vi "TestBoxStart.vi"() -> ()   [LabVIEW 2019]
uses:
  QCtests/general_VIs/globals/QC_MeasurementSetup.vi
  InstrControl/InstrumentSetup.vi
  <instrlib>/ke7002/KE7002.LLB/Keith 7002 Open/Close Chan.vi
  <instrlib>/Agilent 34401/Public/Data/Read (Single Point).vi
  <vilib>/regexp/Match Regular Expression.xnode
  InstrControl/SupplyControl/SupplyControl.lvclass
  InstrControl/LCRControl/LCRControl.lvclass
  InstrControl/InstrControl.lvclass
  InstrControl/ArduinoControl/ArduinoControl.lvclass
  <instrlib>/Agilent 34401/Agilent 34401.lvlib
panel:
  out "Data Path":path
  out "Monitor Start \nTime":dbl=10.0 format="%<%I:%M:%S %p>T"
  out "LCS Data":cluster{dbl[], dbl[], dbl[], dbl[], dbl[]}[](array[cluster])
  out "CV Test CH":i32
  out "CV Data":cluster{dbl[], dbl[], dbl[], dbl[], dbl[]}[](array[cluster])
  out "Time":u32[](array[numeric])
  out "Temperature Array":dbl[](array[numeric])
  out "Humidity Array":dbl[](array[numeric])
  out "IV Data":cluster{dbl[], dbl[], dbl[], dbl[], dbl[]}[](array[cluster])
  out "IV Test CH":i32
  out "Run time":u32 format="%<%H:%M:%S>t"
  out "RH [%]":dbl=10.0
  out "Temp. [°C]":dbl=10.0
  in  "Abort Test":bool
  out "TGraph":cluster{u32[], dbl[]}[](graph)
  in  "Test Control":T1(tab)
  in  "SID 7":string
  in  "LCS Test":bool
  in  "CV Test":bool
  in  "IV Test":bool
  out "T/RH":enum16{"Read Arduino"}(ring)
  in  "Institute:":string(combo)="TRIUMF"
  out "Volt:":string="Aglient 34401A"
  out "LCR:":string="WayneKerr 6440B"
  in  "Quit":bool
  in  "Continue":bool
  in  "Mesurement Control":enum32{"IV Setup", "CV Setup", "LCS Setup"}(tab)
  in  "Cofigure IV Test":bool
  in  "IV Breakdown Limit [V]":dbl=-500.0 caption="Breakdown Limit [V]"
  in  "Step Interval [s] IN":i32=10 caption="step interval [s]"
  in  "Step [V] IN":dbl=10.0 caption="step [V]" format="%.1f"
  in  "IV_Final Volts [V] IN":dbl=-700.0 caption="Final volts [V]"
  in  "IV_Initial Volts [V] IN":dbl caption="Initial volts [V]"
  in  "hold steps IN":i32=6 caption="hold steps"
  in  "IV Current Limit [µA]":dbl=1000.0 caption="Current Limit [µA]" min=0.0001 format="%.3f"
  in  "CV Current Limit [µA]":dbl=15.0 caption="Current Limit [µA]" min=0.0001 format="%.3f"
  in  "CV_depletion limit [V] IN":dbl=-300.0 caption="Depletion Limit [V]"
  in  "CV Frequency [Hz] IN":i32=5000 caption="Frequency [Hz]" format="%#.3p"
  in  "CV_step interval [s] IN":i32=16 caption="Step Interval [s]"
  in  "CV step [V] IN":dbl=10.0 caption="Step [V]" format="%.1f"
  in  "CV_Final volts [V] IN":dbl=-500.0 caption="Final Voltage [V]"
  in  "CV Initial volts [V] IN":dbl caption="Initial Voltage [V]"
  in  "Configure CV Test":bool
  in  "LCS Norm. to Temp. [°C]":dbl=22.0 caption="Norm. to Temp. [°C]"
  in  "LCS Step Interval [s] IN":i32 caption="Step Interval [s]"
  in  "Configure LCS Test":bool
  in  "LCS Current Limit [µA]":dbl=1000.0 caption="Current Limit [µA]" min=0.0001 format="%.3f"
  in  "LCS Step Size [V] IN":dbl caption="Step Size [V]"
  in  "LCS Test Volts [V] IN":dbl=-700.0 caption="Test Voltage [V]"
  in  "LCS Test Duration IN":i32=10 caption="Test Length [HH:MM:SS]" format="%<%H:%M:%S>t"
  in  "LCS Measurement Interval [s] IN":i32=10 caption="Measurement Interval [s]"
  out "SMU:":string="Keithley 2410"
  in  "User:":string(combo)="Graham"
  in  "SID 24":string
  in  "SID 23":string
  in  "SID 22":string
  in  "SID 21":string
  in  "SID 20":string
  in  "SID 19":string
  in  "SID 18":string
  in  "SID 17":string
  in  "SID 16":string
  in  "SID 15":string
  in  "SID 14":string
  in  "SID 13":string
  in  "SID 12":string
  in  "SID 11":string
  in  "SID 10":string
  in  "SID 9":string
  in  "SID 8":string
  in  "SID 6":string
  in  "SID 5":string
  in  "SID 4":string
  in  "SID 3":string
  in  "SID 2":string
  in  "SID 1":string
  in  "IV Scales":T2(ring) caption="Plot Scale"
  out "IV Volts":dbl[](array[numeric]) caption="Volts [V]"
  out "IV Current":dbl[](array[numeric]) caption="Current [nA]"
  in  "IV Iscale":enum16{"nanoAmps", "microAmps", "milliAmps"}(ring) caption="Y Axis Scale"
  out "IV Test Channel:":string caption="Test Channel:"
  out "IV step interval [s]":i32=10 caption="step interval [s]"
  out "IV step [V]":dbl=10.0 caption="Step Size [V]" format="%.1f"
  out "IV Final volts [V]":dbl=-700.0 caption="Final Voltage [V]" format="%.1f"
  out "IV Initial volts [V]":dbl caption="Initial Voltage [V]" format="%.1f"
  out "IV hold steps":i32 caption="Hold Steps"
  out "IV STATUS":string
  out "IV Last reading at:":string caption="Last reading at:"
  out "IV Current reading No.":u32
  out "No of steps":u32
  out "IV Bias On/Off:":bool caption="Bias On/Off:"
  out "IV Current Volts:":dbl caption="Current Volts:" format="%.2f"
  out "IV Time Initiated:":string caption="Time Initiated:"
  out "IV Sensor No.:":string caption="Sensor No.:"
  out "IV Graph":cluster{dbl[], dbl[]}[](graph)
  out "CV Graph":cluster{dbl[], dbl[]}[](graph)
  in  "Cscale":enum16{"1/C^2 [1/nF^2]", "nF", "pF"}(ring) caption="Y Axis Scale"
  out "CV Sensor No.:":string caption="Sensor No.:"
  out "CV Time Initiated:":string caption="Time Initiated:"
  out "CV Current Volts:":dbl caption="Current Volts:" format="%.2f"
  out "CV Bias On/Off:":bool caption="Bias On/Off:"
  out "CV No of steps":u32
  out "CV Current reading No.":u32
  out "CV Last reading at:":string caption="Last reading at:"
  out "CV STATUS":string
  out "CV Test Channel:":string caption="Test Channel:"
  in  "CV Scales":T2(ring) caption="Plot Scale"
  out "CV Capacitance":dbl[](array[numeric]) caption="C [pF]"
  out "CV Resistance":dbl[](array[numeric]) caption="R [kOhm]"
  out "CV Volts":dbl[](array[numeric]) caption="V [V]"
  out "Frequency [Hz]":i32=1000 format="%#.3p"
  out "CV step interval [s]":u32=5 caption="Step Interval [s]"
  out "CV step [V]":dbl=10.0 caption="Step Size [V]" format="%.1f"
  out "CV Final volts [V]":dbl=-700.0 caption="Final Voltage [V]" format="%.1f"
  out "CV Initial volts [V]":dbl caption="Initial Voltage [V]" format="%.1f"
  out "Norm. to Temp. [°C]":dbl=20.0
  out "Number of Sensors":i32=10 caption="No. of Sensors"
  out "LCS Measurement Interval":i32=10 caption="Interval [s["
  out "LCS Test Duration":i32=10 caption="Test Length" format="%<%H:%M:%S>t"
  out "LCS Test Volts [V]":dbl=-700.0 caption="Test Voltage [V]"
  out "Time Remaining":u32 format="%<%H:%M:%S>t"
  out "Time Elapsed":u32 format="%<%H:%M:%S>t"
  out "LCS No of steps":u32
  out "LCS Time Initiated:":string caption="Time Initiated:"
  out "LCS Test Channel:":string caption="Test Channel:"
  out "LCS Sensor No.:":string caption="Sensor No.:"
  out "LCS Current reading No.":u32
  out "LCS Last reading at:":string caption="Last reading at:"
  out "LCS Bias On/Off:":bool caption="Bias On/Off:"
  out "LCS Current Volts:":dbl caption="Current Volts:" format="%.2f"
  in  "LCS Scales":T2(ring) caption="Plot Scale"
  in  "LCS Iscale":enum16{"nanoAmps", "microAmps", "milliAmps"}(ring) caption="Y Axis Scale"
  out "LCS Graph":cluster{dbl[], dbl[]}[](graph)
  out "LCS STATUS":string
  in  "Write Comments":bool
  out "Current Text":string
  in  "End Program":bool
  in  "Comment Box":string
  out "Stability":bool[](array[boolean])
  out "CV":bool[](array[boolean])
  out "IV":bool[](array[boolean])
  in  "Channel":u16(ring)=24 items=["CH 1", "CH 2", "CH 3", "CH 4", "CH 5", "CH 6", "CH 7", "CH 8", "CH 9", "CH 10", "CH 11", "CH 12", "CH 13", "CH 14", "CH 15", "CH 16", "CH 17", "CH 18", "CH 19", "CH 20", "CH 21", "CH 22", "CH 23", "CH 24", "none"]
  in  "Test Type":u16(ring)=3 items=["IV", "CV", "Stability", "none"]
  in  "Review Iscale":u16(ring) caption="Y Axis Scale" items=["nanoAmps", "microAmps", "milliAmps"]
  in  "Review Scales":u16(ring) caption="Plot Scale" items=["Lin - Lin", "Log - Lin", "Lin - Log", "Log - log"]
  out "Review Graph":cluster{dbl[], dbl[]}(graph)
  # "Temperature and Humidity Monitor"
  # "TRIUMF Dark Box Tests"
  # "Base Settings"
  # "Channel 1"
  # "Channel 9"
  # "Channel 17"
  # "Serial Number:"
  # "Serial Number:"
  # "Serial Number:"
  # "Channel 2"
  # "Channel 10"
  # "Channel 18"
  # "Serial Number:"
  # "Serial Number:"
  # "Serial Number:"
  # "Channel 3"
  # "Channel 11"
  # "Channel 19"
  # "Serial Number:"
  # "Serial Number:"
  # "Serial Number:"
  # "Channel 4"
  # "Channel 12"
  # "Channel 20"
  # "Serial Number:"
  # "Serial Number:"
  # "Serial Number:"
  # "Channel 5"
  # "Channel 13"
  # "Channel 21"
  # "Hardware Settings"
  # "Serial Number:"
  # "Serial Number:"
  # "Serial Number:"
  # "Channel 6"
  # "Channel 14"
  # "Channel 22"
  # "Serial Number:"
  # "Serial Number:"
  # "Serial Number:"
  # "Channel 7"
  # "Channel 15"
  # "Channel 23"
  # "Serial Number:"
  # "Serial Number:"
  # "Serial Number:"
  # "Channel 8"
  # "Channel 16"
  # "Channel 24"
  # "Serial Number:"
  # "Serial Number:"
  # "Serial Number:"
  # "IV Mesurement\nParameters"
  # "CV Mesurement\nParameters"
  # "LCS Mesurement\nParameters"
  # "IV Test"
  # "DUT Parameters"
  # "IV Test Parameters"
  # "Plot Settings"
  # "Plot Settings"
  # "Current Status"
  # "Last 5 readings:"
  # "n-4"
  # "n-3"
  # "n-2"
  # "n-1"
  # "Rdg No:"
  # "out of"
  # "n"
  # "CV Test"
  # "DUT Parameters"
  # "CV Test Parameters"
  # "Plot Settings"
  # "Plot Settings"
  # "Current Status"
  # "Last 5 Readings:"
  # "n-4"
  # "n-3"
  # "n-2"
  # "n-1"
  # "Rdg No:"
  # "out of"
  # "n"
  # "Leakage Current Stability Test"
  # "DUT Parameters"
  # "LCS Test Parameters"
  # "Plot Settings"
  # "Plot Settings"
  # "Current Status"
  # "Time"
  # "Rdg No:"
  # "out of"
  # "Test Results"
  # "Plot Selection"
  # "CH 1"
  # "CH 2"
  # "CH 3"
  # "CH 4"
  # "CH 5"
  # "CH 6"
  # "CH 7"
  # "CH 8"
  # "Plot Settings"
  # "CH 9"
  # "CH 10"
  # "Plot Settings"
  # "CH 11"
  # "CH 12"
  # "CH 13"
  # "CH 14"
  # "CH 15"
  # "CH 16"
  # "CH 17"
  # "CH 18"
  # "CH 19"
  # "CH 20"
  # "CH 21"
  # "CH 22"
  # "CH 23"
  # "CH 24"
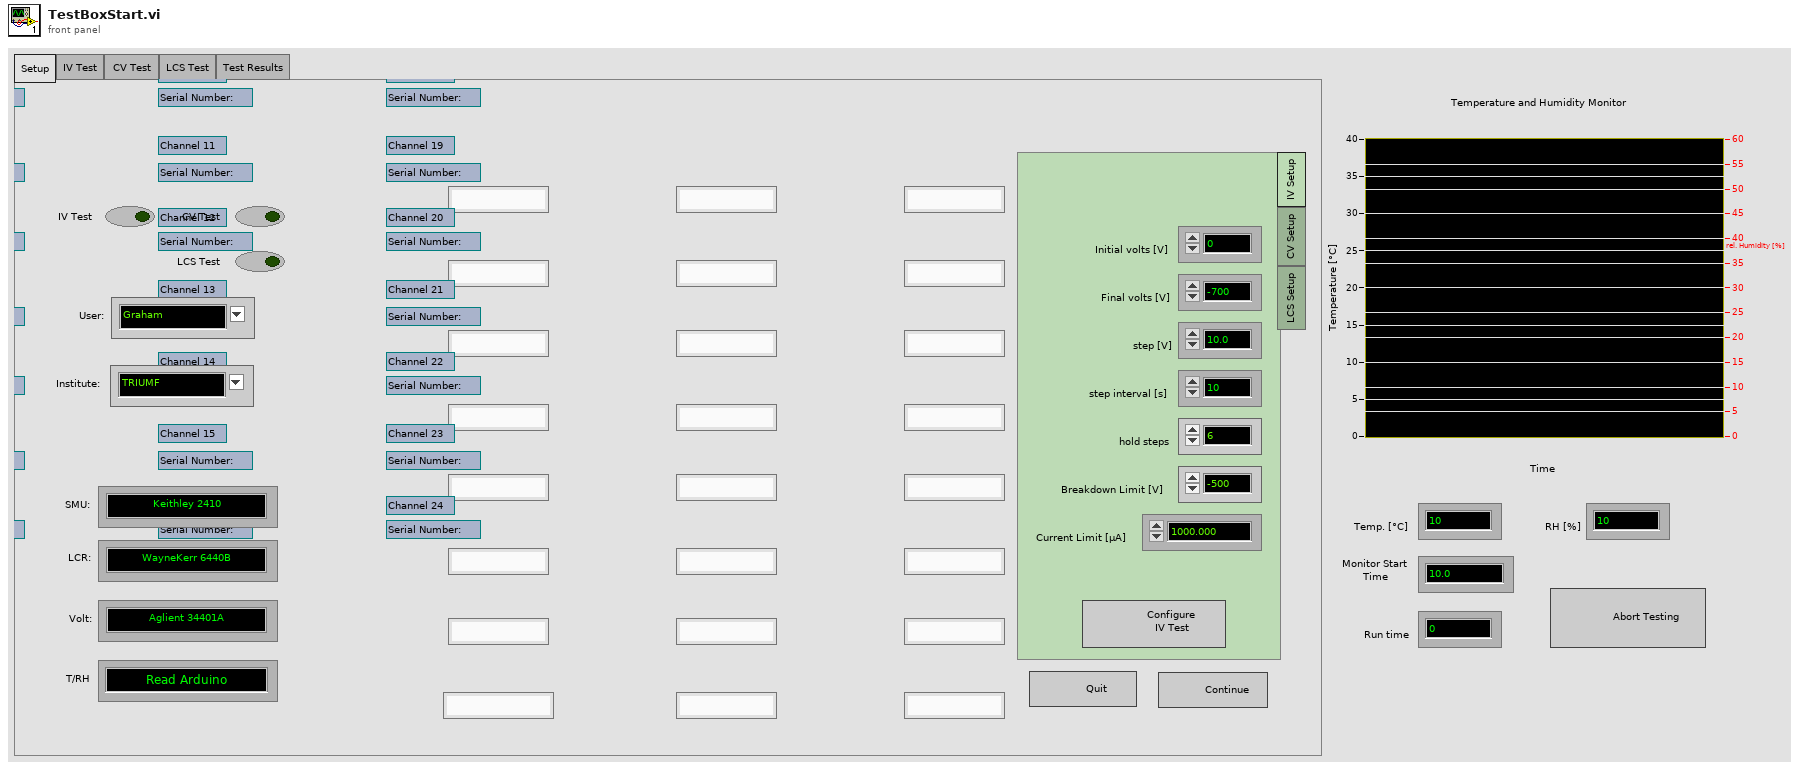
[diagram p1: front panel]
types:
  T1 = enum32{"Setup", "IV Test", "CV Test ", "LCS Test", "Test Results"}
  T2 = enum16{"Lin - Lin", "Log - Lin", "Lin - Log", "Log - log"}
  T3 = enum8{"Enabled", "Disabled", "Disabled and Grayed Out"}
  T4 = enum32{"Setup", "IV Test", "CV Test ", "LCS Test"}
  T5 = enum16{"Supply", "LCR", "Multimeter", "Switching"}
  T6 = enum16{"T/RH", "Interlock", "Edgesense", "Open Switch", "Close Switch", "Reset Switches"}
  T7 = enum32{"IV", "CV", "Stability", "Striptest", "Cis", "Ris", "PTP"}
  T8 = cluster{"Supply":refnum<class "SupplyControl.lvclass">, "Voltage [V]":dbl, "Measurement Interval [s]":i32, "Test Duration":u32, "Ramp up steps [V]":dbl, "Ramp up Interval [s]":u32, "Ramp down steps [V]":dbl, "Ramp down Interval [s]":i32, "Set Current Limit?":bool, "Current Limit [µA]":dbl, "Temperature Readout":enum16{"Read Arduino", "Enter manually"}, "Arduino":refnum<class "ArduinoControl.lvclass">, "Supply Name":string, "Maximum current fluctuation [%]":dbl, "Switching.lvclass":refnum<class "Switching.lvclass">, "Matrix used?":bool, "Matrix X Channels":cluster{"Bias Supply / SMU LO":i32, "Bias Supply / SMU HI":i32, "CV Box LO":i32, "CV Box HI":i32, "CV Box LO IN":i32, "CV Box HI IN":i32, "Volt meter LO":i32, "Volt meter HI":i32, "Mux1 C1":i32, "Mux1 C2":i32, "Mux2 C1":i32, "Mux2 C2":i32}, "LCS Test?":bool, "Number of Steps":i32, "Norm. to Temp.":dbl}
  T9 = cluster{"Supply":refnum<class "SupplyControl.lvclass">, "LCR":refnum<class "LCRControl.lvclass">, "Initial Voltage [V]":dbl, "Final Voltage [V]":dbl, "Step Size [V]":dbl, "Step Interval [s]":i32, "Number Of Steps":u32, "AC frequency [Hz]":i32, "RC Configuration":u16, "AC amplitude [V]":dbl, "Ramp down steps [V]":dbl, "Ramp down Interval [s]":i32, "Set Current Limit?":bool, "Current Limit [µA]":dbl, "Temperature Readout":enum16{"Read Arduino", "Enter manually"}, "Arduino":refnum<class "ArduinoControl.lvclass">, "Supply Name":string, "LCR Name":string, "V_depletion Limit [V]":dbl, "Switching":refnum<class "Switching.lvclass">, "Matrix used?":bool, "Matrix X Channels":cluster{"Bias Supply / SMU LO":i32, "Bias Supply / SMU HI":i32, "CV Box LO":i32, "CV Box HI":i32, "CV Box LO IN":i32, "CV Box HI IN":i32, "Volt meter LO":i32, "Volt meter HI":i32, "Mux1 C1":i32, "Mux1 C2":i32, "Mux2 C1":i32, "Mux2 C2":i32}, "CV Test?":bool}
  T10 = cluster{"Supply":refnum<class "SupplyControl.lvclass">, "Initial Voltage [V]":dbl, "Final Voltage [V]":dbl, "Step Size [V]":dbl, "Step Interval [s]":i32, "Number Of Steps":u32, "Ramp down steps [V]":dbl, "Ramp down Interval [s]":i32, "hold steps":i32, "Set Current Limit?":bool, "Current Limit [µA]":dbl, "Temperature Readout":enum16{"Read Arduino", "Enter manually"}, "Arduino":refnum<class "ArduinoControl.lvclass">, "Supply Name":string, "V_breakdown Limit [V]":dbl, "Switching":refnum<class "Switching.lvclass">, "Matrix used?":bool, "Matrix X Channels":cluster{"Bias Supply / SMU LO":i32, "Bias Supply / SMU HI":i32, "CV Box LO":i32, "CV Box HI":i32, "CV Box LO IN":i32, "CV Box HI IN":i32, "Volt meter LO":i32, "Volt meter HI":i32, "Mux1 C1":i32, "Mux1 C2":i32, "Mux2 C1":i32, "Mux2 C2":i32}, "IV Test?":bool}
  T11 = cluster{"Supply":refnum<class "SupplyControl.lvclass">, "LCR":refnum<class "LCRControl.lvclass">, "Arduino":refnum<class "ArduinoControl.lvclass">, "Switching":refnum<class "Switching.lvclass">, "SMU Name":string, " LCR Name":string, " Volt Name ":string, " Switching GPIB Address ":string, "Temperature Readout":enum16{"Read Arduino", "Enter manually"}, "Voltmeter Visa":refnum<visa-resource-name>}
  T12 = cluster{"User":string, " Institute":string, " Test Time":string, " Test Date":string, "Instruments":string, "Sensor Serials":string[], "IV Test?":bool, "CV Test? ":bool, "LCS Test? ":bool, "No. of Ch.":u16, " Current Sensor":string, " Current Test":string, "Arduino DP Map":string[], "Sensor DB IDs":string[], "Sensor Types":string[], "Data directory":string, "7036 Channel Map":string[], "7054 1 Map":string[], "7054 2 Map ":string[], "7054 3 Map ":string[], "Data Paths":string[][], "IV":bool[], "CV":bool[], "Stability":bool[], "No. of Sensors":i32}
  T13 = cluster{"error":bool, "code":i32, "source":string}
  T14 = cluster{"VISA address":refnum<visa-resource-name>, "T sensor":enum16{"SHT", "DS"}, "Arduino":refnum<class "ArduinoControl.lvclass">}
  T15 = cluster{"slot/memory":i16, "channel/row":i16, "column":i16, bool, bool}[]
  T16 = cluster{"Current Limit":sgl, "KE2410":refnum<class "KE2410.lvclass">}
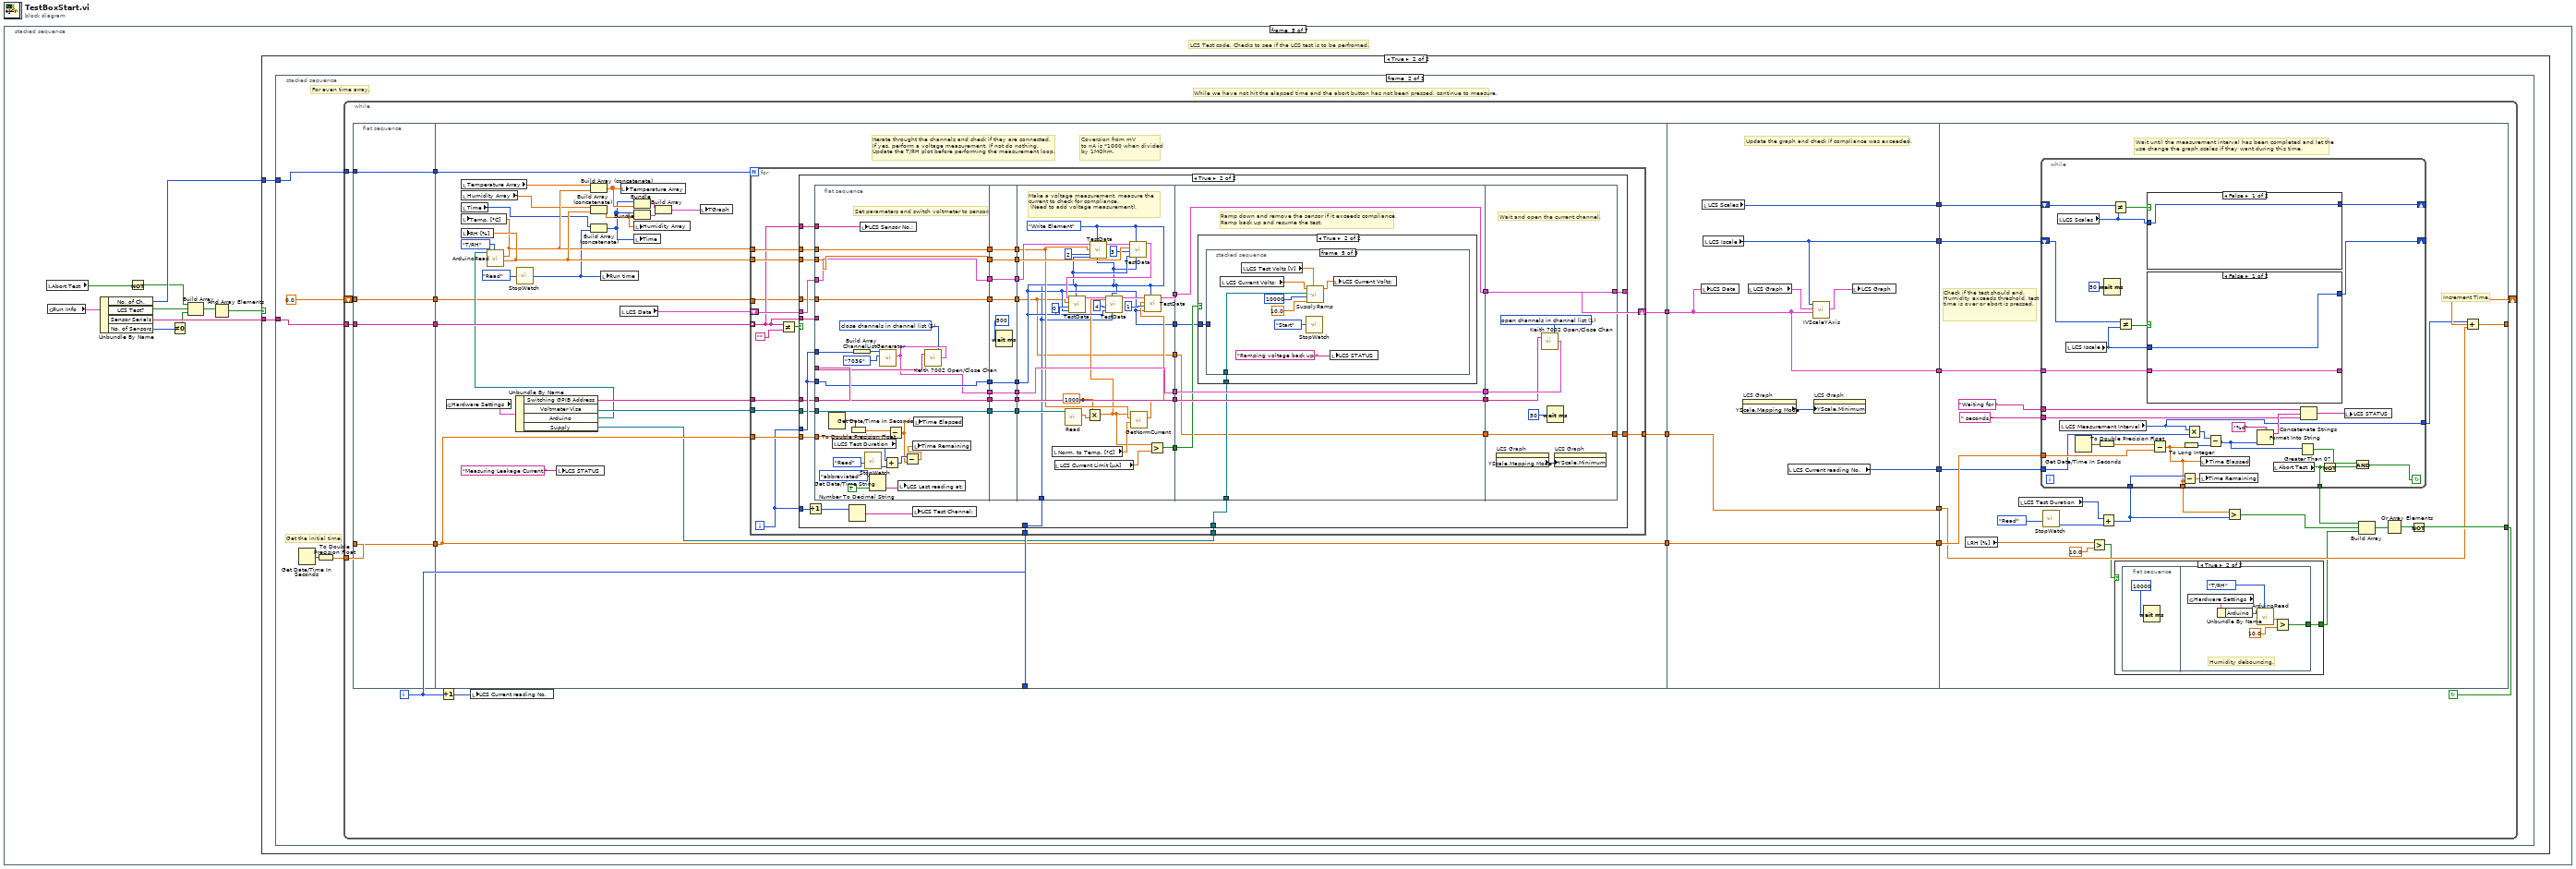
[diagram p0: block diagram]
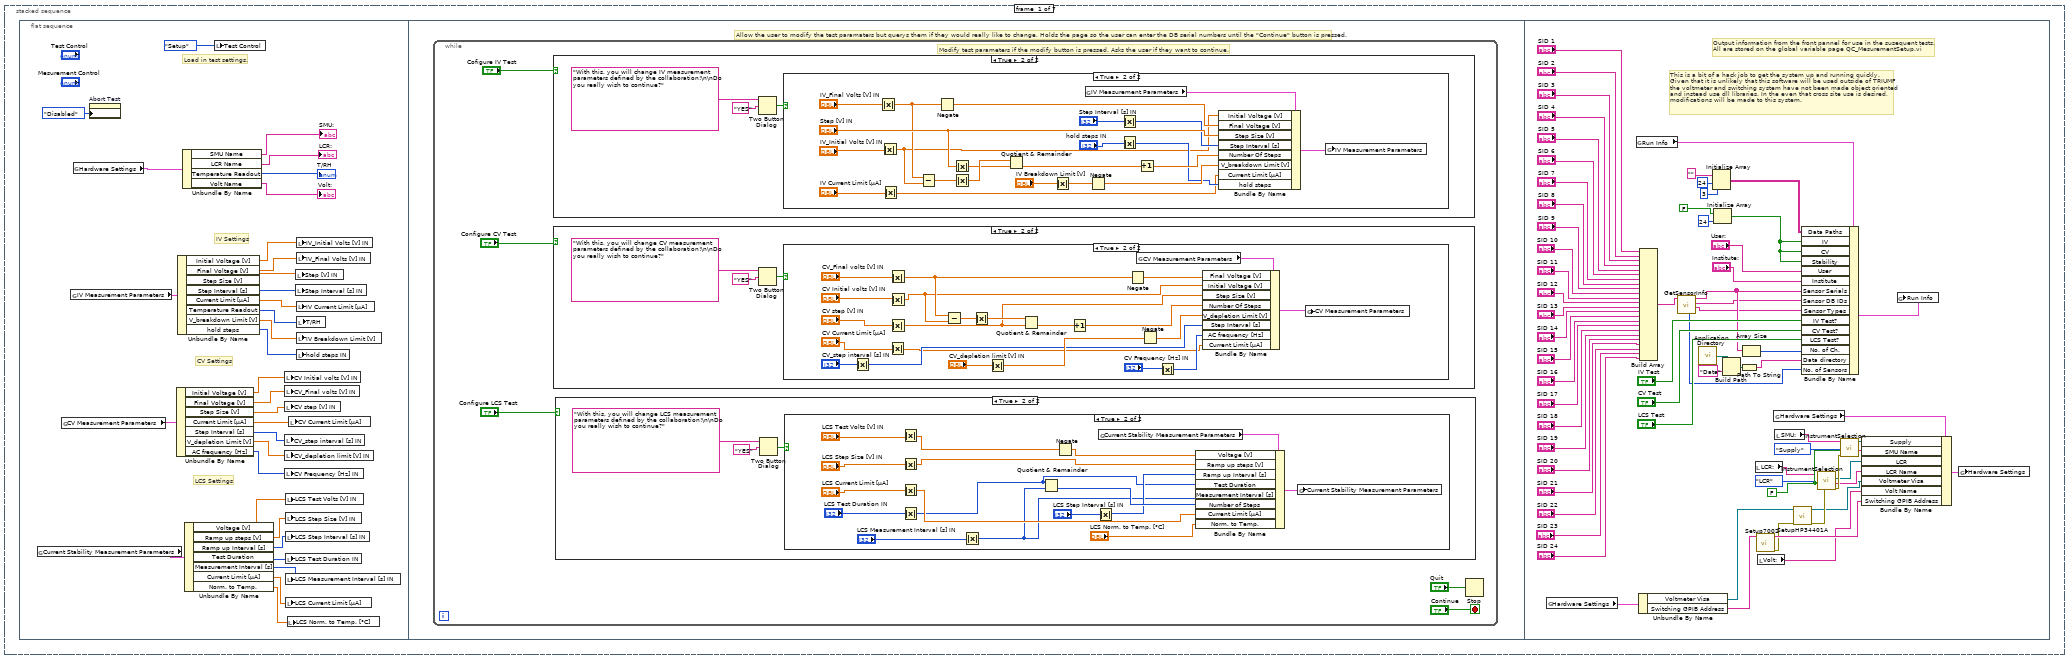
[diagram p2: hidden frame]
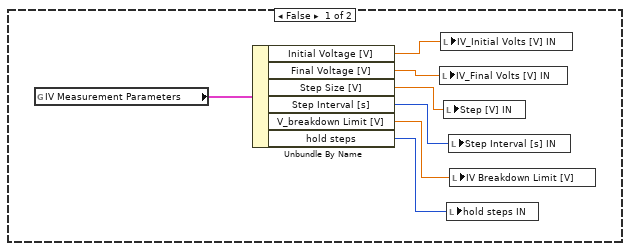
[diagram p8: hidden frame]
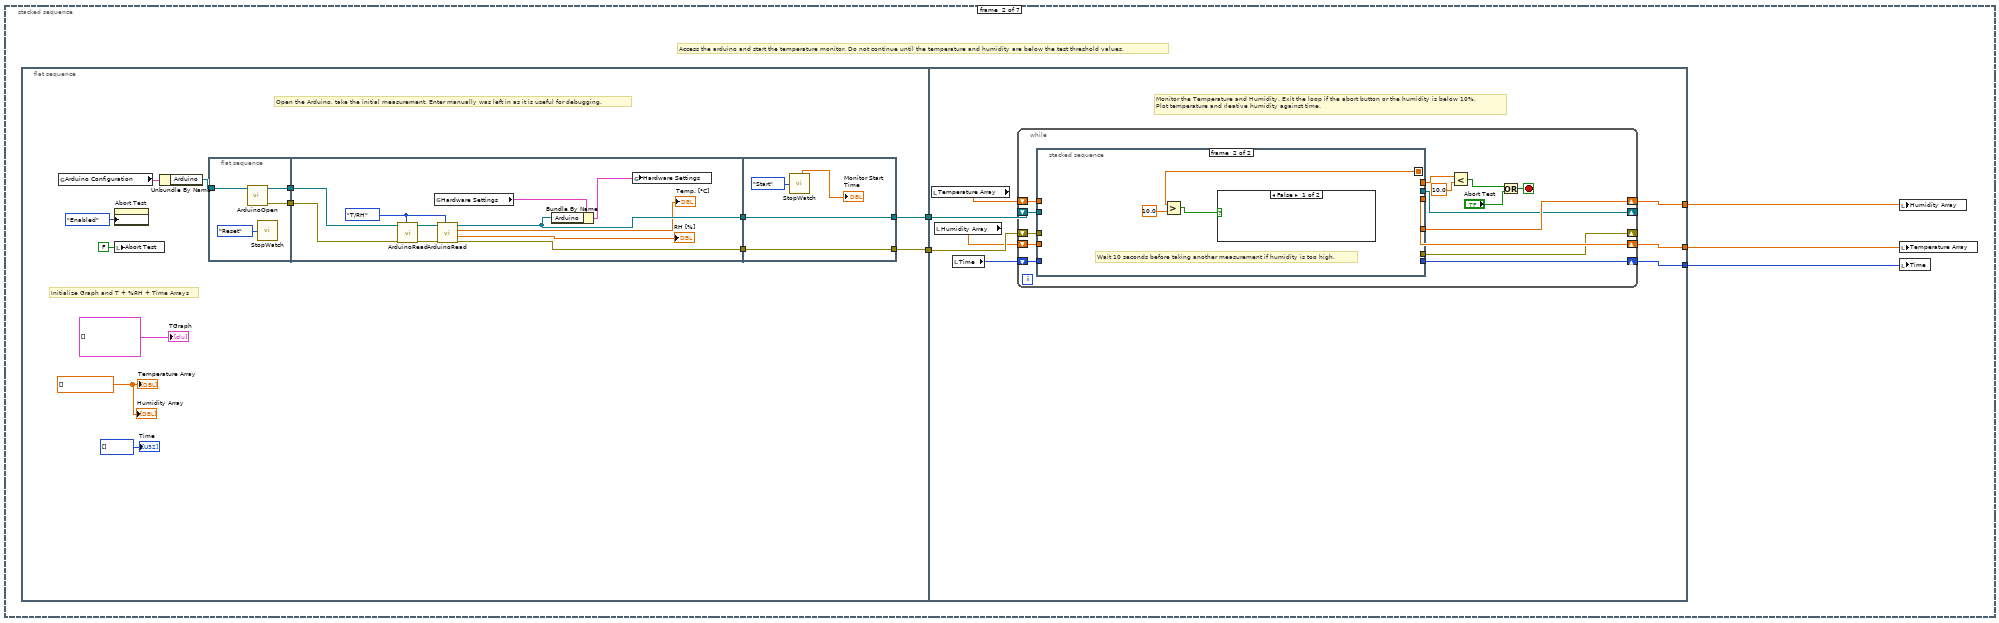
[diagram p9: hidden frame]
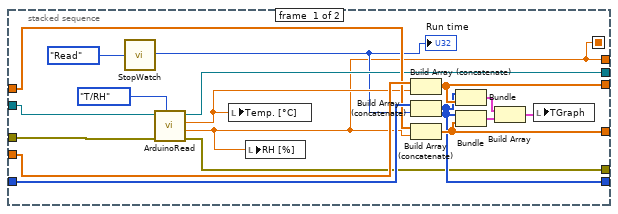
[diagram p10: hidden frame]
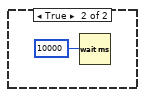
[diagram p11: hidden frame]
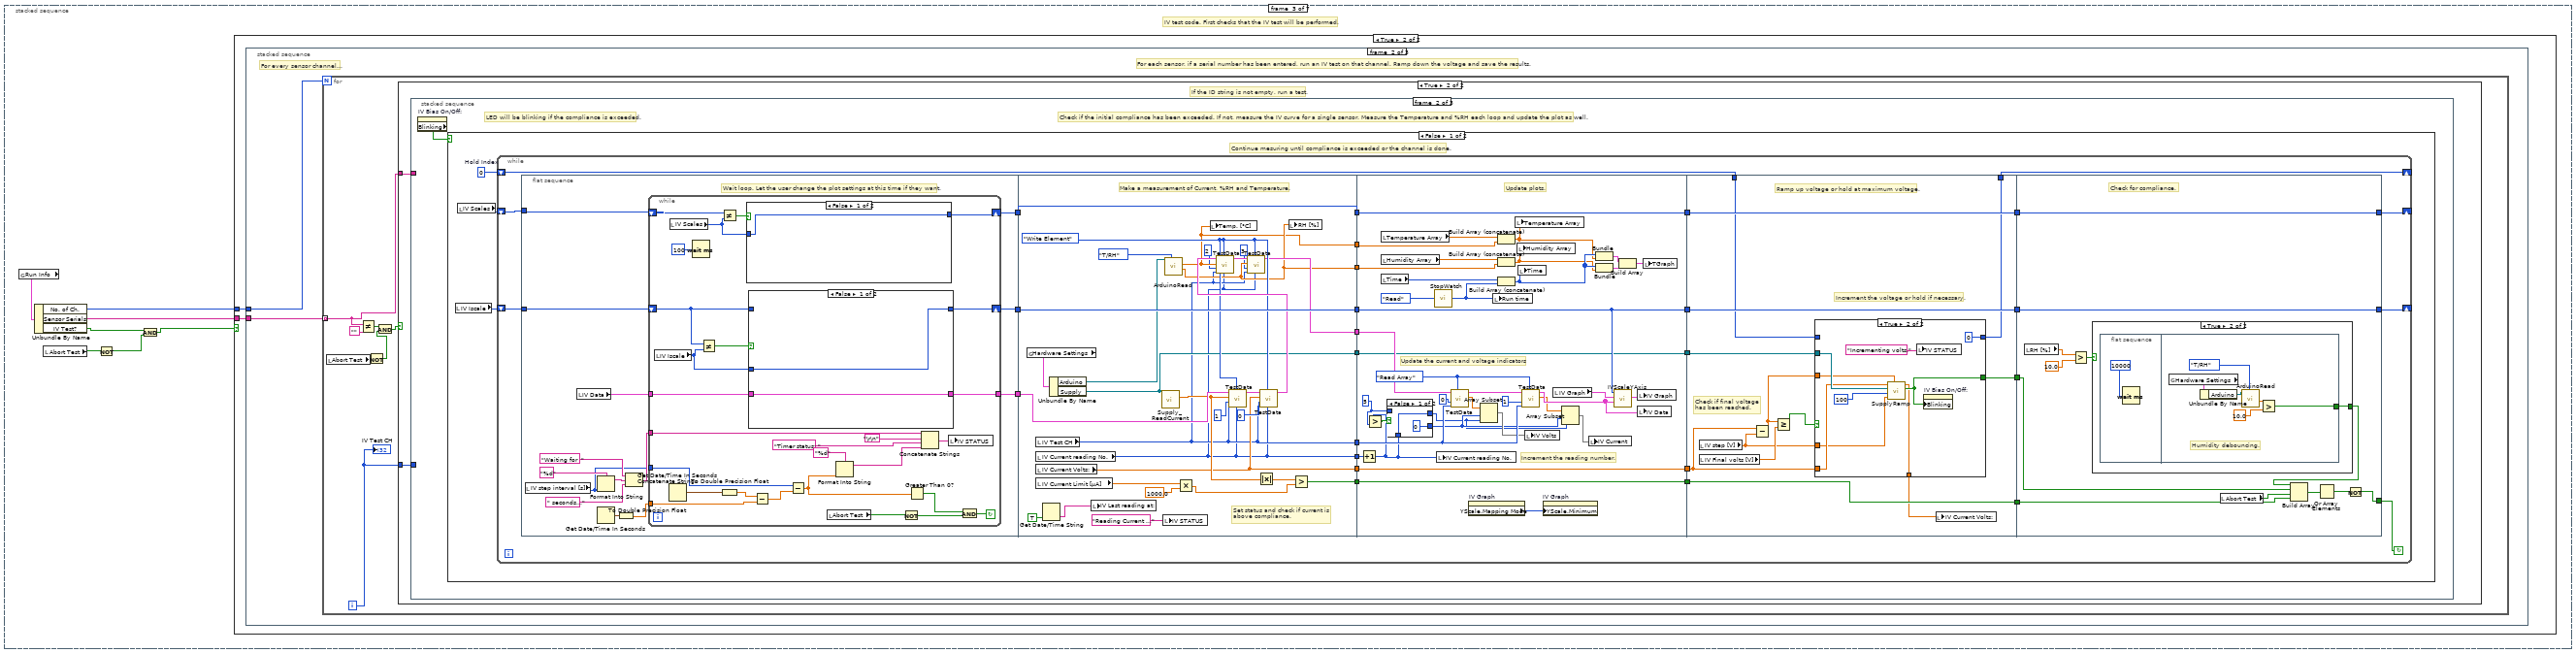
[diagram p12: hidden frame]
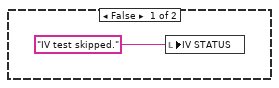
[diagram p13: hidden frame]
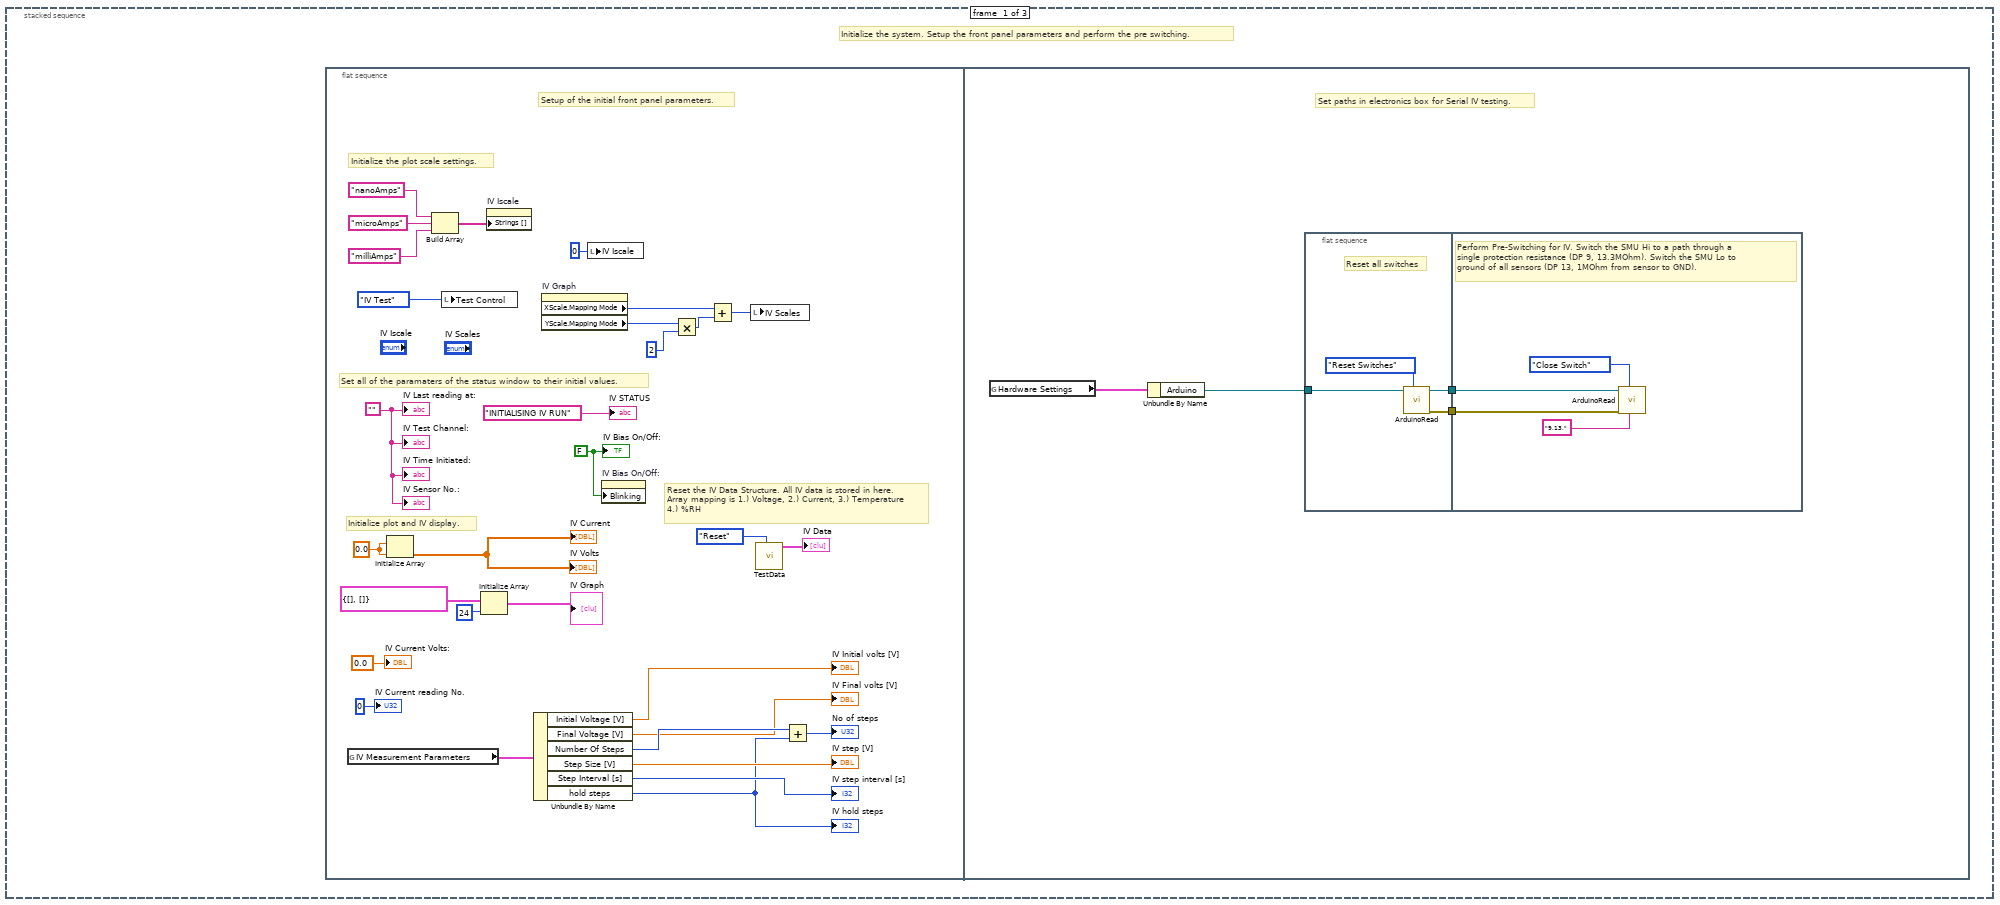
[diagram p14: hidden frame]
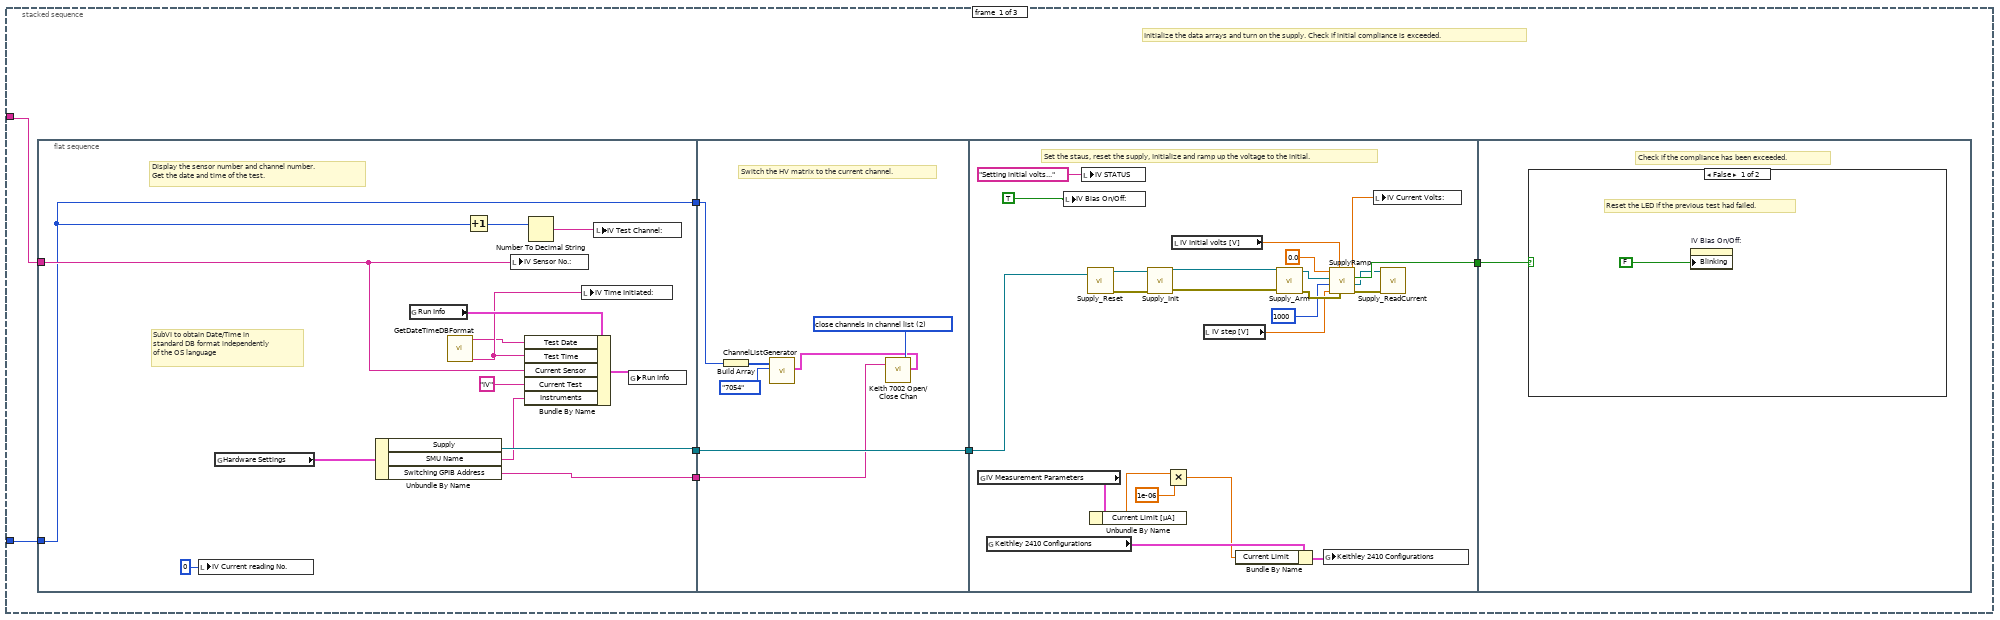
[diagram p16: hidden frame]
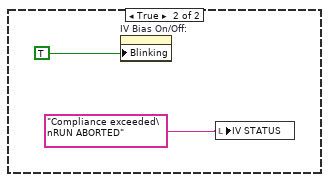
[diagram p17: hidden frame]
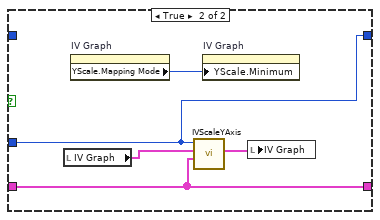
[diagram p18: hidden frame]
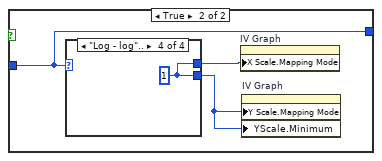
[diagram p19: hidden frame]
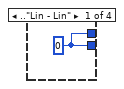
[diagram p20: hidden frame]
diagram:
  n1 = stacked-sequence {
    frame #0 {
      n2 = flat-sequence {
        frame #0 {
          # "LCS Settings"
          # "CV Settings"
          # "IV Settings"
          # "Load in test settings."
          n3 = global read "QC_MeasurementSetup.vi" "Current Stability Measurement Parameters"() -> (w14:T8)
          n4 = global read "QC_MeasurementSetup.vi" "CV Measurement Parameters"() -> (w22:T9)
          n5 = global read "QC_MeasurementSetup.vi" "IV Measurement Parameters"() -> (w32:T10)
          n6 = global read "QC_MeasurementSetup.vi" "Hardware Settings"() -> (w6:T11)
          n7 = property on="Abort Test" class="Bool (strict)"("DisabledEnum"=T3."Disabled" ("Disabled")) -> ()  [unwired: 2 in, 2 out]
          n8 = Unbundle By Name(w22) -> ("Initial Voltage [V]"=w21:dbl, "Final Voltage [V]"=w15:dbl, "Step Size [V]"=w16:dbl, "Current Limit [µA]"=w17:dbl, "Step Interval [s]"=w18:i32, "V_depletion Limit [V]"=w19:dbl, "AC frequency [Hz]"=w20:i32)
          n9 = Unbundle By Name(w32) -> ("Initial Voltage [V]"=w27:dbl, "Final Voltage [V]"=w26:dbl, "Step Size [V]"=w25:dbl, "Step Interval [s]"=w30:i32, "Current Limit [µA]"=w29:dbl, "Temperature Readout"=w28:enum16{"Read Arduino", "Enter manually"}, "V_breakdown Limit [V]"=w24:dbl, "hold steps"=w31:i32)
          n10 = Unbundle By Name(w6) -> ("SMU Name"=→"SMU:":string, "LCR Name"=→"LCR:":string, "Temperature Readout"=→"T/RH":enum16{"Read Arduino", "Enter manually"}, "Volt Name"=→"Volt:":string)
          n11 = Unbundle By Name(w14) -> ("Voltage [V]"=w13:dbl, "Ramp up steps [V]"=w12:dbl, "Ramp up Interval [s]"=w11:u32, "Test Duration"=w10:u32, "Measurement Interval [s]"=w9:i32, "Current Limit [µA]"=w8:dbl, "Norm. to Temp."=w7:dbl)
          n12 = local write "Test Control"(T4."Setup" ("Test Control")) -> ()
          n13 = local write "CV Initial volts [V] IN"(w21) -> ()
          n14 = local write "CV_Final volts [V] IN"(w15) -> ()
          n15 = local write "CV step [V] IN"(w16) -> ()
          n16 = local write "CV_step interval [s] IN"(w18) -> ()
          n17 = local write "CV_depletion limit [V] IN"(w19) -> ()
          n18 = local write "CV Frequency [Hz] IN"(w20) -> ()
          n19 = local write "LCS Test Volts [V] IN"(w13) -> ()
          n20 = local write "LCS Step Size [V] IN"(w12) -> ()
          n21 = local write "LCS Step Interval [s] IN"(w11) -> ()
          n22 = local write "LCS Test Duration IN"(w10) -> ()
          n23 = local write "LCS Measurement Interval [s] IN"(w9) -> ()
          n24 = local write "LCS Current Limit [µA]"(w8) -> ()
          n25 = local write "LCS Norm. to Temp. [°C]"(w7) -> ()
          n26 = local write "CV Current Limit [µA]"(w17) -> ()
          n27 = local write "Step [V] IN"(w25) -> ()
          n28 = local write "Step Interval [s] IN"(w30) -> ()
          n29 = local write "IV_Initial Volts [V] IN"(w27) -> ()
          n30 = local write "IV_Final Volts [V] IN"(w26) -> ()
          n31 = local write "IV Current Limit [µA]"(w29) -> ()
          n32 = local write "IV Breakdown Limit [V]"(w24) -> ()
          n33 = local write "hold steps IN"(w31) -> ()
          n34 = local write "T/RH"(w28) -> ()
        }
        frame #1 {
          # "Allow the user to modify the test paramaters but querys them if they would really like to change. Holds the page so the user can enter the DB serial numbers until the \"Continue\" button is pressed."
          n35 = while {
            stop <- "Continue" stop-if-true
            # "Modify test parameters if the modify button is pressed. Asks the user if they want to continue."
            n36 = case shown="True" "Cofigure IV Test" {
              frame False {
              }
              frame True {
                n37 = Two Button Dialog(message="With this, you will change IV measurement parameters defined by the collaboration!\n\nDo you really wish to continue?", 2:"YES") -> (T button?=w83:bool)  [unwired: 1 in]
                n38 = case shown="True" w83 {
                  frame False {
                    n39 = global read "QC_MeasurementSetup.vi" "IV Measurement Parameters"() -> (w92:T10)
                    n40 = Unbundle By Name(w92) -> ("Initial Voltage [V]"=w90:dbl, "Final Voltage [V]"=w91:dbl, "Step Size [V]"=w89:dbl, "Step Interval [s]"=w88:i32, "V_breakdown Limit [V]"=w87:dbl, "hold steps"=w86:i32)
                    n41 = local write "IV_Final Volts [V] IN"(w91) -> ()
                    n42 = local write "IV_Initial Volts [V] IN"(w90) -> ()
                    n43 = local write "Step [V] IN"(w89) -> ()
                    n44 = local write "hold steps IN"(w86) -> ()
                    n45 = local write "Step Interval [s] IN"(w88) -> ()
                    n46 = local write "IV Breakdown Limit [V]"(w87) -> ()
                  }
                  frame True {
                    n47 = Absolute Value(x="IV_Final Volts [V] IN") -> (abs(x)=w103:dbl)
                    n48 = Absolute Value(x="IV_Initial Volts [V] IN") -> (abs(x)=w93:dbl)
                    n49 = Absolute Value(x="IV Current Limit [µA]") -> (abs(x)=w94:dbl)
                    n50 = Subtract(x=w103, y=w93) -> (x-y=w110:dbl)
                    n51 = Negate(x=w103) -> (-x=w105:dbl)
                    n52 = Absolute Value(x="Step [V] IN") -> (abs(x)=w111:dbl)
                    n53 = Absolute Value(x=w110) -> (abs(x)=w112:dbl)
                    n54 = Quotient & Remainder(x=w112, y=w111) -> (floor(x/y)=w108:dbl)  [unwired: 1 out]
                    n55 = Absolute Value(x="IV Breakdown Limit [V]") -> (abs(x)=w101:dbl)
                    n56 = global read "QC_MeasurementSetup.vi" "IV Measurement Parameters"() -> (w114:T10)
                    n57 = Negate(x=w101) -> (-x=w100:dbl)
                    n58 = Absolute Value(x="Step Interval [s] IN") -> (abs(x)=w98:i32)
                    n59 = Absolute Value(x="hold steps IN") -> (abs(x)=w96:i32)
                    n60 = Increment(x=w108) -> (x+1=w107:dbl)
                    n61 = Bundle By Name(cluster=w114, "Initial Voltage [V]"=w93, "Final Voltage [V]"=w105, "Step Size [V]"="Step [V] IN", "Step Interval [s]"=w98, "Number Of Steps"=w107, "V_breakdown Limit [V]"=w100, "Current Limit [µA]"=w94, "hold steps"=w96) -> (w113:T10)
                    n62 = global write "QC_MeasurementSetup.vi" "IV Measurement Parameters"(w113) -> ()
                  }
                }
              }
            }
            n63 = case shown="True" "Configure CV Test" {
              frame False {
              }
              frame True {
                n64 = Two Button Dialog(message="With this, you will change CV measurement parameters defined by the collaboration!\n\nDo you really wish to continue?", 2:"YES") -> (T button?=w58:bool)  [unwired: 1 in]
                n65 = case shown="True" w58 {
                  frame False {
                  }
                  frame True {
                    n66 = Absolute Value(x="CV_step interval [s] IN") -> (abs(x)=w64:i32)
                    n67 = Absolute Value(x="CV Current Limit [µA]") -> (abs(x)=w62:dbl)
                    n68 = Absolute Value(x="CV_Final volts [V] IN") -> (abs(x)=w72:dbl)
                    n69 = Absolute Value(x="CV Initial volts [V] IN") -> (abs(x)=w61:dbl)
                    n70 = Absolute Value(x="CV step [V] IN") -> (abs(x)=w63:dbl)
                    n71 = Subtract(x=w72, y=w61) -> (x-y=w71:dbl)
                    n72 = Absolute Value(x=w71) -> (abs(x)=w70:dbl)
                    n73 = Absolute Value(x="CV_depletion limit [V] IN") -> (abs(x)=w66:dbl)
                    n74 = Quotient & Remainder(x=w70, y=w63) -> (floor(x/y)=w69:dbl)  [unwired: 1 out]
                    n75 = Increment(x=w69) -> (x+1=w67:dbl)
                    n76 = Negate(x=w72) -> (-x=w79:dbl)
                    n77 = global read "QC_MeasurementSetup.vi" "CV Measurement Parameters"() -> (w82:T9)
                    n78 = Negate(x=w66) -> (-x=w65:dbl)
                    n79 = Absolute Value(x="CV Frequency [Hz] IN") -> (abs(x)=w73:i32)
                    n80 = Bundle By Name(cluster=w82, "Final Voltage [V]"=w79, "Initial Voltage [V]"=w61, "Step Size [V]"=w63, "Number Of Steps"=w67, "V_depletion Limit [V]"=w65, "Step Interval [s]"=w64, "AC frequency [Hz]"=w73, "Current Limit [µA]"=w62) -> (w81:T9)
                    n81 = global write "QC_MeasurementSetup.vi" "CV Measurement Parameters"(w81) -> ()
                  }
                }
              }
            }
            n82 = case shown="True" "Configure LCS Test" {
              frame False {
              }
              frame True {
                n83 = Two Button Dialog(message="With this, you will change LCS measurement parameters defined by the collaboration!\n\nDo you really wish to continue?", 2:"YES") -> (T button?=w38:bool)  [unwired: 1 in]
                n84 = case shown="True" w38 {
                  frame False {
                  }
                  frame True {
                    n85 = Absolute Value(x="LCS Test Volts [V] IN") -> (abs(x)=w52:dbl)
                    n86 = Absolute Value(x="LCS Step Size [V] IN") -> (abs(x)=w48:dbl)
                    n87 = Absolute Value(x="LCS Current Limit [µA]") -> (abs(x)=w47:dbl)
                    n88 = Absolute Value(x="LCS Test Duration IN") -> (abs(x)=w43:i32)
                    n89 = Absolute Value(x="LCS Measurement Interval [s] IN") -> (abs(x)=w44:i32)
                    n90 = Quotient & Remainder(x=w43, y=w44) -> (floor(x/y)=w54:i32)  [unwired: 1 out]
                    n91 = Negate(x=w52) -> (-x=w51:dbl)
                    n92 = Absolute Value(x="LCS Step Interval [s] IN") -> (abs(x)=w53:i32)
                    n93 = global read "QC_MeasurementSetup.vi" "Current Stability Measurement Parameters"() -> (w56:T8)
                    n94 = Bundle By Name(cluster=w56, "Voltage [V]"=w51, "Ramp up steps [V]"=w48, "Ramp up Interval [s]"=w53, "Test Duration"=w43, "Measurement Interval [s]"=w44, "Number of Steps"=w54, "Current Limit [µA]"=w47, "Norm. to Temp."="LCS Norm. to Temp. [°C]") -> (w57:T8)
                    n95 = global write "QC_MeasurementSetup.vi" "Current Stability Measurement Parameters"(w57) -> ()
                  }
                }
              }
            }
            n96 = Stop(stop? (T)="Quit") -> ()
          }
        }
        frame #2 {
          w138 = FALSE
          # "This is a bit of a hack job to get the system up and running quickly.\nGiven that it is unlikely that this software will be used outside of TRIUMF\nthe voltmeter and switching system have not been made object oriented\nand instead use dll libraries. In the even that cross site use is desired, \nmodifications will be made to this system."
          # "Output information from the front pannel for use in the susequent tests.\nAll are stored on the global variable page QC_MesurementSetup.vi"
          n97 = global read "QC_MeasurementSetup.vi" "Hardware Settings"() -> (w153:T11)
          n98 = global read "QC_MeasurementSetup.vi" "Run Info"() -> (w125:T12)
          n99 = Unbundle By Name(w153) -> ("Voltmeter Visa"=w151:refnum<visa-resource-name>, "Switching GPIB Address"=w152:string)
          n100 = Build Array("SID 1", "SID 2", "SID 3", "SID 4", "SID 5", "SID 6", "SID 7", "SID 8", "SID 9", "SID 10", "SID 11", "SID 12", "SID 13", "SID 14", "SID 15", "SID 16", "SID 17", "SID 18", "SID 19", "SID 20", "SID 21", "SID 22", "SID 23", "SID 24") -> (w149:string[])
          n101 = call "GetSensorInfo.vi"("Sensor Serials IN"=w149) -> ("Sensor Types"=w147:string[], "Sensor DB IDs"=w148:string[], "Sensor Serials OUT"=w150:string[], "No. of Sensors"=w115:i32)  [unwired: 6 in, 1 out]
          n102 = call <vilib>:"Application Directory.vi"() -> ("Application Directory"=w146:path)
          n103 = Initialize Array("", 24 ("dimension size"), 3 ("dimension size")) -> (w121:string[][])
          n104 = Initialize Array(FALSE, 24 ("dimension size")) -> (w122:bool[])
          n105 = Build Path(base path=w146, name or relative path="Data") -> (appended path=w144:path)
          n106 = Path To String(path=w144) -> (string=w143:string)
          n107 = Array Size(array=w150) -> (size(s)=w154:i32)
          n108 = local read "LCR:"() -> (w128:string)
          n109 = call "Setup7002.vi"("GPIB IN"=w152) -> ("error out"=w131:T13, "GPIB OUT"=w132:string)  [unwired: 9 in]
          n110 = local read "Volt:"() -> (w126:string)
          n111 = global read "QC_MeasurementSetup.vi" "Hardware Settings"() -> (w142:T11)
          n112 = local read "SMU:"() -> (w127:string)
          n113 = call "SetupHP34401A.vi"("error in (no error)"=w131, "VISA resource name"=w151) -> ("error out"=w130:errorcluster, "VISA resource name out"=w129:refnum<visa-resource-name>)  [unwired: 8 in]
          n114 = Bundle By Name(cluster=w125, "Data Paths"=w121, "IV"=w122, "CV"=w122, "Stability"=w122, "User"="User:", "Institute"="Institute:", "Sensor Serials"=w150, "Sensor DB IDs"=w148, "Sensor Types"=w147, "IV Test?"="IV Test", "CV Test?"="CV Test", "LCS Test?"="LCS Test", "No. of Ch."=w154, "Data directory"=w143, "No. of Sensors"=w115) -> (w160:T12)
          n115 = call "InstrumentSelection.vi"("error in (no error)"=w130, "Verify GPIB address"=w138, "Instrument type"=T5."LCR", "Instrument name IN"=w128) -> ("error out"=w139:errorcluster, "Instrument name OUT"=w134:string, "LCR"=w135:refnum<class "LCRControl.lvclass">)  [unwired: 2 in, 3 out]
          n116 = call "InstrumentSelection.vi"("error in (no error)"=w139, "Verify GPIB address"=w138, "Instrument type"=T5."Supply", "Instrument name IN"=w127) -> ("Instrument name OUT"=w141:string, "Supply"=w140:refnum<class "SupplyControl.lvclass">)  [unwired: 2 in, 4 out]
          n117 = Bundle By Name(cluster=w142, "Supply"=w140, "SMU Name"=w141, "LCR"=w135, "LCR Name"=w134, "Voltmeter Visa"=w129, "Volt Name"=w126, "Switching GPIB Address"=w132) -> (w133:T11)
          n118 = global write "QC_MeasurementSetup.vi" "Run Info"(w160) -> ()
          n119 = global write "QC_MeasurementSetup.vi" "Hardware Settings"(w133) -> ()
        }
      }
    }
    frame #1 {
      # "Access the arduino and start the temperature monitor. Do not continue until the temperature and humidity are below the test threshold values."
      n120 = flat-sequence {
        tunnel: [w198] -> w187
        tunnel: [w195] -> w186
        tunnel: w187 -> [w227]
        tunnel: w186 -> [w226]
        tunnel: [w225] -> w185
        tunnel: [w224] -> w183
        tunnel: [w223] -> w184
        frame #0 {
          w189 = dbl[] [] ("Temperature Array")
          # "Initialize Graph and T + %RH + Time Arrays"
          # "Open the Arduino, take the initial measurement. Enter manually was left in as it is useful for debugging."
          n121 = global read "InstrumentSetup.vi" "Arduino Configuration"() -> (w197:T14)
          n122 = property on="Abort Test" class="Bool (strict)"("DisabledEnum"=T3."Enabled" ("Disabled")) -> ()  [unwired: 2 in, 2 out]
          n123 = local write "Abort Test"(FALSE ("Abort Test")) -> ()
          n124 = Unbundle By Name(w197) -> ("Arduino"=w196:refnum<class "ArduinoControl.lvclass">)
          n125 = flat-sequence {
            tunnel: [w202] -> w200
            tunnel: [w204] -> w199
            tunnel: w196 -> [w203]
            tunnel: w200 -> [w213]
            tunnel: w199 -> [w212]
            tunnel: [w208] -> w194
            tunnel: [w207] -> w193
            tunnel: [w218] -> w195
            tunnel: [w219] -> w198
            tunnel: w194 -> [w219]
            tunnel: w193 -> [w218]
            frame #0 {
              n126 = call "ArduinoOpen.vi"("ArduinoControl in"=w203) -> ("error out"=w204:errorcluster, "ArduinoControl out"=w202:refnum<class "ArduinoControl.lvclass">)  [unwired: 9 in]
              n127 = call "StopWatch.vi"("Action"=enum16{"Start", "Stop", "Read", "Reset"}."Reset") -> ()  [unwired: 5 out]
            }
            frame #1 {
              w209 = enum16{"T/RH", "Interlock", "Edgesense"}."T/RH" ("Arduino function")
              n128 = call "ArduinoRead.vi"("Arduino function"=w209, "error in (no error)"=w212, "ArduinoControl in"=w213) -> ("error out"=w211:errorcluster, "ArduinoControl out"=w210:refnum<class "ArduinoControl.lvclass">)  [unwired: 3 in, 4 out]
              n129 = global read "QC_MeasurementSetup.vi" "Hardware Settings"() -> (w215:T11)
              n130 = call "ArduinoRead.vi"("Arduino function"=w209, "error in (no error)"=w211, "ArduinoControl in"=w210) -> ("error out"=w207:errorcluster, "rel. Humidity [%]"=→"RH [%]":dbl, "Temperature [°C]"=→"Temp. [°C]":dbl, "ArduinoControl out"=w208:refnum<class "ArduinoControl.lvclass">)  [unwired: 3 in, 2 out]
              n131 = Bundle By Name(cluster=w215, "Arduino"=w208) -> (w214:T11)
              n132 = global write "QC_MeasurementSetup.vi" "Hardware Settings"(w214) -> ()
            }
            frame #2 {
              n133 = call "StopWatch.vi"("Action"=enum16{"Start", "Stop", "Read", "Reset"}."Start") -> ("Time started"=→"Monitor Start \nTime":dbl)  [unwired: 4 out]
            }
          }
          "TGraph" <- cluster{u32[], dbl[]}[] [] ("TGraph")
          "Humidity Array" <- w189
          "Temperature Array" <- w189
          "Time" <- u32[] [] ("Time")
        }
        frame #1 {
          # "Monitor the Temperature and Humidity. Exit the loop if the abort button or the humidity is below 10%.\nPlot temperature and rleative humidity against time."
          n134 = local read "Temperature Array"() -> (w222:dbl[])
          n135 = local read "Humidity Array"() -> (w221:dbl[])
          n136 = local read "Time"() -> (w220:u32[])
          n137 = while {
            shift-right: [w240] -> w223
            shift-left: w220 -> [w241]
            shift-right: [w236] -> w224
            shift-left: w221 -> [w239]
            shift-right: [w237] -> w225
            shift-left: w222 -> [w238]
            shift-right: [w234] -> _
            shift-left: w227 -> [w235]
            shift-right: [w232] -> _
            shift-left: w226 -> [w233]
            stop <- w242 stop-if-true
            n138 = stacked-sequence {
              seq-local: [w243 _] -> [_ w263]
              tunnel: w241 -> [w260 _]
              tunnel: [w255 _] -> w240
              tunnel: w239 -> [w259 _]
              tunnel: w238 -> [w258 _]
              tunnel: [w257 _] -> w237
              tunnel: [w256 _] -> w236
              tunnel: w235 -> [w252 _]
              tunnel: [w251 _] -> w234
              tunnel: w233 -> [w250 _]
              tunnel: [w249 _] -> w232
              tunnel: [w243 _] -> w229
              frame #0 {
                n139 = call "StopWatch.vi"("Action"=enum16{"Start", "Stop", "Read", "Reset"}."Read") -> ("Time elapsed"=w245:u32)  [unwired: 4 out]
                "Run time" <- w245
                n140 = call "ArduinoRead.vi"("Arduino function"=enum16{"T/RH", "Interlock", "Edgesense"}."T/RH", "error in (no error)"=w250, "ArduinoControl in"=w252) -> ("error out"=w249:errorcluster, "rel. Humidity [%]"=w243:dbl, "Temperature [°C]"=w246:dbl, "ArduinoControl out"=w251:refnum<class "ArduinoControl.lvclass">)  [unwired: 3 in, 2 out]
                n141 = local write "Temp. [°C]"(w246) -> ()
                n142 = local write "RH [%]"(w243) -> ()
                n143 = Build Array (concatenate)(w259, w246) -> (w256:dbl[])
                n144 = Build Array (concatenate)(w260, w245) -> (w255:u32[])
                n145 = Build Array (concatenate)(w258, w243) -> (w257:dbl[])
                n146 = Bundle(w255, w256) -> (w254:cluster{u32[], dbl[]})  [unwired: 1 in]
                n147 = Bundle(w255, w257) -> (w253:cluster{u32[], dbl[]})  [unwired: 1 in]
                n148 = Build Array(w254, w253) -> (w244:cluster{u32[], dbl[]}[])
                n149 = local write "TGraph"(w244) -> ()
              }
              frame #1 {
                # "Wait 10 seconds before taking another measurement if humidity is too high."
                n150 = Greater?(x=w263, y=10.0) -> (0:w261:bool)
                n151 = case shown="False" w261 {
                  frame False {
                  }
                  frame True {
                    n152 = Wait (ms)(milliseconds to wait=u32 10000) -> ()  [unwired: 1 out]
                  }
                }
              }
            }
            n153 = Less?(x=w229, y=10.0 ("x")) -> (x < y?=w230:bool)
            n154 = Or(x=w230, y="Abort Test") -> (x .or. y?=w242:bool)
          }
        }
      }
      n155 = local write "Humidity Array"(w185) -> ()
      n156 = local write "Temperature Array"(w183) -> ()
      n157 = local write "Time"(w184) -> ()
    }
    frame #2 {
      # "IV test code. First checks that the IV test will be performed."
      n158 = global read "QC_MeasurementSetup.vi" "Run Info"() -> (w271:T12)
      n159 = Unbundle By Name(w271) -> ("No. of Ch."=w269:u16, "Sensor Serials"=w270:string[], "IV Test?"=w265:bool)
      n160 = local read "Abort Test"() -> (w267:bool)
      n161 = Not(x=w267) -> (.not. x?=w266:bool)
      n162 = And(x=w265, y=w266) -> (x .and. y?=w268:bool)
      n163 = case shown="True" w268 {
        tunnel: w270 -> [_ w274]
        tunnel: w269 -> [_ w273]
        frame False {
          n164 = local write "IV STATUS"("IV test skipped." ("IV STATUS")) -> ()
        }
        frame True {
          n165 = stacked-sequence {
            tunnel: w274 -> [_ w319 _]
            tunnel: w273 -> [_ w318 _]
            frame #0 {
              # "Initialize the system. Setup the front panel parameters and perform the pre switching."
              n166 = flat-sequence {
                frame #0 {
                  w281 = ""
                  w291 = 0.0
                  w290 = FALSE ("Visible")
                  # "Reset the IV Data Structure. All IV data is stored in here.\nArray mapping is 1.) Voltage, 2.) Current, 3.) Temperature\n4.) %RH"
                  # "Initialize plot and IV display."
                  # "Setup of the initial front panel parameters."
                  # "Set all of the paramaters of the status window to their initial values."
                  # "Initialize the plot scale settings."
                  n167 = global read "QC_MeasurementSetup.vi" "IV Measurement Parameters"() -> (w302:T10)
                  n168 = Initialize Array(w291, w291) -> (→"IV Volts" →"IV Current":dbl[])
                  n169 = Build Array("nanoAmps", "microAmps", "milliAmps") -> (w293:string[])
                  n170 = local write "Test Control"(T4."IV Test" ("Test Control")) -> ()
                  n171 = Initialize Array(cluster{dbl[], dbl[]} {[], []}, 24 ("dimension size")) -> (→"IV Graph":cluster{dbl[], dbl[]}[])
                  n172 = property on="IV Iscale" class="Enum (strict)"("Strings []"=w293) -> ()  [unwired: 2 in, 2 out]
                  n173 = Unbundle By Name(w302) -> ("Initial Voltage [V]"=→"IV Initial volts [V]":dbl, "Final Voltage [V]"=→"IV Final volts [V]":dbl, "Number Of Steps"=w303:u32, "Step Size [V]"=→"IV step [V]":dbl, "Step Interval [s]"=→"IV step interval [s]":i32, "hold steps"=w280:i32)
                  "IV hold steps" <- w280
                  n174 = property on="IV Graph" class="XYGraph (strict)"() -> ("XScale.Mapping Mode"=w299:u8, "YScale.Mapping Mode"=w300:u8)  [unwired: 2 in, 2 out]
                  n175 = local write "IV Iscale"(u16 0 ("Scale")) -> ()
                  n176 = property on="IV Bias On/Off:" class="Bool (strict)"("Blinking"=w290) -> ()  [unwired: 2 in, 2 out]
                  n177 = Multiply(x=w300, y=2) -> (x*y=w298:i32)
                  n178 = Add(x=w299, y=w298) -> (x+y=w301:i32)
                  n179 = local write "IV Scales"(w301) -> ()
                  n180 = call "TestData.vi"("Action"=enum16{"Reset", "Write Element", "Read Array"}."Reset") -> ("Data OUT"=→"IV Data":cluster{dbl[], dbl[], dbl[], dbl[], dbl[]}[])  [unwired: 9 in, 1 out]
                  n181 = Add(x=w303, y=w280) -> (x+y=→"No of steps":u32)
                  "IV STATUS" <- "INITIALISING IV RUN"
                  "IV Sensor No.:" <- w281
                  "IV Time Initiated:" <- w281
                  "IV Test Channel:" <- w281
                  "IV Bias On/Off:" <- w290
                  "IV Last reading at:" <- w281
                  "IV Current reading No." <- u32 0 ("Current reading No.")
                  "IV Current Volts:" <- 0.0 ("Current Volts:")
                }
                frame #1 {
                  # "Set paths in electronics box for Serial IV testing."
                  n182 = global read "QC_MeasurementSetup.vi" "Hardware Settings"() -> (w309:T11)
                  n183 = Unbundle By Name(w309) -> ("Arduino"=w306:refnum<class "ArduinoControl.lvclass">)
                  n184 = flat-sequence {
                    tunnel: w306 -> [w313]
                    tunnel: [w312] -> w308
                    tunnel: [w311] -> w307
                    tunnel: w308 -> [w317]
                    tunnel: w307 -> [w315]
                    frame #0 {
                      # "Reset all switches"
                      n185 = call "ArduinoRead.vi"("Arduino function"=T6."Reset Switches", "ArduinoControl in"=w313) -> ("error out"=w311:errorcluster, "ArduinoControl out"=w312:refnum<class "ArduinoControl.lvclass">)  [unwired: 4 in, 4 out]
                    }
                    frame #1 {
                      # "Perform Pre-Switching for IV. Switch the SMU Hi to a path through a \nsingle protection resistance (DP 9, 13.3MOhm). Switch the SMU Lo to \nground of all sensors (DP 13, 1MOhm from sensor to GND)."
                      n186 = call "ArduinoRead.vi"("Command String"="9,13,", "Arduino function"=T6."Close Switch", "error in (no error)"=w315, "ArduinoControl in"=w317) -> ()  [unwired: 2 in, 6 out]
                    }
                  }
                }
              }
            }
            frame #1 {
              # "For every sensor channel..."
              # "For each sensor, if a serial number has been entered, run an IV test on that channel. Ramp down the voltage and save the results."
              n187 = for {
                N: w318 -> [_]
                tunnel: w319 -> [w325] mode=indexing
                i -> [w324]
                n188 = local read "Abort Test"() -> (w323:bool)
                n189 = Not Equal?(x=w325, y="") -> (x != y?=w322:bool)
                n190 = Not(x=w323) -> (.not. x?=w321:bool)
                n191 = And(x=w322, y=w321) -> (x .and. y?=w320:bool)
                n192 = case shown="True" w320 {
                  tunnel: w325 -> [_ w327]
                  tunnel: w324 -> [_ w328]
                  frame False {
                    # "If the ID String is empty, do nothing."
                  }
                  frame True {
                    # "If the ID string is not empty, run a test."
                    n193 = stacked-sequence {
                      tunnel: w328 -> [w333 _ w601]
                      tunnel: w327 -> [w329 _ _]
                      frame #0 {
                        # "Initialize the data arrays and turn on the supply. Check if initial compliance is exceeded."
                        n194 = flat-sequence {
                          tunnel: w329 -> [w345]
                          tunnel: [w338] -> w335
                          tunnel: w333 -> [w338]
                          tunnel: [w342] -> w331
                          tunnel: [w340] -> w330
                          tunnel: w335 -> [w350]
                          tunnel: [w356] -> w332
                          tunnel: w331 -> [w356]
                          tunnel: w330 -> [w355]
                          tunnel: [w377] -> w334
                          tunnel: w332 -> [w376]
                          tunnel: w334 -> [w380]
                          frame #0 {
                            # "SubVI to obtain Date/Time in\nstandard DB format independently\nof the OS language"
                            # "Display the sensor number and channel number. \nGet the date and time of the test."
                            n195 = local write "IV Current reading No."(u32 0 ("IV Current reading No.")) -> ()
                            n196 = global read "QC_MeasurementSetup.vi" "Hardware Settings"() -> (w343:T11)
                            n197 = Unbundle By Name(w343) -> ("Supply"=w342:refnum<class "SupplyControl.lvclass">, "SMU Name"=w341:string, "Switching GPIB Address"=w340:string)
                            n198 = global read "QC_MeasurementSetup.vi" "Run Info"() -> (w348:T12)
                            n199 = call "GetDateTimeDBFormat.vi"() -> ("Time in 24h format, e.g. 13:40:54"=w337:string, "Abbreviated Date, e.g. 13 Nov 2020"=w336:string)  [unwired: 10 in]
                            n200 = Increment(x=w338) -> (x+1=w339:i32)
                            n201 = local write "IV Sensor No.:"(w345) -> ()
                            n202 = Bundle By Name(cluster=w348, "Test Date"=w336, "Test Time"=w337, "Current Sensor"=w345, "Current Test"="IV", "Instruments"=w341) -> (w347:T12)
                            n203 = Number To Decimal String(number=w339) -> (decimal integer string=w349:string)  [unwired: 1 in]
                            n204 = local write "IV Time Initiated:"(w337) -> ()
                            n205 = local write "IV Test Channel:"(w349) -> ()
                            n206 = global write "QC_MeasurementSetup.vi" "Run Info"(w347) -> ()
                          }
                          frame #1 {
                            w354 = u16 2 items=["open all channels", "open channels in channel list", "close channels in channel list"] ("open/close (open all:0)")
                            # "Switch the HV matrix to the current channel."
                            n207 = Build Array(w350) -> (w353:i32[])
                            n208 = call "ChannelListGenerator.vi"("Card Type"=enum16{"7036", "7054"}."7054", "Channels"=w353) -> ("Channel List"=w351:T15)  [unwired: 9 in]
                            n209 = call "Keith 7002 Open/Close Chan.vi"("GPIB address"=w355, "open/close (open all:0)"=w354, "channel list"=w351) -> ()  [unwired: 1 in, 1 out]
                          }
                          frame #2 {
                            # "Set the staus, reset the supply, Initialize and ramp up the voltage to the initial."
                            n210 = global read "QC_MeasurementSetup.vi" "IV Measurement Parameters"() -> (w364:T10)
                            n211 = global read "InstrumentSetup.vi" "Keithley 2410 Configurations"() -> (w361:T16)
                            n212 = local write "IV Bias On/Off:"(TRUE ("IV Bias On/Off:")) -> ()
                            n213 = local write "IV STATUS"("Setting initial volts..." ("STATUS 1")) -> ()
                            n214 = call-dynamic "Supply_Reset.vi"("SupplyControl in"=w376) -> ("error out"=w373:errorcluster, "SupplyControl out"=w374:refnum<class "SupplyControl.lvclass">)  [unwired: 9 in]
                            n215 = Unbundle By Name(w364) -> ("Current Limit [µA]"=w362:dbl)
                            n216 = call-dynamic "Supply_Init.vi"("error in (no error)"=w373, "SupplyControl in"=w374) -> ("error out"=w357:errorcluster, "SupplyControl out"=w358:refnum<class "SupplyControl.lvclass">)  [unwired: 8 in]
                            n217 = Multiply(x=w362, y=1e-06) -> (x*y=w359:dbl)
                            n218 = local read "IV Initial volts [V]"() -> (w365:dbl)
                            n219 = local read "IV step [V]"() -> (w366:dbl)
                            n220 = Bundle By Name(cluster=w361, "Current Limit"=w359) -> (w360:T16)
                            n221 = call-dynamic "Supply_Arm.vi"("error in (no error)"=w357, "SupplyControl in"=w358) -> ("error out"=w371:errorcluster, "SupplyControl out"=w372:refnum<class "SupplyControl.lvclass">)  [unwired: 8 in]
                            n222 = global write "InstrumentSetup.vi" "Keithley 2410 Configurations"(w360) -> ()
                            n223 = call "SupplyRamp.vi"("error in"=w371, "Requested Voltage"=w365, "Step Size"=w366, "Step Delay"=1000, "Supply IN"=w372, "Starting Voltage"=0.0) -> ("error out"=w370:errorcluster, "Supply OUT"=w369:refnum<class "SupplyControl.lvclass">, "Compliance exceeded"=w377:bool, "Current Voltage"=w375:dbl)  [unwired: 2 in]
                            n224 = local write "IV Current Volts:"(w375) -> ()
                            n225 = call-dynamic "Supply_ReadCurrent.vi"("error in (no error)"=w370, "SupplyControl in"=w369) -> ()  [unwired: 7 in, 3 out]
                          }
                          frame #3 {
                            # "Check if the compliance has been exceeded."
                            n226 = case shown="False" w380 {
                              frame False {
                                # "Reset the LED if the previous test had failed."
                                n227 = property on="IV Bias On/Off:" class="Bool (strict)"("Blinking"=FALSE) -> ()  [unwired: 2 in, 2 out]
                              }
                              frame True {
                                n228 = property on="IV Bias On/Off:" class="Bool (strict)"("Blinking"=TRUE) -> ()  [unwired: 2 in, 2 out]
                                n229 = local write "IV STATUS"("Compliance exceeded\nRUN ABORTED") -> ()
                              }
                            }
                          }
                        }
                      }
                      frame #1 {
                        # "LED will be blinking if the compliance is exceeded."
                        # "Check if the initial compliance has been exceeded. If not, measure the IV curve for a single sensor. Measure the Temperature and %RH each loop and update the plot as well."
                        n230 = property on="IV Bias On/Off:" class="Bool (strict)"() -> ("Blinking"=w384:bool)  [unwired: 2 in, 2 out]
                        n231 = case shown="False" w384 {
                          frame False {
                            w385 = 0  # Hold Index
                            # "Continue mesuring until compliance is exceeded or the channel is done."
                            n232 = local read "IV Iscale"() -> (w387:enum16{"nanoAmps", "microAmps", "milliAmps"})
                            n233 = local read "IV Scales"() -> (w386:T2)
                            n234 = while {
                              shift-right: [w390] -> _
                              shift-left: w387 -> [w415]
                              shift-right: [w391] -> _
                              shift-left: w386 -> [w416]
                              shift-right: [w392] -> _
                              shift-left: w385 -> [w393]
                              stop <- w388 continue-if-true
                              n235 = flat-sequence {
                                tunnel: w416 -> [w425]
                                tunnel: w415 -> [w424]
                                tunnel: [w420] -> w414
                                tunnel: [w419] -> w413
                                tunnel: [w417] -> w406
                                tunnel: w414 -> [w504]
                                tunnel: w413 -> [w503]
                                tunnel: [w504] -> w412
                                tunnel: [w503] -> w411
                                tunnel: w406 -> [w497]
                                tunnel: [w494] -> w405
                                tunnel: [w488] -> w404
                                tunnel: [w479] -> w403
                                tunnel: [w480] -> w402
                                tunnel: [w487] -> w400
                                tunnel: [w486] -> w399
                                tunnel: [w481] -> w397
                                tunnel: [w485] -> w394
                                tunnel: w412 -> [w542]
                                tunnel: w411 -> [w534]
                                tunnel: [w542] -> w410
                                tunnel: [w534] -> w409
                                tunnel: w405 -> [w539]
                                tunnel: w404 -> [w530]
                                tunnel: w403 -> [w519]
                                tunnel: w402 -> [w537]
                                tunnel: [w530] -> w401
                                tunnel: w400 -> [w529]
                                tunnel: w399 -> [w528]
                                tunnel: w397 -> [w527]
                                tunnel: [w527] -> w396
                                tunnel: [w526] -> w395
                                tunnel: w394 -> [w526]
                                tunnel: w410 -> [w560]
                                tunnel: w409 -> [w559]
                                tunnel: [w560] -> w408
                                tunnel: [w559] -> w407
                                tunnel: w401 -> [w558]
                                tunnel: [w558] -> w398
                                tunnel: w396 -> [w553]
                                tunnel: w395 -> [w555]
                                tunnel: w393 -> [w551]
                                tunnel: [w550] -> w392
                                tunnel: [w549] -> w389
                                tunnel: [w585] -> w390
                                tunnel: [w586] -> w391
                                tunnel: w408 -> [w586]
                                tunnel: w407 -> [w585]
                                tunnel: w398 -> [w580]
                                tunnel: w389 -> [w582]
                                tunnel: [w579] -> w388
                                frame #0 {
                                # "Wait loop. Let the user change the plot settings at this time if they want."
                                n236 = local read "IV step interval [s]"() -> (w421:i32)
                                n237 = local read "IV Data"() -> (w418:cluster{dbl[], dbl[], dbl[], dbl[], dbl[]}[])
                                n238 = Format Into String(format string="%d", w421) -> (resulting string=w428:string)  [unwired: 2 in, 1 out]
                                n239 = Get Date/Time In Seconds() -> (seconds since 1Jan1904=w426:timestamp)
                                n240 = To Double Precision Float(number=w426) -> (double precision float=w423:dbl)
                                n241 = Concatenate Strings("Waiting for  ", w428, " seconds...") -> (w422:string)
                                n242 = while {
                                shift-right: [w454] -> w420
                                shift-left: w425 -> [w456]
                                shift-right: [w453] -> w419
                                shift-left: w424 -> [w452]
                                tunnel: w423 -> [w438]
                                tunnel: w422 -> [w437]
                                tunnel: w421 -> [w434]
                                tunnel: w418 -> [w432]
                                tunnel: [w431] -> w417
                                stop <- w435 continue-if-true
                                n243 = local read "IV Iscale"() -> (w449:enum16{"nanoAmps", "microAmps", "milliAmps"})
                                n244 = Get Date/Time In Seconds() -> (seconds since 1Jan1904=w441:timestamp)
                                n245 = local read "IV Scales"() -> (w455:T2)
                                n246 = Wait (ms)(milliseconds to wait=u32 100) -> ()  [unwired: 1 out]
                                n247 = Not Equal?(x=w452, y=w449) -> (x != y?=w451:bool)
                                n248 = Not Equal?(x=w456, y=w455) -> (x != y?=w457:bool)
                                n249 = To Double Precision Float(number=w441) -> (double precision float=w442:dbl)
                                n250 = case shown="False" w457 {
                                tunnel: w455 -> [w465 w466]
                                tunnel: [w465 w466] -> w454
                                frame False {
                                }
                                frame True {
                                n251 = case shown="\"Log - log\".." w466 {
                                tunnel: [w469 1 0 w474] -> w468
                                tunnel: [w469 0 1 w474] -> w467
                                frame .."Lin - Lin" {
                                w469 = 0
                                }
                                frame "Log - Lin" {
                                }
                                frame "Lin - Log" {
                                }
                                frame "Log - log".. {
                                w474 = 1
                                }
                                }
                                n252 = property on="IV Graph" class="XYGraph (strict)"("X Scale.Mapping Mode"=w468) -> ()  [unwired: 2 in, 2 out]
                                n253 = property on="IV Graph" class="XYGraph (strict)"("Y Scale.Mapping Mode"=w467, "YScale.Minimum"=w467) -> ()  [unwired: 2 in, 2 out]
                                }
                                }
                                n254 = case shown="False" w451 {
                                tunnel: w452 -> [_ _]
                                tunnel: [w458 w460] -> w453
                                tunnel: w449 -> [w458 w460]
                                tunnel: w432 -> [w459 w461]
                                tunnel: [w459 w461] -> w431
                                frame False {
                                }
                                frame True {
                                n255 = local read "IV Graph"() -> (w462:cluster{dbl[], dbl[]}[])
                                n256 = property on="IV Graph" class="XYGraph (strict)"() -> ("YScale.Mapping Mode"=w464:u8)  [unwired: 2 in, 2 out]
                                n257 = call "IVScaleYAxis.vi"("Data IN"=w461, "Plot In"=w462, "Y Scale"=w460) -> ("Plot Out"=w463:cluster{dbl[], dbl[]}[])  [unwired: 8 in]
                                n258 = property on="IV Graph" class="XYGraph (strict)"("YScale.Minimum"=w464) -> ()  [unwired: 2 in, 2 out]
                                n259 = local write "IV Graph"(w463) -> ()
                                }
                                }
                                n260 = Subtract(x=w442, y=w438) -> (x-y=w440:dbl)
                                n261 = Subtract(x=w434, y=w440) -> (x-y=w433:dbl)
                                n262 = local read "Abort Test"() -> (w439:bool)
                                n263 = Format Into String(format string="%d", w433) -> (resulting string=w447:string)  [unwired: 2 in, 1 out]
                                n264 = Not(x=w439) -> (.not. x?=w448:bool)
                                n265 = Greater Than 0?(x=w433) -> (x > 0?=w443:bool)
                                n266 = Concatenate Strings(w437, "\r\n", "Timer status: ", w447) -> (w436:string)
                                n267 = local write "IV STATUS"(w436) -> ()
                                n268 = And(x=w443, y=w448) -> (x .and. y?=w435:bool)
                                }
                                }
                                frame #1 {
                                w495 = enum16{"Reset", "Write Element", "Read Array"}."Write Element" ("Action")
                                # "Set status and check if current is \nabove compliance."
                                # "Make a measurement of Current, %RH and Temperature."
                                n269 = global read "QC_MeasurementSetup.vi" "Hardware Settings"() -> (w499:T11)
                                n270 = local read "IV Test CH"() -> (w480:i32)
                                n271 = local read "IV Current reading No."() -> (w479:u32)
                                n272 = local read "IV Current Volts:"() -> (w481:dbl)
                                n273 = local read "IV Current Limit [µA]"() -> (w491:dbl)
                                n274 = Get Date/Time String(want seconds? (F)=TRUE) -> (time string=w501:string)  [unwired: 2 in, 1 out]
                                n275 = Unbundle By Name(w499) -> ("Arduino"=w498:refnum<class "ArduinoControl.lvclass">, "Supply"=w485:refnum<class "SupplyControl.lvclass">)
                                n276 = local write "IV Last reading at:"(w501) -> ()
                                n277 = call-dynamic "Supply_ReadCurrent.vi"("SupplyControl in"=w485) -> ("Current in nA"=w489:dbl)  [unwired: 8 in, 2 out]
                                n278 = local write "IV STATUS"("Reading Current ..." ("status")) -> ()
                                n279 = call "ArduinoRead.vi"("Arduino function"=T6."T/RH", "ArduinoControl in"=w498) -> ("rel. Humidity [%]"=w487:dbl, "Temperature [°C]"=w486:dbl)  [unwired: 4 in, 4 out]
                                n280 = Multiply(x=w491, y=1000.0) -> (x*y=w490:dbl)
                                n281 = local write "Temp. [°C]"(w486) -> ()
                                n282 = call "TestData.vi"("Reading No."=w479, "Action"=w495, "Test No."=w480, "Array No."=u32 1, 10:"Data IN"=w489, 11:"Data IN"=w497) -> ("Data OUT"=w484:cluster{dbl[], dbl[], dbl[], dbl[], dbl[]}[])  [unwired: 4 in, 1 out]
                                n283 = Absolute Value(x=w489) -> (abs(x)=w493:dbl)
                                n284 = call "TestData.vi"("Reading No."=w479, "Action"=w495, "Test No."=w480, "Array No."=u32 0, 10:"Data IN"=w481, 11:"Data IN"=w484) -> ("Data OUT"=w496:cluster{dbl[], dbl[], dbl[], dbl[], dbl[]}[])  [unwired: 4 in, 1 out]
                                n285 = call "TestData.vi"("Reading No."=w479, "Action"=w495, "Test No."=w480, "Array No."=u32 2, 10:"Data IN"=w486, 11:"Data IN"=w496) -> ("Data OUT"=w478:cluster{dbl[], dbl[], dbl[], dbl[], dbl[]}[])  [unwired: 4 in, 1 out]
                                n286 = call "TestData.vi"("Reading No."=w479, "Action"=w495, "Test No."=w480, "Array No."=u32 3, 10:"Data IN"=w487, 11:"Data IN"=w478) -> ("Data OUT"=w494:cluster{dbl[], dbl[], dbl[], dbl[], dbl[]}[])  [unwired: 4 in, 1 out]
                                n287 = local write "RH [%]"(w487) -> ()
                                n288 = Greater?(x=w493, y=w490) -> (0:w488:bool)
                                }
                                frame #2 {
                                w520 = u32 5 ("y")
                                w540 = enum16{"Reset", "Write Element", "Read Array"}."Read Array" ("Action")
                                # "Increment the reading number."
                                # "Update the current and voltage indicators"
                                # "Update plots."
                                n289 = Increment(x=w519) -> (x+1=w516:u32)
                                n290 = Greater?(x=w516, y=w520) -> (0:w521:bool)
                                n291 = local read "Temperature Array"() -> (w512:dbl[])
                                n292 = local read "Humidity Array"() -> (w511:dbl[])
                                n293 = local read "Time"() -> (w510:u32[])
                                n294 = case shown="False" w521 {
                                tunnel: w520 -> [_ w545]
                                tunnel: w516 -> [w544 w547]
                                tunnel: [u32 0 w546] -> w518
                                tunnel: [w544 w545] -> w517
                                frame False {
                                }
                                frame True {
                                n295 = Subtract(x=w547, y=w545) -> (x-y=w546:u32)
                                }
                                }
                                n296 = call "StopWatch.vi"("Action"=enum16{"Start", "Stop", "Read", "Reset"}."Read") -> ("Time elapsed"=w509:u32)  [unwired: 4 out]
                                n297 = local write "IV Current reading No."(w516) -> ()
                                n298 = call "TestData.vi"("Action"=w540, "Test No."=w537, "Array No."=u32 0, "Data IN"=w539) -> ("Array OUT"=w524:dbl[], "Data OUT"=w538:cluster{dbl[], dbl[], dbl[], dbl[], dbl[]}[])  [unwired: 6 in]
                                n299 = property on="IV Graph" class="XYGraph (strict)"() -> ("YScale.Mapping Mode"=w541:u8)  [unwired: 2 in, 2 out]
                                n300 = Array Subset(array=w524, index=w518, length=w517) -> (w525:dbl[])
                                n301 = local write "Run time"(w509) -> ()
                                n302 = Build Array (concatenate)(w512, w528) -> (w507:dbl[])
                                n303 = Build Array (concatenate)(w511, w529) -> (w506:dbl[])
                                n304 = Build Array (concatenate)(w510, w509) -> (w508:u32[])
                                n305 = local write "Temperature Array"(w507) -> ()
                                n306 = local write "Humidity Array"(w506) -> ()
                                n307 = local write "Time"(w508) -> ()
                                n308 = call "TestData.vi"("Action"=w540, "Test No."=w537, "Array No."=u32 1, "Data IN"=w538) -> ("Array OUT"=w523:dbl[], "Data OUT"=w531:cluster{dbl[], dbl[], dbl[], dbl[], dbl[]}[])  [unwired: 6 in]
                                n309 = local write "IV Volts"(w525) -> ()
                                n310 = property on="IV Graph" class="XYGraph (strict)"("YScale.Minimum"=w541) -> ()  [unwired: 2 in, 2 out]
                                n311 = local read "IV Graph"() -> (w536:cluster{dbl[], dbl[]}[])
                                n312 = Array Subset(array=w523, index=w518, length=w517) -> (w522:dbl[])
                                n313 = local write "IV Current"(w522) -> ()
                                n314 = Bundle(w508, w507) -> (w515:cluster{u32[], dbl[]})  [unwired: 1 in]
                                n315 = Bundle(w508, w506) -> (w514:cluster{u32[], dbl[]})  [unwired: 1 in]
                                n316 = call "IVScaleYAxis.vi"("Data IN"=w531, "Plot In"=w536, "Y Scale"=w534) -> ("Plot Out"=w535:cluster{dbl[], dbl[]}[])  [unwired: 8 in]
                                n317 = Build Array(w515, w514) -> (w505:cluster{u32[], dbl[]}[])
                                n318 = local write "IV Graph"(w535) -> ()
                                n319 = local write "IV Data"(w531) -> ()
                                n320 = local write "TGraph"(w505) -> ()
                                }
                                frame #3 {
                                # "Increment the voltage or hold if necessary."
                                # "Check if final voltage \nhas been reached."
                                # "Ramp up voltage or hold at maximum voltage."
                                n321 = local read "IV step [V]"() -> (w552:dbl)
                                n322 = local read "IV Final volts [V]"() -> (w557:dbl)
                                n323 = Subtract(x=w553, y=w552) -> (x-y=w554:dbl)
                                n324 = Greater Or Equal?(x=w554, y=w557) -> (x >= y?=w556:bool)
                                n325 = case shown="True" w556 {
                                tunnel: w555 -> [_ w573]
                                tunnel: w554 -> [_ w571]
                                tunnel: w553 -> [_ w570]
                                tunnel: w552 -> [_ w569]
                                tunnel: w551 -> [w564 _]
                                tunnel: [w563 0] -> w550
                                tunnel: [w562 w567] -> w549
                                tunnel: [w561 w566] -> w548
                                frame False {
                                n326 = local read "IV hold steps"() -> (w565:i32)
                                n327 = local read "IV Current Volts:"() -> (w561:dbl)
                                n328 = Increment(x=w564) -> (x+1=w563:i32)
                                n329 = Greater Or Equal?(x=w564, y=w565) -> (x >= y?=w562:bool)
                                }
                                frame True {
                                n330 = call "SupplyRamp.vi"("Requested Voltage"=w571, "Step Size"=w569, "Step Delay"=100, "Supply IN"=w573, "Starting Voltage"=w570) -> ("Compliance exceeded"=w567:bool, "Current Voltage"=w566:dbl)  [unwired: 3 in, 2 out]
                                n331 = local write "IV STATUS"("Incrementing volts.") -> ()
                                n332 = property on="IV Bias On/Off:" class="Bool (strict)"("Blinking"=w567) -> ()  [unwired: 2 in, 2 out]
                                }
                                }
                                n333 = local write "IV Current Volts:"(w548) -> ()
                                }
                                frame #4 {
                                # "Check for compliance."
                                n334 = local read "RH [%]"() -> (w578:dbl)
                                n335 = Greater?(x=w578, y=10.0) -> (0:w576:bool)
                                n336 = case shown="True" w576 {
                                selector: w576 -> [w587 _]
                                tunnel: [w587 w588] -> w575
                                frame False {
                                }
                                frame True {
                                n337 = flat-sequence {
                                tunnel: [w590] -> w588
                                frame #0 {
                                n338 = Wait (ms)(milliseconds to wait=u32 10000) -> ()  [unwired: 1 out]
                                }
                                frame #1 {
                                # "Humidity debouncing."
                                n339 = global read "QC_MeasurementSetup.vi" "Hardware Settings"() -> (w595:T11)
                                n340 = Unbundle By Name(w595) -> ("Arduino"=w594:refnum<class "ArduinoControl.lvclass">)
                                n341 = call "ArduinoRead.vi"("Arduino function"=T6."T/RH", "ArduinoControl in"=w594) -> ("rel. Humidity [%]"=w591:dbl)  [unwired: 4 in, 5 out]
                                n342 = Greater?(x=w591, y=10.0) -> (0:w590:bool)
                                }
                                }
                                }
                                }
                                n343 = local read "Abort Test"() -> (w581:bool)
                                n344 = Build Array(w575, w582, w581, w580) -> (w583:bool[])
                                n345 = Or Array Elements(Boolean array=w583) -> (logical OR=w584:bool)
                                n346 = Not(x=w584) -> (.not. x?=w579:bool)
                                }
                              }
                            }
                          }
                          frame True {
                            n347 = local write "IV STATUS"("Run aborted - compliance exceeded.") -> ()
                          }
                        }
                      }
                      frame #2 {
                        # "Ramp down the voltage and save the data."
                        n348 = flat-sequence {
                          tunnel: [w618] -> w602
                          tunnel: w601 -> [w618]
                          tunnel: [w616] -> w599
                          tunnel: [w615] -> w597
                          tunnel: w602 -> [w623]
                          tunnel: [w623] -> w600
                          tunnel: w599 -> [w625]
                          tunnel: [w625] -> w598
                          tunnel: w597 -> [w624]
                          tunnel: w600 -> [w638]
                          tunnel: w598 -> [w644]
                          frame #0 {
                            # "Ramp down the voltage."
                            n349 = global read "QC_MeasurementSetup.vi" "Hardware Settings"() -> (w609:T11)
                            n350 = global read "QC_MeasurementSetup.vi" "IV Measurement Parameters"() -> (w607:T10)
                            n351 = Unbundle By Name(w609) -> ("Switching GPIB Address"=w615:string, "Supply"=w608:refnum<class "SupplyControl.lvclass">)
                            n352 = Unbundle By Name(w607) -> ("Ramp down steps [V]"=w606:dbl, "Ramp down Interval [s]"=w605:i32, "V_breakdown Limit [V]"=w616:dbl)
                            n353 = local write "IV STATUS"("Ramping down voltage.") -> ()
                            n354 = local read "IV Current Volts:"() -> (w611:dbl)
                            n355 = Multiply(x=w605, y=1000) -> (x*y=w603:i32)
                            n356 = call "SupplyRamp.vi"("Requested Voltage"=0.0, "Step Size"=w606, "Step Delay"=w603, "Supply IN"=w608, "Starting Voltage"=w611) -> ("error out"=w614:errorcluster, "Supply OUT"=w613:refnum<class "SupplyControl.lvclass">, "Current Voltage"=w610:dbl)  [unwired: 3 in, 1 out]
                            n357 = local write "IV Current Volts:"(w610) -> ()
                            n358 = call-dynamic "Supply_Stby.vi"("error in (no error)"=w614, "SupplyControl in"=w613) -> ()  [unwired: 8 in, 2 out]
                          }
                          frame #1 {
                            w622 = u16 1 items=["open all channels", "open channels in channel list", "close channels in channel list"] ("open/close (open all:0)")
                            # "Disconnect the sensor that was tested."
                            n359 = Build Array(w623) -> (w621:i32[])
                            n360 = call "ChannelListGenerator.vi"("Card Type"=enum16{"7036", "7054"}."7054", "Channels"=w621) -> ("Channel List"=w619:T15)  [unwired: 9 in]
                            n361 = call "Keith 7002 Open/Close Chan.vi"("GPIB address"=w624, "open/close (open all:0)"=w622, "channel list"=w619) -> ()  [unwired: 1 in, 1 out]
                          }
                          frame #2 {
                            w660 = enum16{"Reset", "Write Element", "Read Array"}."Read Array" ("Action")
                            # "T and RH double-precision numbers\nmodified to the DB standard with only \n1 digit after the decimal"
                            # "Save the data. Save the mean temperature and %RH. \nSave the arrays of current and voltage."
                            n362 = local read "IV Current reading No."() -> (w647:u32)
                            n363 = local read "IV Data"() -> (w639:cluster{dbl[], dbl[], dbl[], dbl[], dbl[]}[])
                            n364 = local write "IV STATUS"("Saving Data.") -> ()
                            n365 = call "ScanFeedback.vi"("Data IN"=w639, "measurement type"=T7."IV", "Test No."=w638) -> ("V breakdown"=w641:dbl)  [unwired: 2 in, 4 out]
                            n366 = Absolute Value(x=w641) -> (abs(x)=w642:dbl)
                            n367 = Absolute Value(x=w644) -> (abs(x)=w643:dbl)
                            n368 = call "TestData.vi"("Action"=w660, "Test No."=w638, "Array No."=u32 0, "Data IN"=w639) -> ("Array OUT"=w637:dbl[], "Data OUT"=w659:cluster{dbl[], dbl[], dbl[], dbl[], dbl[]}[])  [unwired: 6 in]
                            n369 = Array Size(array=w637) -> (size(s)=w636:i32)
                            n370 = Greater Or Equal?(x=w642, y=w643) -> ()  [unwired: 1 out]
                            n371 = call "TestData.vi"("Action"=w660, "Test No."=w638, "Array No."=u32 1, "Data IN"=w659) -> ("Array OUT"=w652:dbl[], "Data OUT"=w658:cluster{dbl[], dbl[], dbl[], dbl[], dbl[]}[])  [unwired: 6 in]
                            n372 = Initialize Array(0.0 ("element"), w636) -> (w634:dbl[])
                            n373 = call "TestData.vi"("Action"=w660, "Test No."=w638, "Array No."=u32 2, "Data IN"=w658) -> ("Array OUT"=w650:dbl[], "Data OUT"=w657:cluster{dbl[], dbl[], dbl[], dbl[], dbl[]}[])  [unwired: 6 in]
                            n374 = call "TestData.vi"("Action"=w660, "Test No."=w638, "Array No."=u32 3, "Data IN"=w657) -> ("Array OUT"=w649:dbl[])  [unwired: 6 in, 1 out]
                            n375 = Build Array(w637, w652, w634) -> (w651:dbl[][])
                            n376 = call "ComputeMean.vi"("Array In"=w649, "No. of Readings"=w647) -> ("Mean"=w631:dbl)  [unwired: 9 in]
                            n377 = call "ComputeMean.vi"("Array In"=w650, "No. of Readings"=w647) -> ("Mean"=w628:dbl)  [unwired: 9 in]
                            n378 = Transpose 2D Array(2D array=w651) -> (transposed array=w646:dbl[][])
                            n379 = Number To Fractional String(number=w631, precision (6)=1) -> (F-format string=w632:string)  [unwired: 2 in]
                            n380 = Number To Fractional String(number=w628, precision (6)=1) -> (F-format string=w627:string)  [unwired: 2 in]
                            n381 = Fract/Exp String To Number(string=w627) -> (number=w626:dbl)  [unwired: 3 in, 1 out]
                            n382 = Fract/Exp String To Number(string=w632) -> (number=w630:dbl)  [unwired: 3 in, 1 out]
                            n383 = call "SaveDataFile.vi"("Data Array"=w646, "Temperature"=w626, "Channel Number"=w638, "Humidity"=w630, "Array Titles"="Voltage[V]\tCurrent[nA]\tShunt_voltage[mV]", "Strip Segment"="") -> ()  [unwired: 6 in, 4 out]
                          }
                          frame #3 {
                            n384 = global read "QC_MeasurementSetup.vi" "Run Info"() -> (w665:T12)
                            n385 = local read "IV Test CH"() -> (w666:i32)
                            n386 = Unbundle By Name(w665) -> ("IV"=w664:bool[])
                            n387 = Replace Array Subset(array=w664, new element=TRUE ("new element/subarray"), index=w666) -> (w663:bool[])
                            n388 = Bundle By Name(cluster=w665, "IV"=w663) -> (w667:T12)
                            n389 = global write "QC_MeasurementSetup.vi" "Run Info"(w667) -> ()
                          }
                        }
                      }
                    }
                  }
                }
                "IV Test CH" <- w324
              }
            }
            frame #2 {
              # "Shut down the IV test. Open all channels in the electronics box."
              n390 = flat-sequence {
                tunnel: [w670] -> w668
                tunnel: w668 -> [w674]
                frame #0 {
                  # "Open all cahnnels in arduino."
                  n391 = global read "QC_MeasurementSetup.vi" "Hardware Settings"() -> (w672:T11)
                  n392 = Unbundle By Name(w672) -> ("Arduino"=w671:refnum<class "ArduinoControl.lvclass">, "Switching GPIB Address"=w670:string)
                  n393 = call "ArduinoRead.vi"("Arduino function"=T6."Reset Switches", "ArduinoControl in"=w671) -> ()  [unwired: 4 in, 6 out]
                }
                frame #1 {
                  w673 = u16 0 items=["open all channels", "open channels in channel list", "close channels in channel list"] ("open/close (open all:0)")
                  # "Open all channels in Keithley 7002."
                  n394 = call "Keith 7002 Open/Close Chan.vi"("GPIB address"=w674, "open/close (open all:0)"=w673) -> ()  [unwired: 2 in, 1 out]
                }
              }
            }
          }
        }
      }
    }
    frame #3 {
      # "CV Test code. Check to see if the CV test will be perfromed."
      n395 = global read "QC_MeasurementSetup.vi" "Run Info"() -> (w681:T12)
      n396 = Unbundle By Name(w681) -> ("No. of Ch."=w679:u16, "Sensor Serials"=w680:string[], "CV Test?"=w677:bool)
      n397 = local read "Abort Test"() -> (w675:bool)
      n398 = Not(x=w675) -> (.not. x?=w676:bool)
      n399 = And(x=w677, y=w676) -> (x .and. y?=w678:bool)
      n400 = case shown="True" w678 {
        tunnel: w680 -> [_ w682]
        tunnel: w679 -> [_ w683]
        frame False {
        }
        frame True {
          n401 = stacked-sequence {
            tunnel: w683 -> [_ w727 _]
            tunnel: w682 -> [_ w726 _]
            frame #0 {
              # "Setup page. Load the settings to the front page and set any parameters wich only need to be set once."
              n402 = flat-sequence {
                frame #0 {
                  w684 = u32 0 ("CV Current reading No.")
                  w701 = FALSE ("CV Bias On/Off:")
                  w706 = 0.0
                  w704 = ""
                  # "Reset the CV Data Structure. All IV data is stored in here.\nArray mapping is 1.) Voltage, 2.) Current, 3.) Temperature\n4.) %RH 5.) Resistance"
                  # "Set all of the paramaters of the status window to their initial values."
                  # "Setup the CV front panel parameters and switch to the tab."
                  n403 = global read "QC_MeasurementSetup.vi" "CV Measurement Parameters"() -> (w692:T9)
                  n404 = property on="CV Graph" class="XYGraph (strict)"() -> ("XScale.Mapping Mode"=w695:u8, "YScale.Mapping Mode"=w694:u8)  [unwired: 2 in, 2 out]
                  n405 = Initialize Array(w706, w706) -> (→"CV Capacitance" →"CV Resistance" →"CV Volts":dbl[])
                  n406 = Initialize Array(cluster{dbl[], dbl[]} {[], []}, 24 ("dimension size")) -> (→"CV Graph":cluster{dbl[], dbl[]}[])
                  n407 = local write "Test Control"(T4."CV Test " ("Test Control")) -> ()
                  n408 = Build Array("1/C^2 [1/nF^2]", "nF", "pF") -> (w709:string[])
                  n409 = Multiply(x=w694, y=2) -> (x*y=w712:i32)
                  n410 = property on="Cscale" class="Enum (strict)"("Strings []"=w709) -> ()  [unwired: 2 in, 2 out]
                  n411 = Add(x=w695, y=w712) -> (x+y=w693:i32)
                  n412 = property on="CV Bias On/Off:" class="Bool (strict)"("Blinking"=w701) -> ()  [unwired: 2 in, 2 out]
                  n413 = Unbundle By Name(w692) -> ("Final Voltage [V]"=→"CV Final volts [V]":dbl, "Initial Voltage [V]"=→"CV Initial volts [V]":dbl, "Number Of Steps"=→"CV No of steps":u32, "Step Size [V]"=→"CV step [V]":dbl, "Step Interval [s]"=→"CV step interval [s]":i32, "AC frequency [Hz]"=→"Frequency [Hz]":i32)
                  n414 = local write "CV Scales"(w693) -> ()
                  n415 = local write "Cscale"(0) -> ()
                  n416 = call "TestData.vi"("Action"=enum16{"Reset", "Write Element", "Read Array"}."Reset") -> ("Data OUT"=→"CV Data":cluster{dbl[], dbl[], dbl[], dbl[], dbl[]}[])  [unwired: 9 in, 1 out]
                  "CV Sensor No.:" <- w704
                  "CV Test Channel:" <- w704
                  "CV Time Initiated:" <- w704
                  "CV Last reading at:" <- w704
                  "CV STATUS" <- "INITIALISING CV RUN"
                  "CV Bias On/Off:" <- w701
                  "CV Current Volts:" <- w684
                  "CV Current reading No." <- w684
                }
                frame #1 {
                  # "Perform the switching on the Arduino."
                  n417 = global read "QC_MeasurementSetup.vi" "Hardware Settings"() -> (w715:T11)
                  n418 = Unbundle By Name(w715) -> ("Arduino"=w716:refnum<class "ArduinoControl.lvclass">)
                  n419 = flat-sequence {
                    tunnel: w716 -> [w720]
                    tunnel: [w719] -> w714
                    tunnel: [w718] -> w713
                    tunnel: w714 -> [w725]
                    tunnel: w713 -> [w723]
                    tunnel: [w722] -> _
                    frame #0 {
                      # "Reset all switches"
                      n420 = call "ArduinoRead.vi"("Arduino function"=T6."Reset Switches", "ArduinoControl in"=w720) -> ("error out"=w718:errorcluster, "ArduinoControl out"=w719:refnum<class "ArduinoControl.lvclass">)  [unwired: 4 in, 4 out]
                    }
                    frame #1 {
                      # "Perform Pre-Switching for IV. Switch the SMU Hi to a path through a \nsingle protection resistance (DP 8, 1MOhm). Switch the SMU Lo and LCR Lo to common of KE 7036 (DP 10, 7). Switch Hi of LCR to protection cap \n (DP 6)."
                      n421 = call "ArduinoRead.vi"("Command String"="6,7,8,10,", "Arduino function"=T6."Close Switch", "error in (no error)"=w723, "ArduinoControl in"=w725) -> ("ArduinoControl out"=w722:refnum<class "ArduinoControl.lvclass">)  [unwired: 2 in, 5 out]
                    }
                  }
                }
              }
            }
            frame #1 {
              n422 = for {
                N: w727 -> [_]
                tunnel: w726 -> [w732] mode=indexing
                i -> [w733]
                n423 = local read "Abort Test"() -> (w731:bool)
                n424 = Not(x=w731) -> (.not. x?=w730:bool)
                n425 = Not Equal?(x=w732, y="") -> (x != y?=w729:bool)
                n426 = And(x=w730, y=w729) -> (x .and. y?=w728:bool)
                n427 = case shown="True" w728 {
                  tunnel: w732 -> [_ w735]
                  tunnel: w733 -> [_ w736]
                  frame False {
                  }
                  frame True {
                    n428 = stacked-sequence {
                      tunnel: w736 -> [w745 _ w1028]
                      tunnel: w735 -> [w737 _ _]
                      frame #0 {
                        # "Connect to the channel and initialize the LCR and SMU."
                        n429 = flat-sequence {
                          tunnel: w737 -> [w754]
                          tunnel: w745 -> [w752]
                          tunnel: [w752] -> w744
                          tunnel: [w751] -> w743
                          tunnel: [w750] -> w742
                          tunnel: [w749] -> w738
                          tunnel: w744 -> [w770]
                          tunnel: w743 -> [w773]
                          tunnel: w742 -> [w772]
                          tunnel: [w773] -> w741
                          tunnel: [w772] -> w740
                          tunnel: w738 -> [w771]
                          tunnel: w741 -> [w805]
                          tunnel: w740 -> [w804]
                          tunnel: [w802] -> w739
                          tunnel: w739 -> [w807]
                          frame #0 {
                            # "SubVI to obtain Date/Time in\nstandard DB format independently\nof the OS language"
                            # "Record vital information for the Run Info."
                            n430 = call "GetDateTimeDBFormat.vi"() -> ("Time in 24h format, e.g. 13:40:54"=w746:string, "Abbreviated Date, e.g. 13 Nov 2020"=w747:string)  [unwired: 10 in]
                            n431 = Increment(x=w752) -> (x+1=w748:i32)
                            n432 = local write "CV Sensor No.:"(w754) -> ()
                            n433 = global read "QC_MeasurementSetup.vi" "Hardware Settings"() -> (w760:T11)
                            n434 = Number To Decimal String(number=w748) -> (decimal integer string=w753:string)  [unwired: 1 in]
                            n435 = local write "CV Time Initiated:"(w746) -> ()
                            n436 = Unbundle By Name(w760) -> ("Supply"=w751:refnum<class "SupplyControl.lvclass">, "LCR"=w750:refnum<class "LCRControl.lvclass">, "SMU Name"=w758:string, "LCR Name"=w757:string, "Switching GPIB Address"=w749:string)
                            n437 = local write "CV Test Channel:"(w753) -> ()
                            n438 = global read "QC_MeasurementSetup.vi" "Run Info"() -> (w763:T12)
                            n439 = local write "CV Current reading No."(u32 0 ("CV Current reading No.")) -> ()
                            n440 = Concatenate Strings(w758, "," ("string"), w757) -> (w756:string)
                            n441 = Bundle By Name(cluster=w763, "Test Date"=w747, "Test Time"=w746, "Current Sensor"=w754, "Current Test"="CV", "Instruments"=w756) -> (w762:T12)
                            n442 = global write "QC_MeasurementSetup.vi" "Run Info"(w762) -> ()
                          }
                          frame #1 {
                            w766 = u16 2 items=["open all channels", "open channels in channel list", "close channels in channel list"] ("open/close (open all:0)")
                            # "Code to connect the HV matrix and the LV matrix channels (to be done)"
                            n443 = Build Array(w770) -> (w769:i32[])
                            n444 = call "ChannelListGenerator.vi"("Card Type"=enum16{"7036", "7054"}."7036", "Channels"=w769) -> ("Channel List"=w765:T15)  [unwired: 9 in]
                            n445 = call "ChannelListGenerator.vi"("Card Type"=enum16{"7036", "7054"}."7054", "Channels"=w769) -> ("Channel List"=w764:T15)  [unwired: 9 in]
                            n446 = call "Keith 7002 Open/Close Chan.vi"("GPIB address"=w771, "open/close (open all:0)"=w766, "channel list"=w765) -> ()  [unwired: 1 in, 1 out]
                            n447 = call "Keith 7002 Open/Close Chan.vi"("GPIB address"=w771, "open/close (open all:0)"=w766, "channel list"=w764) -> ()  [unwired: 1 in, 1 out]
                          }
                          frame #2 {
                            # "Write out Capacitance\nand Resistance for debugging."
                            # "Initialize LCR meter and SMU."
                            n448 = global read "QC_MeasurementSetup.vi" "CV Measurement Parameters"() -> (w776:T9)
                            n449 = global read "InstrumentSetup.vi" "Keithley 2410 Configurations"() -> (w779:T16)
                            n450 = call-dynamic "Supply_Reset.vi"("SupplyControl in"=w805) -> ("error out"=w797:errorcluster, "SupplyControl out"=w801:refnum<class "SupplyControl.lvclass">)  [unwired: 9 in]
                            n451 = call-dynamic "Supply_Init.vi"("error in (no error)"=w797, "SupplyControl in"=w801) -> ("error out"=w774:errorcluster, "SupplyControl out"=w775:refnum<class "SupplyControl.lvclass">)  [unwired: 8 in]
                            n452 = local read "CV Initial volts [V]"() -> (w792:dbl)
                            n453 = Unbundle By Name(w776) -> ("Current Limit [µA]"=w780:dbl)
                            n454 = local read "CV step [V]"() -> (w791:dbl)
                            n455 = Multiply(x=w780, y=1e-06) -> (x*y=w777:dbl)
                            n456 = call-dynamic "Supply_Arm.vi"("error in (no error)"=w774, "SupplyControl in"=w775) -> ("error out"=w796:errorcluster, "SupplyControl out"=w800:refnum<class "SupplyControl.lvclass">)  [unwired: 8 in]
                            n457 = Bundle By Name(cluster=w779, "Current Limit"=w777) -> (w778:T16)
                            n458 = local read "Frequency [Hz]"() -> (w782:i32)
                            n459 = call "SupplyRamp.vi"("error in"=w796, "Requested Voltage"=0.0, "Step Size"=w791, "Step Delay"=u32 100, "Supply IN"=w800, "Starting Voltage"=w792) -> ("error out"=w795:errorcluster, "Supply OUT"=w799:refnum<class "SupplyControl.lvclass">, "Compliance exceeded"=w802:bool, "Current Voltage"=w803:dbl)  [unwired: 2 in]
                            n460 = global write "InstrumentSetup.vi" "Keithley 2410 Configurations"(w778) -> ()
                            n461 = call-dynamic "Supply_ReadCurrent.vi"("error in (no error)"=w795, "SupplyControl in"=w799) -> ("error out"=w794:errorcluster)  [unwired: 7 in, 2 out]
                            n462 = call-dynamic "LCR_Init.vi"("error in (no error)"=w794, "LCRControl in"=w804) -> ("error out"=w793:errorcluster, "LCRControl out"=w798:refnum<class "LCRControl.lvclass">)  [unwired: 8 in]
                            n463 = call-dynamic "LCR_Readout.vi"("error in (no error)"=w793, "Frequency in Hz"=w782, "LCRControl in"=w798) -> ("Resistance in Ohm"=w787:dbl, "Capacitance in pF"=w788:dbl)  [unwired: 5 in, 2 out]
                            n464 = Initialize Array(w788, 1) -> (w785:dbl[])
                            n465 = Initialize Array(w787, 1) -> (w786:dbl[])
                            n466 = local write "CV Current Volts:"(w803) -> ()
                            n467 = local write "CV Capacitance"(w785) -> ()
                            n468 = local write "CV Resistance"(w786) -> ()
                          }
                          frame #3 {
                            # "Added a wait to try to discharge the capacitor between runs."
                            n469 = case shown="True" w807 {
                              selector: w807 -> [w808 w809]
                              frame False {
                                n470 = property on="CV Bias On/Off:" class="Bool (strict)"("Blinking"=w808) -> ()  [unwired: 2 in, 2 out]
                              }
                              frame True {
                                n471 = property on="CV Bias On/Off:" class="Bool (strict)"("Blinking"=w809) -> ()  [unwired: 2 in, 2 out]
                                n472 = local write "CV STATUS"("Compliance exceeded\nRUN ABORTED") -> ()
                              }
                            }
                            n473 = Wait (ms)(milliseconds to wait=u32 10000) -> ()  [unwired: 1 out]
                          }
                        }
                      }
                      frame #1 {
                        n474 = local read "CV Scales"() -> (w812:T2)
                        n475 = local read "Cscale"() -> (w811:enum16{"1/C^2 [1/nF^2]", "nF", "pF"})
                        n476 = while {
                          shift-right: [w815] -> _
                          shift-left: w812 -> [w839]
                          shift-right: [w813] -> _
                          shift-left: w811 -> [w837]
                          stop <- w817 continue-if-true
                          # "Measurement loop."
                          n477 = flat-sequence {
                            tunnel: w839 -> [w852]
                            tunnel: [w851] -> w838
                            tunnel: w837 -> [w850]
                            tunnel: [w841] -> w836
                            tunnel: [w840] -> w835
                            tunnel: w838 -> [w908]
                            tunnel: w836 -> [w907]
                            tunnel: w835 -> [w903]
                            tunnel: [w927] -> w834
                            tunnel: [w921] -> w833
                            tunnel: [w911] -> w832
                            tunnel: [w901] -> w831
                            tunnel: [w908] -> w830
                            tunnel: [w907] -> w829
                            tunnel: [w906] -> w828
                            tunnel: [w905] -> w826
                            tunnel: [w904] -> w825
                            tunnel: [w900] -> w821
                            tunnel: w834 -> [w973]
                            tunnel: w833 -> [w964]
                            tunnel: w832 -> [w959]
                            tunnel: w831 -> [w977]
                            tunnel: w830 -> [w961]
                            tunnel: w829 -> [w962]
                            tunnel: w828 -> [w963]
                            tunnel: [w962] -> w827
                            tunnel: w826 -> [w975]
                            tunnel: w825 -> [w974]
                            tunnel: [w964] -> w824
                            tunnel: [w961] -> w823
                            tunnel: [w960] -> w822
                            tunnel: w821 -> [w960]
                            tunnel: [w959] -> w820
                            tunnel: w827 -> [w984]
                            tunnel: w824 -> [w988]
                            tunnel: w823 -> [w985]
                            tunnel: w822 -> [w989]
                            tunnel: w820 -> [w987]
                            tunnel: [w987] -> w819
                            tunnel: [w986] -> w818
                            tunnel: [w985] -> w816
                            tunnel: [w984] -> w814
                            tunnel: w819 -> [w1013]
                            tunnel: w818 -> [w1012]
                            tunnel: [w1010] -> w817
                            tunnel: w816 -> [w1009]
                            tunnel: [w1009] -> w815
                            tunnel: w814 -> [w1008]
                            tunnel: [w1008] -> w813
                            frame #0 {
                              # "Wait and allow the user to adjust the graph scales if they want."
                              n478 = local read "CV step interval [s]"() -> (w842:u32)
                              n479 = Get Date/Time In Seconds() -> (seconds since 1Jan1904=w848:timestamp)
                              n480 = Format Into String(format string="%d" ("initial string"), w842) -> (resulting string=w849:string)  [unwired: 2 in, 1 out]
                              n481 = To Double Precision Float(number=w848) -> (double precision float=w846:dbl)
                              n482 = Concatenate Strings("Waiting for " ("string"), w849, " seconds...") -> (w847:string)
                              n483 = while {
                                shift-right: [w875] -> w851
                                shift-left: w852 -> [w876]
                                shift-right: [w872] -> w841
                                shift-left: w850 -> [w873]
                                tunnel: w847 -> [w859]
                                tunnel: w846 -> [w861]
                                tunnel: w842 -> [w860]
                                tunnel: [w853] -> w840
                                stop <- w855 continue-if-true
                                n484 = local read "Cscale"() -> (w874:enum16{"1/C^2 [1/nF^2]", "nF", "pF"})
                                n485 = local read "CV Scales"() -> (w877:T2)
                                n486 = local read "CV Data"() -> (w870:cluster{dbl[], dbl[], dbl[], dbl[], dbl[]}[])
                                n487 = Get Date/Time In Seconds() -> (seconds since 1Jan1904=w864:timestamp)
                                n488 = Wait (ms)(milliseconds to wait=u32 100) -> ()  [unwired: 1 out]
                                n489 = Not Equal?(x=w873, y=w874) -> (x != y?=w878:bool)
                                n490 = Not Equal?(x=w876, y=w877) -> (x != y?=w879:bool)
                                n491 = To Double Precision Float(number=w864) -> (double precision float=w865:dbl)
                                n492 = case shown="True" w879 {
                                tunnel: w877 -> [w887 w888]
                                tunnel: [w887 w888] -> w875
                                frame False {
                                }
                                frame True {
                                n493 = case shown="\"Log - log\".." w888 {
                                tunnel: [w891 1 0 w896] -> w890
                                tunnel: [w891 0 1 w896] -> w889
                                frame .."Lin - Lin" {
                                w891 = 0
                                }
                                frame "Log - Lin" {
                                }
                                frame "Lin - Log" {
                                }
                                frame "Log - log".. {
                                w896 = 1
                                }
                                }
                                n494 = property on="CV Graph" class="XYGraph (strict)"("X Scale.Mapping Mode"=w890) -> ()  [unwired: 2 in, 2 out]
                                n495 = property on="CV Graph" class="XYGraph (strict)"("Y Scale.Mapping Mode"=w889, "YScale.Minimum"=w889) -> ()  [unwired: 2 in, 2 out]
                                }
                                }
                                n496 = case shown="True" w878 {
                                tunnel: [w880 w882] -> w872
                                tunnel: w874 -> [w880 w882]
                                tunnel: w870 -> [w881 w883]
                                tunnel: [w881 w883] -> w853
                                frame False {
                                }
                                frame True {
                                n497 = local read "CV Graph"() -> (w884:cluster{dbl[], dbl[]}[])
                                n498 = property on="CV Graph" class="XYGraph (strict)"() -> ("YScale.Mapping Mode"=w886:u8)  [unwired: 2 in, 2 out]
                                n499 = call "CVScaleYAxis.vi"("Data IN"=w883, "Plot In"=w884, "Y Scale"=w882) -> ("Plot Out"=w885:cluster{dbl[], dbl[]}[])  [unwired: 8 in]
                                n500 = property on="CV Graph" class="XYGraph (strict)"("YScale.Minimum"=w886) -> ()  [unwired: 2 in, 2 out]
                                n501 = local write "CV Graph"(w885) -> ()
                                }
                                }
                                n502 = Subtract(x=w865, y=w861) -> (x-y=w863:dbl)
                                n503 = Subtract(x=w860, y=w863) -> (x-y=w862:dbl)
                                n504 = local read "Abort Test"() -> (w857:bool)
                                n505 = Format Into String(format string="%d", w862) -> (resulting string=w869:string)  [unwired: 2 in, 1 out]
                                n506 = Not(x=w857) -> (.not. x?=w858:bool)
                                n507 = Greater Than 0?(x=w862) -> (x > 0?=w856:bool)
                                n508 = Concatenate Strings(w859, "\r\n", "Timer status: ", w869) -> (w854:string)
                                n509 = local write "CV STATUS"(w854) -> ()
                                n510 = And(x=w856, y=w858) -> (x .and. y?=w855:bool)
                              }
                            }
                            frame #1 {
                              w920 = enum16{"Reset", "Write Element", "Read Array"}."Write Element" ("Action")
                              # "Set status and check if current is \nabove compliance."
                              # "Read fro the LCR meter, SMU and Arduino."
                              n511 = local read "Frequency [Hz]"() -> (w910:i32)
                              n512 = global read "QC_MeasurementSetup.vi" "Hardware Settings"() -> (w933:T11)
                              n513 = local read "CV Current reading No."() -> (w901:u32)
                              n514 = local read "CV Current Volts:"() -> (w900:dbl)
                              n515 = local read "CV Current Limit [µA]"() -> (w913:dbl)
                              n516 = local read "CV Test CH"() -> (w906:i32)
                              n517 = Get Date/Time String(want seconds? (F)=TRUE) -> (time string=w918:string)  [unwired: 2 in, 1 out]
                              n518 = Unbundle By Name(w933) -> ("Arduino"=w932:refnum<class "ArduinoControl.lvclass">, "LCR"=w929:refnum<class "LCRControl.lvclass">, "Supply"=w928:refnum<class "SupplyControl.lvclass">)
                              n519 = local write "CV Last reading at:"(w918) -> ()
                              n520 = call-dynamic "LCR_Readout.vi"("Frequency in Hz"=w910, "LCRControl in"=w929) -> ("Resistance in Ohm"=w909:dbl, "Capacitance in pF"=w926:dbl)  [unwired: 6 in, 2 out]
                              n521 = call-dynamic "Supply_ReadCurrent.vi"("SupplyControl in"=w928) -> ("Current in nA"=w912:dbl, "SupplyControl out"=w921:refnum<class "SupplyControl.lvclass">)  [unwired: 8 in, 1 out]
                              n522 = local write "CV STATUS"("Reading LCR Meter ..." ("status")) -> ()
                              n523 = call "ArduinoRead.vi"("Arduino function"=T6."T/RH", "ArduinoControl in"=w932) -> ("rel. Humidity [%]"=w904:dbl, "Temperature [°C]"=w905:dbl)  [unwired: 4 in, 4 out]
                              n524 = local write "Temp. [°C]"(w905) -> ()
                              n525 = call "TestData.vi"("Reading No."=w901, "Action"=w920, "Test No."=w906, "Array No."=u32 0, 10:"Data IN"=w900, 11:"Data IN"=w903) -> ("Data OUT"=w930:cluster{dbl[], dbl[], dbl[], dbl[], dbl[]}[])  [unwired: 4 in, 1 out]
                              n526 = call "TestData.vi"("Reading No."=w901, "Action"=w920, "Test No."=w906, "Array No."=u32 1, 10:"Data IN"=w926, 11:"Data IN"=w930) -> ("Data OUT"=w922:cluster{dbl[], dbl[], dbl[], dbl[], dbl[]}[])  [unwired: 4 in, 1 out]
                              n527 = Multiply(x=w913, y=1000.0) -> (x*y=w914:dbl)
                              n528 = call "TestData.vi"("Reading No."=w901, "Action"=w920, "Test No."=w906, "Array No."=u32 4, 10:"Data IN"=w909, 11:"Data IN"=w922) -> ("Data OUT"=w931:cluster{dbl[], dbl[], dbl[], dbl[], dbl[]}[])  [unwired: 4 in, 1 out]
                              n529 = call "TestData.vi"("Reading No."=w901, "Action"=w920, "Test No."=w906, "Array No."=u32 2, 10:"Data IN"=w905, 11:"Data IN"=w931) -> ("Data OUT"=w899:cluster{dbl[], dbl[], dbl[], dbl[], dbl[]}[])  [unwired: 4 in, 1 out]
                              n530 = call "TestData.vi"("Reading No."=w901, "Action"=w920, "Test No."=w906, "Array No."=u32 3, 10:"Data IN"=w904, 11:"Data IN"=w899) -> ("Data OUT"=w927:cluster{dbl[], dbl[], dbl[], dbl[], dbl[]}[])  [unwired: 4 in, 1 out]
                              n531 = Absolute Value(x=w912) -> (abs(x)=w916:dbl)
                              n532 = local write "RH [%]"(w904) -> ()
                              n533 = Greater?(x=w916, y=w914) -> (0:w911:bool)
                            }
                            frame #2 {
                              w947 = u32 5 ("y")
                              w970 = enum16{"Reset", "Write Element", "Read Array"}."Read Array" ("Action")
                              # "Update the plots and front pannel indicators."
                              n534 = Increment(x=w977) -> (x+1=w948:u32)
                              n535 = Greater?(x=w948, y=w947) -> (0:w949:bool)
                              n536 = case shown="False" w949 {
                                tunnel: w947 -> [_ w980]
                                tunnel: w948 -> [w979 w982]
                                tunnel: [u32 0 w981] -> w946
                                tunnel: [w979 w980] -> w945
                                frame False {
                                }
                                frame True {
                                n537 = Subtract(x=w982, y=w980) -> (x-y=w981:u32)
                                }
                              }
                              n538 = local read "Temperature Array"() -> (w939:dbl[])
                              n539 = local read "Humidity Array"() -> (w940:dbl[])
                              n540 = local read "Time"() -> (w941:u32[])
                              n541 = call "TestData.vi"("Action"=w970, "Test No."=w963, "Array No."=u32 0, "Data IN"=w973) -> ("Array OUT"=w951:dbl[], "Data OUT"=w972:cluster{dbl[], dbl[], dbl[], dbl[], dbl[]}[])  [unwired: 6 in]
                              n542 = call "StopWatch.vi"("Action"=enum16{"Start", "Stop", "Read", "Reset"}."Read") -> ("Time elapsed"=w937:u32)  [unwired: 4 out]
                              n543 = Array Subset(array=w951, index=w946, length=w945) -> (w950:dbl[])
                              n544 = property on="CV Graph" class="XYGraph (strict)"() -> ("YScale.Mapping Mode"=w976:u8)  [unwired: 2 in, 2 out]
                              n545 = local write "CV Volts"(w950) -> ()
                              n546 = call "TestData.vi"("Action"=w970, "Test No."=w963, "Array No."=u32 1, "Data IN"=w972) -> ("Array OUT"=w952:dbl[], "Data OUT"=w971:cluster{dbl[], dbl[], dbl[], dbl[], dbl[]}[])  [unwired: 6 in]
                              n547 = local write "CV Current reading No."(w948) -> ()
                              n548 = local write "Run time"(w937) -> ()
                              n549 = Build Array (concatenate)(w939, w975) -> (w935:dbl[])
                              n550 = Build Array (concatenate)(w940, w974) -> (w934:dbl[])
                              n551 = Build Array (concatenate)(w941, w937) -> (w936:u32[])
                              n552 = Array Subset(array=w952, index=w946, length=w945) -> (w953:dbl[])
                              n553 = local write "CV Capacitance"(w953) -> ()
                              n554 = property on="CV Graph" class="XYGraph (strict)"("YScale.Minimum"=w976) -> ()  [unwired: 2 in, 2 out]
                              n555 = call "TestData.vi"("Action"=w970, "Test No."=w963, "Array No."=u32 4, "Data IN"=w971) -> ("Array OUT"=w956:dbl[], "Data OUT"=w958:cluster{dbl[], dbl[], dbl[], dbl[], dbl[]}[])  [unwired: 6 in]
                              n556 = local write "Temperature Array"(w935) -> ()
                              n557 = local write "Humidity Array"(w934) -> ()
                              n558 = local write "Time"(w936) -> ()
                              n559 = Bundle(w936, w935) -> (w944:cluster{u32[], dbl[]})  [unwired: 1 in]
                              n560 = Bundle(w936, w934) -> (w943:cluster{u32[], dbl[]})  [unwired: 1 in]
                              n561 = local read "CV Graph"() -> (w968:cluster{dbl[], dbl[]}[])
                              n562 = Build Array(w944, w943) -> (w938:cluster{u32[], dbl[]}[])
                              n563 = Multiply(x=w956, y=0.001) -> (x*y=w955:dbl[])
                              n564 = call "CVScaleYAxis.vi"("Data IN"=w958, "Plot In"=w968, "Y Scale"=w962) -> ("Plot Out"=w969:cluster{dbl[], dbl[]}[])  [unwired: 8 in]
                              n565 = Array Subset(array=w955, index=w946, length=w945) -> (w954:dbl[])
                              n566 = local write "CV Resistance"(w954) -> ()
                              n567 = local write "TGraph"(w938) -> ()
                              n568 = local write "CV Graph"(w969) -> ()
                              n569 = local write "CV Data"(w958) -> ()
                            }
                            frame #3 {
                              # "Incremnt the voltage or stop the test if the final voltage has been reached."
                              # "Check if final voltage \nhas been reached."
                              n570 = local read "CV step [V]"() -> (w990:dbl)
                              n571 = local read "CV Final volts [V]"() -> (w993:dbl)
                              n572 = Subtract(x=w989, y=w990) -> (x-y=w992:dbl)
                              n573 = Greater Or Equal?(x=w992, y=w993) -> (x >= y?=w991:bool)
                              n574 = case shown="True" w991 {
                                tunnel: w992 -> [_ w1001]
                                tunnel: w990 -> [_ w1000]
                                tunnel: w989 -> [_ w999]
                                tunnel: w988 -> [_ w998]
                                tunnel: [TRUE ("Compliance exceeded") w997] -> w986
                                tunnel: [w994 w996] -> w983
                                frame False {
                                n575 = local read "CV Current Volts:"() -> (w994:dbl)
                                }
                                frame True {
                                n576 = call "SupplyRamp.vi"("Requested Voltage"=w1001, "Step Size"=w1000, "Step Delay"=100, "Supply IN"=w998, "Starting Voltage"=w999) -> ("Compliance exceeded"=w997:bool, "Current Voltage"=w996:dbl)  [unwired: 3 in, 2 out]
                                n577 = local write "CV STATUS"("Incrementing voltage.") -> ()
                                n578 = property on="CV Bias On/Off:" class="Bool (strict)"("Blinking"=w997) -> ()  [unwired: 2 in, 2 out]
                                }
                              }
                              n579 = local write "CV Current Volts:"(w983) -> ()
                            }
                            frame #4 {
                              # "Check if any of the conditons for ending the loop \nhave been met. Abort test button pressed, complinace \nexceded, test complete or humidity threshold exceeded."
                              n580 = local read "RH [%]"() -> (w1007:dbl)
                              n581 = Greater?(x=w1007, y=10.0) -> (0:w1005:bool)
                              n582 = case shown="True" w1005 {
                                selector: w1005 -> [w1016 _]
                                tunnel: [w1016 w1017] -> w1004
                                frame False {
                                }
                                frame True {
                                n583 = flat-sequence {
                                tunnel: [w1019] -> w1017
                                frame #0 {
                                n584 = Wait (ms)(milliseconds to wait=u32 10000) -> ()  [unwired: 1 out]
                                }
                                frame #1 {
                                # "Humidity debouncing."
                                n585 = global read "QC_MeasurementSetup.vi" "Hardware Settings"() -> (w1024:T11)
                                n586 = Unbundle By Name(w1024) -> ("Arduino"=w1023:refnum<class "ArduinoControl.lvclass">)
                                n587 = call "ArduinoRead.vi"("Arduino function"=T6."T/RH", "ArduinoControl in"=w1023) -> ("rel. Humidity [%]"=w1020:dbl)  [unwired: 4 in, 5 out]
                                n588 = Greater?(x=w1020, y=10.0) -> (0:w1019:bool)
                                }
                                }
                                }
                              }
                              n589 = local read "Abort Test"() -> (w1011:bool)
                              n590 = Build Array(w1011, w1012, w1013, w1004) -> (w1014:bool[])
                              n591 = Or Array Elements(Boolean array=w1014) -> (logical OR=w1015:bool)
                              n592 = Not(x=w1015) -> (.not. x?=w1010:bool)
                            }
                          }
                        }
                      }
                      frame #2 {
                        n593 = flat-sequence {
                          tunnel: [w1047] -> w1030
                          tunnel: [w1046] -> w1029
                          tunnel: w1028 -> [w1046]
                          tunnel: [w1045] -> w1025
                          tunnel: w1030 -> [w1062]
                          tunnel: w1029 -> [w1060]
                          tunnel: [w1062] -> w1027
                          tunnel: [w1060] -> w1026
                          tunnel: w1025 -> [w1059]
                          tunnel: w1027 -> [w1074]
                          tunnel: w1026 -> [w1072]
                          frame #0 {
                            # "Ramp down the bias voltage. Delay of 10s has been added to allow \nstored chage to disipate."
                            n594 = global read "QC_MeasurementSetup.vi" "Hardware Settings"() -> (w1043:T11)
                            n595 = global read "QC_MeasurementSetup.vi" "CV Measurement Parameters"() -> (w1042:T9)
                            n596 = Unbundle By Name(w1043) -> ("Supply"=w1034:refnum<class "SupplyControl.lvclass">, "Switching GPIB Address"=w1045:string)
                            n597 = Unbundle By Name(w1042) -> ("Ramp down steps [V]"=w1041:dbl, "Ramp down Interval [s]"=w1040:i32, "V_depletion Limit [V]"=w1047:dbl)
                            n598 = local write "CV STATUS"("Ramping down voltage.") -> ()
                            n599 = local read "CV Current Volts:"() -> (w1036:dbl)
                            n600 = Multiply(x=w1040, y=1000) -> (x*y=w1038:i32)
                            n601 = call "SupplyRamp.vi"("Requested Voltage"=0.0, "Step Size"=w1041, "Step Delay"=w1038, "Supply IN"=w1034, "Starting Voltage"=w1036) -> ("error out"=w1044:errorcluster, "Supply OUT"=w1033:refnum<class "SupplyControl.lvclass">, "Current Voltage"=w1035:dbl)  [unwired: 3 in, 1 out]
                            n602 = flat-sequence {
                              tunnel: w1033 -> [w1050]
                              tunnel: w1044 -> [w1051]
                              tunnel: [w1051] -> w1032
                              tunnel: [w1050] -> w1031
                              tunnel: w1032 -> [w1053]
                              tunnel: w1031 -> [w1052]
                              frame #0 {
                                n603 = Wait (ms)(milliseconds to wait=u32 10000) -> ()  [unwired: 1 out]
                              }
                              frame #1 {
                                n604 = call-dynamic "Supply_Stby.vi"("error in (no error)"=w1053, "SupplyControl in"=w1052) -> ()  [unwired: 8 in, 2 out]
                              }
                            }
                            n605 = local write "CV Current Volts:"(w1035) -> ()
                          }
                          frame #1 {
                            w1056 = u16 1 items=["open all channels", "open channels in channel list", "close channels in channel list"] ("open/close (open all:0)")
                            # "Disconnect the sensor that was tested."
                            n606 = Build Array(w1060) -> (w1061:i32[])
                            n607 = call "ChannelListGenerator.vi"("Card Type"=enum16{"7036", "7054"}."7036", "Channels"=w1061) -> ("Channel List"=w1055:T15)  [unwired: 9 in]
                            n608 = call "ChannelListGenerator.vi"("Card Type"=enum16{"7036", "7054"}."7054", "Channels"=w1061) -> ("Channel List"=w1054:T15)  [unwired: 9 in]
                            n609 = call "Keith 7002 Open/Close Chan.vi"("GPIB address"=w1059, "open/close (open all:0)"=w1056, "channel list"=w1055) -> ()  [unwired: 1 in, 1 out]
                            n610 = call "Keith 7002 Open/Close Chan.vi"("GPIB address"=w1059, "open/close (open all:0)"=w1056, "channel list"=w1054) -> ()  [unwired: 1 in, 1 out]
                          }
                          frame #2 {
                            w1071 = enum16{"Reset", "Write Element", "Read Array"}."Read Array" ("Action")
                            # "T and RH double-precision numbers\nmodified to the DB standard with only \n1 digit after the decimal"
                            n611 = local read "CV Current reading No."() -> (w1076:u32)
                            n612 = local read "CV Data"() -> (w1073:cluster{dbl[], dbl[], dbl[], dbl[], dbl[]}[])
                            n613 = local write "CV STATUS"("Saving Data.") -> ()
                            n614 = call "TestData.vi"("Action"=w1071, "Test No."=w1072, "Array No."=u32 0, "Data IN"=w1073) -> ("Array OUT"=w1094:dbl[], "Data OUT"=w1100:cluster{dbl[], dbl[], dbl[], dbl[], dbl[]}[])  [unwired: 6 in]
                            n615 = call "ScanFeedback.vi"("Data IN"=w1073, "measurement type"=T7."CV", "Test No."=w1072) -> ("V depletion"=w1077:dbl)  [unwired: 2 in, 4 out]
                            n616 = call "TestData.vi"("Action"=w1071, "Test No."=w1072, "Array No."=u32 1, "Data IN"=w1100) -> ("Array OUT"=w1093:dbl[], "Data OUT"=w1083:cluster{dbl[], dbl[], dbl[], dbl[], dbl[]}[])  [unwired: 6 in]
                            n617 = Absolute Value(x=w1077) -> (abs(x)=w1086:dbl)
                            n618 = Absolute Value(x=w1074) -> (abs(x)=w1087:dbl)
                            n619 = call "TestData.vi"("Action"=w1071, "Test No."=w1072, "Array No."=u32 4, "Data IN"=w1083) -> ("Array OUT"=w1079:dbl[], "Data OUT"=w1082:cluster{dbl[], dbl[], dbl[], dbl[], dbl[]}[])  [unwired: 6 in]
                            n620 = Less Or Equal?(x=w1086, y=w1087) -> ()  [unwired: 1 out]
                            n621 = call "TestData.vi"("Action"=w1071, "Test No."=w1072, "Array No."=u32 2, "Data IN"=w1082) -> ("Array OUT"=w1091:dbl[], "Data OUT"=w1099:cluster{dbl[], dbl[], dbl[], dbl[], dbl[]}[])  [unwired: 6 in]
                            n622 = Multiply(x=w1079, y=1e-06) -> (x*y=w1078:dbl[])
                            n623 = call "TestData.vi"("Action"=w1071, "Test No."=w1072, "Array No."=u32 3, "Data IN"=w1099) -> ("Array OUT"=w1090:dbl[])  [unwired: 6 in, 1 out]
                            n624 = Build Array(w1094, w1093, w1078) -> (w1092:dbl[][])
                            n625 = call "ComputeMean.vi"("Array In"=w1090, "No. of Readings"=w1076) -> ("Mean"=w1068:dbl)  [unwired: 9 in]
                            n626 = call "ComputeMean.vi"("Array In"=w1091, "No. of Readings"=w1076) -> ("Mean"=w1064:dbl)  [unwired: 9 in]
                            n627 = Transpose 2D Array(2D array=w1092) -> (transposed array=w1089:dbl[][])
                            n628 = Number To Fractional String(number=w1064, precision (6)=1) -> (F-format string=w1065:string)  [unwired: 2 in]
                            n629 = Number To Fractional String(number=w1068, precision (6)=1) -> (F-format string=w1069:string)  [unwired: 2 in]
                            n630 = Fract/Exp String To Number(string=w1065) -> (number=w1063:dbl)  [unwired: 3 in, 1 out]
                            n631 = Fract/Exp String To Number(string=w1069) -> (number=w1067:dbl)  [unwired: 3 in, 1 out]
                            n632 = call "SaveDataFile.vi"("Data Array"=w1089, "Temperature"=w1063, "Channel Number"=w1072, "Humidity"=w1067, "Array Titles"="Voltage[V]\tCapacitance[pF]\tResistance[MOhm]", "Strip Segment"="") -> ()  [unwired: 6 in, 4 out]
                          }
                          frame #3 {
                            n633 = global read "QC_MeasurementSetup.vi" "Run Info"() -> (w1105:T12)
                            n634 = local read "CV Test CH"() -> (w1102:i32)
                            n635 = Unbundle By Name(w1105) -> ("CV"=w1103:bool[])
                            n636 = Replace Array Subset(array=w1103, new element=TRUE ("new element/subarray"), index=w1102) -> (w1104:bool[])
                            n637 = Bundle By Name(cluster=w1105, "CV"=w1104) -> (w1106:T12)
                            n638 = global write "QC_MeasurementSetup.vi" "Run Info"(w1106) -> ()
                          }
                        }
                      }
                    }
                  }
                }
                "CV Test CH" <- w733
              }
            }
            frame #2 {
              # "Open all channels to finish test."
              n639 = flat-sequence {
                tunnel: [w1109] -> w1107
                tunnel: w1107 -> [w1112]
                frame #0 {
                  # "Open all cahnnels in arduino."
                  n640 = global read "QC_MeasurementSetup.vi" "Hardware Settings"() -> (w1111:T11)
                  n641 = Unbundle By Name(w1111) -> ("Arduino"=w1110:refnum<class "ArduinoControl.lvclass">, "Switching GPIB Address"=w1109:string)
                  n642 = call "ArduinoRead.vi"("Arduino function"=T6."Reset Switches", "ArduinoControl in"=w1110) -> ()  [unwired: 4 in, 6 out]
                }
                frame #1 {
                  w1113 = u16 0 items=["open all channels", "open channels in channel list", "close channels in channel list"] ("open/close (open all:0)")
                  # "Open all channels in Keithley"
                  n643 = call "Keith 7002 Open/Close Chan.vi"("GPIB address"=w1112, "open/close (open all:0)"=w1113) -> ()  [unwired: 2 in, 1 out]
                }
              }
            }
          }
        }
      }
    }
    frame #4 {
      # "LCS Test code. Checks to see if the LCS test is to be perfromed."
      n644 = local read "Abort Test"() -> (w1120:bool)
      n645 = global read "QC_MeasurementSetup.vi" "Run Info"() -> (w1123:T12)
      n646 = Unbundle By Name(w1123) -> ("No. of Ch."=w1121:u16, "LCS Test?"=w1115:bool, "Sensor Serials"=w1122:string[], "No. of Sensors"=w1119:i32)
      n647 = Not(x=w1120) -> (.not. x?=w1116:bool)
      n648 = Not Equal To 0?(x=w1119) -> (x != 0?=w1114:bool)
      n649 = Build Array(w1116, w1115, w1114) -> (w1117:bool[])
      n650 = And Array Elements(Boolean array=w1117) -> (logical AND=w1118:bool)
      n651 = case shown="True" w1118 {
        tunnel: w1122 -> [_ w1125]
        tunnel: w1121 -> [_ w1124]
        frame False {
        }
        frame True {
          n652 = stacked-sequence {
            tunnel: w1125 -> [w1129 w1256 w1583]
            tunnel: w1124 -> [w1127 w1255 w1581]
            frame #0 {
              # "Setup Page. Initializes all of the variables"
              n653 = flat-sequence {
                tunnel: [w1134] -> w1128
                tunnel: w1127 -> [w1134]
                tunnel: w1129 -> [w1176]
                tunnel: w1128 -> [w1177]
                tunnel: [w1174] -> w1126
                tunnel: w1126 -> [w1249]
                frame #0 {
                  w1137 = u32 0 ("Current reading No.")
                  w1146 = FALSE ("Visible")
                  w1143 = ""
                  # "Reset the LCS Data Structure. All IV data is stored in here.\nArray mapping is 1.) Time, 2.) Current, 3.) Temperature\n4.) %RH"
                  # "Set all of the paramaters of the status window to their initial values."
                  # "Setup of the initial front panel parameters."
                  # "Initialize the plot scale settings."
                  n654 = global read "QC_MeasurementSetup.vi" "Current Stability Measurement Parameters"() -> (w1148:T8)
                  n655 = Build Array("nanoAmps", "microAmps", "milliAmps") -> (w1155:string[])
                  n656 = Initialize Array(cluster{dbl[], dbl[]} {[], []}, 24 ("dimension size")) -> (→"LCS Graph":cluster{dbl[], dbl[]}[])
                  n657 = property on="LCS Iscale" class="Enum (strict)"("Strings []"=w1155) -> ()  [unwired: 2 in, 2 out]
                  n658 = Unbundle By Name(w1148) -> ("Ramp up steps [V]"=w1130:dbl, "Ramp up Interval [s]"=w1131:u32, "Voltage [V]"=→"LCS Test Volts [V]":dbl, "Measurement Interval [s]"=→"LCS Measurement Interval":i32, "Number of Steps"=→"LCS No of steps":i32, "Test Duration"=→"LCS Test Duration":u32, "Norm. to Temp."=→"Norm. to Temp. [°C]":dbl)
                  n659 = local write "LCS Iscale"(0) -> ()
                  n660 = property on="LCS Bias On/Off:" class="Bool (strict)"("Blinking"=w1146) -> ()  [unwired: 2 in, 2 out]
                  n661 = property on="LCS Graph" class="XYGraph (strict)"() -> ("XScale.Mapping Mode"=w1158:u8, "YScale.Mapping Mode"=w1159:u8)  [unwired: 2 in, 2 out]
                  n662 = local write "Test Control"(T4."LCS Test" ("Test Control")) -> ()
                  n663 = call "TestData.vi"("Action"=enum16{"Reset", "Write Element", "Read Array"}."Reset") -> ("Data OUT"=→"LCS Data":cluster{dbl[], dbl[], dbl[], dbl[], dbl[]}[])  [unwired: 9 in, 1 out]
                  n664 = Multiply(x=w1159, y=2) -> (x*y=w1157:i32)
                  n665 = local write "LCS Step Size [V] IN"(w1130) -> ()
                  n666 = local write "LCS Step Interval [s] IN"(w1131) -> ()
                  n667 = Add(x=w1158, y=w1157) -> (x+y=w1138:i32)
                  n668 = local write "LCS Scales"(w1138) -> ()
                  "LCS Bias On/Off:" <- w1146
                  "LCS Sensor No.:" <- w1143
                  "LCS Test Channel:" <- w1143
                  "LCS Last reading at:" <- w1143
                  "LCS STATUS" <- "INITIALISING LCS RUN"
                  "LCS Time Initiated:" <- w1143
                  "Time Remaining" <- w1137
                  "Time Elapsed" <- w1137
                  "LCS Current reading No." <- w1137
                  "LCS Current Volts:" <- 0.0 ("Current Volts:")
                }
                frame #1 {
                  # "SubVI to obtain Date/Time in\nstandard DB format independently\nof the OS language"
                  # "Perform all of the Arduino pre-switching."
                  n669 = call "GetDateTimeDBFormat.vi"() -> ("Time in 24h format, e.g. 13:40:54"=w1166:string, "Abbreviated Date, e.g. 13 Nov 2020"=w1165:string)  [unwired: 10 in]
                  n670 = global read "QC_MeasurementSetup.vi" "Hardware Settings"() -> (w1178:T11)
                  n671 = global read "QC_MeasurementSetup.vi" "Run Info"() -> (w1173:T12)
                  n672 = Unbundle By Name(w1178) -> ("Arduino"=w1179:refnum<class "ArduinoControl.lvclass">, "Supply"=w1174:refnum<class "SupplyControl.lvclass">, "Volt Name"=w1169:string, "SMU Name"=w1168:string)
                  n673 = Concatenate Strings(w1169, "," ("string"), w1168) -> (w1170:string)
                  n674 = Unbundle By Name(w1173) -> ("Arduino DP Map"=w1175:string[])
                  n675 = Bundle By Name(cluster=w1173, "Instruments"=w1170, "Test Date"=w1165, "Test Time"=w1166, "Current Test"="Stability") -> (w1167:T12)
                  n676 = local write "LCS Time Initiated:"(w1166) -> ()
                  n677 = global write "QC_MeasurementSetup.vi" "Run Info"(w1167) -> ()
                  n678 = flat-sequence {
                    tunnel: w1179 -> [w1184]
                    tunnel: [w1183] -> w1164
                    tunnel: [w1182] -> w1163
                    tunnel: [w1181] -> w1162
                    tunnel: w1175 -> [w1181]
                    tunnel: w1164 -> [w1190]
                    tunnel: w1163 -> [w1188]
                    tunnel: w1162 -> [w1187]
                    tunnel: [w1187] -> w1161
                    tunnel: [w1186] -> w1160
                    tunnel: w1177 -> [w1195]
                    tunnel: w1176 -> [w1196]
                    tunnel: w1161 -> [w1192]
                    tunnel: w1160 -> [w1191]
                    frame #0 {
                      # "Reset all switches"
                      n679 = call "ArduinoRead.vi"("Arduino function"=T6."Reset Switches", "ArduinoControl in"=w1184) -> ("error out"=w1182:errorcluster, "ArduinoControl out"=w1183:refnum<class "ArduinoControl.lvclass">)  [unwired: 4 in, 4 out]
                    }
                    frame #1 {
                      # "Perform Pre-Switching for IV. SMU Hi is already connected to the sensor boards by default. Switch the SMU Lo and LCR Lo to low of signla boards (DP 13). Switch Hi of LCR to protection cap \n (DP 6)."
                      n680 = call "ArduinoRead.vi"("Command String"="11,12,13,", "Arduino function"=T6."Close Switch", "error in (no error)"=w1188, "ArduinoControl in"=w1190) -> ("ArduinoControl out"=w1186:refnum<class "ArduinoControl.lvclass">)  [unwired: 2 in, 5 out]
                    }
                    frame #2 {
                      w1194 = 8
                      # "Close the HV relays for sensors which are present (a DB serial number was entered). \nHas to be done in increments due to the 64 byte limit of the Arduino serial buffer."
                      n681 = Quotient & Remainder(x=w1195, y=w1194) -> (floor(x/y)=w1193:i32)  [unwired: 1 out]
                      n682 = for {
                        N: w1193 -> [_]
                        tunnel: w1194 -> [w1202]
                        tunnel: w1196 -> [w1204]
                        tunnel: w1192 -> [w1201]
                        tunnel: w1191 -> [w1199]
                        i -> [w1203]
                        n683 = for {
                          N: w1202 -> [_]
                          tunnel: w1204 -> [w1212]
                          tunnel: w1203 -> [w1215]
                          tunnel: w1202 -> [w1214]
                          shift-right: [w1205] -> w1198
                          shift-left: "" -> [w1208]
                          tunnel: w1201 -> [w1207]
                          i -> [w1213]
                          n684 = Multiply(x=w1214, y=w1215) -> (x*y=w1216:i32)
                          n685 = Add(x=w1216, y=w1213) -> (x+y=w1206:i32)
                          n686 = Index Array(array=w1212, index=w1206) -> (element=w1210:string)
                          n687 = Not Equal?(x=w1210, y="") -> (x != y?=w1211:bool)
                          n688 = case shown="False" w1211 {
                            tunnel: w1208 -> [w1217 w1221]
                            tunnel: w1207 -> [_ w1223]
                            tunnel: w1206 -> [_ w1222]
                            tunnel: [w1217 w1218] -> w1205
                            frame False {
                            }
                            frame True {
                              n689 = Index Array(array=w1223, index=w1222) -> (element=w1219:string)
                              n690 = Concatenate Strings(w1221, w1219, "," ("string")) -> (w1218:string)
                            }
                          }
                        }
                        n691 = call "ArduinoRead.vi"("Command String"=w1198, "Arduino function"=T6."Close Switch", "ArduinoControl in"=w1199) -> ()  [unwired: 3 in, 6 out]
                      }
                    }
                  }
                }
                frame #2 {
                  # "Ramp up the Voltage"
                  n692 = global read "QC_MeasurementSetup.vi" "Current Stability Measurement Parameters"() -> (w1234:T8)
                  n693 = global read "InstrumentSetup.vi" "Keithley 2410 Configurations"() -> (w1231:T16)
                  n694 = global read "QC_MeasurementSetup.vi" "Run Info"() -> (w1233:T12)
                  n695 = local read "LCS Step Interval [s] IN"() -> (w1236:i32)
                  n696 = call-dynamic "Supply_Reset.vi"("SupplyControl in"=w1249) -> ("error out"=w1243:errorcluster, "SupplyControl out"=w1244:refnum<class "SupplyControl.lvclass">)  [unwired: 9 in]
                  n697 = Unbundle By Name(w1233) -> ("No. of Sensors"=w1224:i32)
                  "Number of Sensors" <- w1224
                  n698 = local read "LCS Step Size [V] IN"() -> (w1238:dbl)
                  n699 = Unbundle By Name(w1234) -> ("Current Limit [µA]"=w1232:dbl)
                  n700 = call-dynamic "Supply_Init.vi"("error in (no error)"=w1243, "SupplyControl in"=w1244) -> ("error out"=w1228:errorcluster, "SupplyControl out"=w1229:refnum<class "SupplyControl.lvclass">)  [unwired: 8 in]
                  n701 = Multiply(x=w1232, y=w1224) -> (x*y=w1227:dbl)
                  n702 = Multiply(x=w1227, y=1e-06) -> (x*y=w1225:dbl)
                  n703 = Bundle By Name(cluster=w1231, "Current Limit"=w1225) -> (w1230:T16)
                  n704 = local read "LCS Test Volts [V]"() -> (w1239:dbl)
                  n705 = Multiply(x=w1236, y=1000) -> (x*y=w1237:i32)
                  n706 = call-dynamic "Supply_Arm.vi"("error in (no error)"=w1228, "SupplyControl in"=w1229) -> ("error out"=w1241:errorcluster, "SupplyControl out"=w1242:refnum<class "SupplyControl.lvclass">)  [unwired: 8 in]
                  n707 = call "SupplyRamp.vi"("error in"=w1241, "Requested Voltage"=w1239, "Step Size"=w1238, "Step Delay"=w1237, "Supply IN"=w1242, "Starting Voltage"=0.0) -> ("Compliance exceeded"=w1245:bool, "Current Voltage"=w1248:dbl)  [unwired: 2 in, 2 out]
                  n708 = global write "InstrumentSetup.vi" "Keithley 2410 Configurations"(w1230) -> ()
                  n709 = local write "LCS Current Volts:"(w1248) -> ()
                  n710 = case shown="False" w1245 {
                    selector: w1245 -> [w1250 w1252]
                    frame False {
                      n711 = property on="LCS Bias On/Off:" class="Bool (strict)"("Blinking"=w1250) -> ()  [unwired: 2 in, 2 out]
                    }
                    frame True {
                      n712 = property on="LCS Bias On/Off:" class="Bool (strict)"("Blinking"=w1252) -> ()  [unwired: 2 in, 2 out]
                      n713 = local write "LCS STATUS"("Run aborted, compliance exceeded." ("STATUS 1")) -> ()
                    }
                  }
                  n714 = local write "LCS Bias On/Off:"(TRUE ("IV Bias On/Off:")) -> ()
                  n715 = local write "LCS STATUS"("Biasing Sensors..." ("STATUS 1")) -> ()
                }
              }
            }
            frame #1 {
              # "For even time array."
              # "Get the initial time."
              # "While we have not hit the elapsed time and the abort button has not been pressed, continue to measure."
              n716 = Get Date/Time In Seconds() -> (seconds since 1Jan1904=w1257:timestamp)
              n717 = To Double Precision Float(number=w1257) -> (double precision float=w1254:dbl)
              n718 = while {
                tunnel: w1254 -> [w1278]
                tunnel: w1256 -> [w1276]
                tunnel: w1255 -> [w1275]
                shift-right: [w1262] -> _
                shift-left: 0.0 -> [w1265]
                i -> [w1268]
                stop <- w1272 continue-if-true
                n719 = flat-sequence {
                  tunnel: w1265 -> [w1279]
                  tunnel: w1275 -> [w1280]
                  tunnel: w1276 -> [w1281]
                  tunnel: w1278 -> [w1282]
                  tunnel: [w1282] -> w1261
                  tunnel: [w1281] -> w1260
                  tunnel: [w1280] -> w1259
                  tunnel: [w1279] -> w1258
                  tunnel: [w1299] -> w1277
                  tunnel: w1268 -> [w1303]
                  tunnel: [w1298] -> w1274
                  tunnel: [w1283] -> w1264
                  tunnel: w1261 -> [w1299]
                  tunnel: w1260 -> [w1309]
                  tunnel: w1259 -> [w1310]
                  tunnel: w1258 -> [w1284]
                  tunnel: w1277 -> [w1498]
                  tunnel: w1274 -> [w1493]
                  tunnel: [w1498] -> w1273
                  tunnel: [w1495] -> w1271
                  tunnel: [w1494] -> w1270
                  tunnel: [w1493] -> w1269
                  tunnel: [w1491] -> w1266
                  tunnel: w1264 -> [w1490]
                  tunnel: [w1490] -> w1263
                  tunnel: w1273 -> [w1508]
                  tunnel: [w1515] -> w1272
                  tunnel: w1271 -> [w1522]
                  tunnel: w1270 -> [w1521]
                  tunnel: w1269 -> [w1520]
                  tunnel: w1266 -> [w1504]
                  tunnel: w1263 -> [w1507]
                  tunnel: [w1505] -> w1262
                  frame #0 {
                  }
                  frame #1 {
                    # "Coversion from mV\nto nA is *1000 when divided\nby 1MOhm."
                    # "Iterate throught the channels and check if they are connected.\nIf yes, perform a voltage measurement. If not do nothing. \nUpdate the T/RH plot before performing the measurement loop."
                    n720 = global read "QC_MeasurementSetup.vi" "Hardware Settings"() -> (w1307:T11)
                    n721 = local read "Temperature Array"() -> (w1293:dbl[])
                    n722 = local read "Humidity Array"() -> (w1292:dbl[])
                    n723 = local read "Time"() -> (w1291:u32[])
                    n724 = Unbundle By Name(w1307) -> ("Switching GPIB Address"=w1305:string, "Voltmeter Visa"=w1306:refnum<visa-resource-name>, "Arduino"=w1302:refnum<class "ArduinoControl.lvclass">, "Supply"=w1297:refnum<class "SupplyControl.lvclass">)
                    n725 = call "ArduinoRead.vi"("Arduino function"=T6."T/RH", "ArduinoControl in"=w1302) -> ("rel. Humidity [%]"=w1301:dbl, "Temperature [°C]"=w1300:dbl)  [unwired: 4 in, 4 out]
                    n726 = local write "Temp. [°C]"(w1300) -> ()
                    n727 = local write "RH [%]"(w1301) -> ()
                    n728 = call "StopWatch.vi"("Action"=enum16{"Start", "Stop", "Read", "Reset"}."Read") -> ("Time elapsed"=w1288:u32)  [unwired: 4 out]
                    n729 = local write "LCS STATUS"("Measuring Leakage Current." ("LCS STATUS")) -> ()
                    n730 = Build Array (concatenate)(w1293, w1300) -> (w1286:dbl[])
                    n731 = Build Array (concatenate)(w1292, w1301) -> (w1287:dbl[])
                    n732 = Build Array (concatenate)(w1291, w1288) -> (w1285:u32[])
                    n733 = local write "Run time"(w1288) -> ()
                    n734 = local read "LCS Data"() -> (w1304:cluster{dbl[], dbl[], dbl[], dbl[], dbl[]}[])
                    n735 = local write "Temperature Array"(w1286) -> ()
                    n736 = Bundle(w1285, w1286) -> (w1295:cluster{u32[], dbl[]})  [unwired: 1 in]
                    n737 = Bundle(w1285, w1287) -> (w1294:cluster{u32[], dbl[]})  [unwired: 1 in]
                    n738 = local write "Humidity Array"(w1287) -> ()
                    n739 = local write "Time"(w1285) -> ()
                    n740 = Build Array(w1295, w1294) -> (w1290:cluster{u32[], dbl[]}[])
                    n741 = local write "TGraph"(w1290) -> ()
                    n742 = for {
                      N: w1310 -> [_]
                      tunnel: w1309 -> [w1314] mode=indexing
                      tunnel: w1306 -> [w1323]
                      tunnel: w1305 -> [w1322]
                      tunnel: w1300 -> [w1321]
                      tunnel: w1301 -> [w1320]
                      shift-right: [w1316] -> w1298
                      shift-left: w1304 -> [w1319]
                      tunnel: w1299 -> [w1318]
                      tunnel: w1303 -> [w1317]
                      tunnel: w1297 -> [w1315]
                      tunnel: w1284 -> [w1312]
                      tunnel: [w1311] -> w1283
                      i -> [w1313]
                      n743 = Not Equal?(x=w1314, y="") -> (x != y?=w1325:bool)
                      n744 = case shown="True" w1325 {
                        tunnel: w1314 -> [_ w1370]
                        tunnel: w1313 -> [_ w1364]
                        tunnel: w1323 -> [_ w1363]
                        tunnel: w1322 -> [_ w1362]
                        tunnel: w1321 -> [_ w1369]
                        tunnel: w1320 -> [_ w1368]
                        tunnel: w1319 -> [w1327 w1367]
                        tunnel: w1318 -> [_ w1366]
                        tunnel: w1317 -> [_ w1365]
                        tunnel: [w1327 w1361] -> w1316
                        tunnel: w1315 -> [_ w1354]
                        tunnel: w1314 -> [_ w1351]
                        tunnel: w1313 -> [_ w1349]
                        tunnel: w1312 -> [w1326 w1333]
                        tunnel: [w1326 w1328] -> w1311
                        frame False {
                        }
                        frame True {
                          n745 = Increment(x=w1349) -> (x+1=w1334:i32)
                          n746 = flat-sequence {
                            tunnel: w1370 -> [w1396]
                            tunnel: w1364 -> [w1395]
                            tunnel: w1362 -> [w1394]
                            tunnel: [w1393] -> w1348
                            tunnel: w1369 -> [w1393]
                            tunnel: [w1392] -> w1346
                            tunnel: w1368 -> [w1392]
                            tunnel: [w1391] -> w1344
                            tunnel: w1367 -> [w1391]
                            tunnel: w1366 -> [w1390]
                            tunnel: [w1388] -> w1342
                            tunnel: w1364 -> [w1388]
                            tunnel: [w1387] -> w1340
                            tunnel: w1363 -> [w1387]
                            tunnel: [w1386] -> w1338
                            tunnel: [w1385] -> w1336
                            tunnel: w1362 -> [w1385]
                            tunnel: w1351 -> [_]
                            tunnel: w1333 -> [w1371]
                            tunnel: [w1371] -> w1332
                            tunnel: w1348 -> [w1405]
                            tunnel: [w1405] -> w1347
                            tunnel: w1346 -> [w1404]
                            tunnel: [w1404] -> w1345
                            tunnel: w1344 -> [w1403]
                            tunnel: [w1403] -> w1343
                            tunnel: w1342 -> [w1402]
                            tunnel: [w1402] -> w1341
                            tunnel: w1340 -> [w1401]
                            tunnel: [w1401] -> w1339
                            tunnel: w1338 -> [w1400]
                            tunnel: [w1400] -> w1337
                            tunnel: w1336 -> [w1399]
                            tunnel: [w1399] -> w1335
                            tunnel: w1332 -> [w1397]
                            tunnel: [w1397] -> w1331
                            tunnel: w1347 -> [w1423]
                            tunnel: w1345 -> [w1432]
                            tunnel: w1343 -> [w1430]
                            tunnel: w1365 -> [w1412]
                            tunnel: w1341 -> [w1415]
                            tunnel: w1339 -> [w1424]
                            tunnel: w1337 -> [w1427]
                            tunnel: [w1427] -> w1360
                            tunnel: w1335 -> [w1426]
                            tunnel: [w1426] -> w1359
                            tunnel: [w1425] -> w1358
                            tunnel: [w1419] -> w1355
                            tunnel: [w1415] -> w1352
                            tunnel: w1331 -> [w1406]
                            tunnel: [w1406] -> w1330
                            tunnel: w1360 -> [w1439]
                            tunnel: w1359 -> [w1438]
                            tunnel: w1358 -> [w1435]
                            tunnel: [w1439] -> w1357
                            tunnel: [w1438] -> w1356
                            tunnel: w1355 -> [w1437]
                            tunnel: w1354 -> [w1436]
                            tunnel: [w1435] -> w1353
                            tunnel: w1352 -> [w1434]
                            tunnel: w1330 -> [w1433]
                            tunnel: [w1433] -> w1329
                            tunnel: [w1485] -> w1361
                            tunnel: w1357 -> [w1487]
                            tunnel: w1356 -> [w1486]
                            tunnel: w1353 -> [w1485]
                            tunnel: w1329 -> [w1483]
                            tunnel: [w1483] -> w1328
                            frame #0 {
                              w1373 = u16 2 items=["open all channels", "open channels in channel list", "close channels in channel list"] ("open/close (open all:0)")
                              # "Set parameters and switch voltmeter to sensor."
                              n747 = Get Date/Time In Seconds() -> (seconds since 1Jan1904=w1384:timestamp)
                              n748 = local read "LCS Test Duration"() -> (w1380:i32)
                              n749 = To Double Precision Float(number=w1384) -> (double precision float=w1389:dbl)
                              n750 = Build Array(w1395) -> (w1372:i32[])
                              n751 = local write "LCS Sensor No.:"(w1396) -> ()
                              n752 = call "StopWatch.vi"("Action"=enum16{"Start", "Stop", "Read", "Reset"}."Read") -> ("Time paused"=w1379:u32)  [unwired: 4 out]
                              n753 = Get Date/Time String(date format (0)=enum16{"short", "long", "abbreviated"}."abbreviated", want seconds? (F)=TRUE) -> (time string=w1382:string)  [unwired: 1 in, 1 out]
                              n754 = call "ChannelListGenerator.vi"("Card Type"=enum16{"7036", "7054"}."7036", "Channels"=w1372) -> ("Channel List"=w1386:T15)  [unwired: 9 in]
                              n755 = Add(x=w1380, y=w1379) -> (x+y=w1376:u32)
                              n756 = Subtract(x=w1389, y=w1390) -> (x-y=w1375:dbl)
                              n757 = local write "LCS Last reading at:"(w1382) -> ()
                              n758 = Subtract(x=w1376, y=w1375) -> (x-y=w1377:dbl)
                              n759 = local write "Time Remaining"(w1377) -> ()
                              n760 = local write "Time Elapsed"(w1375) -> ()
                              n761 = call "Keith 7002 Open/Close Chan.vi"("GPIB address"=w1394, "open/close (open all:0)"=w1373, "channel list"=w1386) -> ()  [unwired: 1 in, 1 out]
                            }
                            frame #1 {
                              n762 = Wait (ms)(milliseconds to wait=u32 500) -> ()  [unwired: 1 out]
                            }
                            frame #2 {
                              w1414 = enum16{"Reset", "Write Element", "Read Array"}."Write Element" ("Action")
                              # "Make a voltage measurement, measure the \ncurrent to check for compliance.\n (Need to add voltage measurement)."
                              n763 = local read "Norm. to Temp. [°C]"() -> (w1421:dbl)
                              n764 = local read "LCS Current Limit [µA]"() -> (w1420:dbl)
                              n765 = call-poly <instrlib>:"Read.vi"("VISA resource name"=w1424) -> ("Measurement"=w1411:dbl)  [unwired: 8 in, 2 out]
                              n766 = Multiply(x=1000.0, y=w1411) -> (x*y=w1413:dbl)
                              n767 = call "TestData.vi"("Reading No."=w1412, "Action"=w1414, "Test No."=w1415, "Array No."=u32 2, 10:"Data IN"=w1423, 11:"Data IN"=w1430) -> ("Data OUT"=w1407:cluster{dbl[], dbl[], dbl[], dbl[], dbl[]}[])  [unwired: 4 in, 1 out]
                              n768 = call "TestData.vi"("Reading No."=w1412, "Action"=w1414, "Test No."=w1415, "Array No."=u32 3, 10:"Data IN"=w1432, 11:"Data IN"=w1407) -> ("Data OUT"=w1429:cluster{dbl[], dbl[], dbl[], dbl[], dbl[]}[])  [unwired: 4 in, 1 out]
                              n769 = call "TestData.vi"("Reading No."=w1412, "Action"=w1414, "Test No."=w1415, "Array No."=u32 0, 10:"Data IN"=w1406, 11:"Data IN"=w1429) -> ("Data OUT"=w1417:cluster{dbl[], dbl[], dbl[], dbl[], dbl[]}[])  [unwired: 4 in, 1 out]
                              n770 = call "TestData.vi"("Reading No."=w1412, "Action"=w1414, "Test No."=w1415, "Array No."=u32 4, 10:"Data IN"=w1413, 11:"Data IN"=w1417) -> ("Data OUT"=w1416:cluster{dbl[], dbl[], dbl[], dbl[], dbl[]}[])  [unwired: 4 in, 1 out]
                              n771 = call "GetNormCurrent.vi"("Norm. to temperature (°C)"=w1421, "Measured temperature (°C)"=w1423, "Measured Current"=w1413) -> ("Normalized current"=w1422:dbl)  [unwired: 7 in, 1 out]
                              n772 = call "TestData.vi"("Reading No."=w1412, "Action"=w1414, "Test No."=w1415, "Array No."=u32 1, 10:"Data IN"=w1422, 11:"Data IN"=w1416) -> ("Data OUT"=w1425:cluster{dbl[], dbl[], dbl[], dbl[], dbl[]}[])  [unwired: 4 in, 1 out]
                              n773 = Greater?(x=w1413, y=w1420) -> (0:w1419:bool)
                            }
                            frame #3 {
                              # "Ramp down and remove the sensor if it exceeds compliance.\nRamp back up and resume the test."
                              n774 = case shown="True" w1437 {
                                tunnel: w1436 -> [_ w1441]
                                tunnel: w1434 -> [_ w1440]
                                frame False {
                                }
                                frame True {
                                n775 = stacked-sequence {
                                tunnel: w1441 -> [w1449 _ _ _ w1479]
                                tunnel: w1440 -> [_ w1454 _ _ _]
                                frame #0 {
                                n776 = local read "LCS Current Volts:"() -> (w1446:dbl)
                                n777 = call "StopWatch.vi"("Action"=enum16{"Start", "Stop", "Read", "Reset"}."Stop") -> ()  [unwired: 5 out]
                                n778 = call "SupplyRamp.vi"("Requested Voltage"=0.0, "Step Size"=10.0, "Step Delay"=u32 10000, "Supply IN"=w1449, "Starting Voltage"=w1446) -> ("Current Voltage"=w1445:dbl)  [unwired: 3 in, 3 out]
                                n779 = local write "LCS Current Volts:"(w1445) -> ()
                                n780 = local write "LCS STATUS"("Complaince exceeded... \nRamping down.") -> ()
                                }
                                frame #1 {
                                n781 = global read "QC_MeasurementSetup.vi" "Hardware Settings"() -> (w1461:T11)
                                n782 = global read "QC_MeasurementSetup.vi" "Run Info"() -> (w1455:T12)
                                n783 = Unbundle By Name(w1455) -> ("Arduino DP Map"=w1462:string[], "Sensor Serials"=w1453:string[])
                                n784 = Unbundle By Name(w1461) -> ("Arduino"=w1460:refnum<class "ArduinoControl.lvclass">)
                                n785 = Replace Array Subset(array=w1453, new element="", index=w1454) -> (w1451:string[])
                                n786 = Index Array(array=w1462, index=w1454) -> (element=w1459:string)
                                n787 = Bundle By Name(cluster=w1455, "Sensor Serials"=w1451) -> (w1450:T12)
                                n788 = Concatenate Strings(w1459, "," ("string")) -> (w1457:string)
                                n789 = global write "QC_MeasurementSetup.vi" "Run Info"(w1450) -> ()
                                n790 = call "ArduinoRead.vi"("Command String"=w1457, "Arduino function"=T6."Open Switch", "ArduinoControl in"=w1460) -> ()  [unwired: 3 in, 6 out]
                                }
                                frame #2 {
                                n791 = global read "InstrumentSetup.vi" "Keithley 2410 Configurations"() -> (w1464:T16)
                                n792 = global read "QC_MeasurementSetup.vi" "Current Stability Measurement Parameters"() -> (w1468:T8)
                                n793 = global read "QC_MeasurementSetup.vi" "Run Info"() -> (w1470:T12)
                                n794 = Unbundle By Name(w1470) -> ("No. of Sensors"=w1469:i32)
                                n795 = Unbundle By Name(w1468) -> ("Current Limit [µA]"=w1467:dbl)
                                n796 = Decrement(x=w1469) -> (x-1=w1466:i32)
                                n797 = Multiply(x=w1467, y=w1466) -> (x*y=w1463:dbl)
                                n798 = local write "Number of Sensors"(w1466) -> ()
                                n799 = Bundle By Name(cluster=w1464, "Current Limit"=w1463) -> (w1465:T16)
                                n800 = global write "InstrumentSetup.vi" "Keithley 2410 Configurations"(w1465) -> ()
                                }
                                frame #3 {
                                n801 = local read "Number of Sensors"() -> (w1472:i32)
                                n802 = Equal?(x=w1472, y=0) -> (x = y?=w1473:bool)
                                n803 = case shown="True" w1473 {
                                frame False {
                                }
                                frame True {
                                n804 = local write "Abort Test"(TRUE) -> ()
                                }
                                }
                                }
                                frame #4 {
                                n805 = local read "LCS Current Volts:"() -> (w1477:dbl)
                                n806 = local read "LCS Test Volts [V]"() -> (w1478:dbl)
                                n807 = call "StopWatch.vi"("Action"=enum16{"Start", "Stop", "Read", "Reset"}."Start") -> ()  [unwired: 5 out]
                                n808 = call "SupplyRamp.vi"("Requested Voltage"=w1478, "Step Size"=10.0, "Step Delay"=u32 10000, "Supply IN"=w1479, "Starting Voltage"=w1477) -> ("Current Voltage"=w1476:dbl)  [unwired: 3 in, 3 out]
                                n809 = local write "LCS STATUS"("Ramping voltage back up." ("LCS STATUS")) -> ()
                                n810 = local write "LCS Current Volts:"(w1476) -> ()
                                }
                                }
                                }
                              }
                            }
                            frame #4 {
                              w1484 = u16 1 items=["open all channels", "open channels in channel list", "close channels in channel list"] ("open/close (open all:0)")
                              # "Wait and open the current channel."
                              n811 = property on="LCS Graph" class="XYGraph (strict)"() -> ("YScale.Mapping Mode"=w1489:u8)  [unwired: 2 in, 2 out]
                              n812 = call "Keith 7002 Open/Close Chan.vi"("GPIB address"=w1486, "open/close (open all:0)"=w1484, "channel list"=w1487) -> ()  [unwired: 1 in, 1 out]
                              n813 = Wait (ms)(milliseconds to wait=u32 50) -> ()  [unwired: 1 out]
                              n814 = property on="LCS Graph" class="XYGraph (strict)"("YScale.Minimum"=w1489) -> ()  [unwired: 2 in, 2 out]
                            }
                          }
                          n815 = Number To Decimal String(number=w1334) -> (decimal integer string=w1350:string)  [unwired: 1 in]
                          n816 = local write "LCS Test Channel:"(w1350) -> ()
                        }
                      }
                    }
                  }
                  frame #2 {
                    # "Update the graph and check if compliance was exceeded."
                    n817 = local write "LCS Data"(w1493) -> ()
                    n818 = local read "LCS Scales"() -> (w1495:T2)
                    n819 = local read "LCS Iscale"() -> (w1494:enum16{"nanoAmps", "microAmps", "milliAmps"})
                    n820 = property on="LCS Graph" class="XYGraph (strict)"() -> ("YScale.Mapping Mode"=w1492:u8)  [unwired: 2 in, 2 out]
                    n821 = local read "LCS Graph"() -> (w1497:cluster{dbl[], dbl[]}[])
                    n822 = local read "LCS Current reading No."() -> (w1491:u32)
                    n823 = call "IVScaleYAxis.vi"("Data IN"=w1493, "Plot In"=w1497, "Y Scale"=w1494) -> ("Plot Out"=w1496:cluster{dbl[], dbl[]}[])  [unwired: 8 in]
                    n824 = property on="LCS Graph" class="XYGraph (strict)"("YScale.Minimum"=w1492) -> ()  [unwired: 2 in, 2 out]
                    n825 = local write "LCS Graph"(w1496) -> ()
                  }
                  frame #3 {
                    # "Increment Time."
                    # "Wait until the measurement interval has been completed and let the \nuse change the graph scales if they want during this time."
                    # "Check if the test should end. Humidity exceeds threshold, test time is over or abort is pressed."
                    n826 = local read "RH [%]"() -> (w1513:dbl)
                    n827 = local read "LCS Test Duration"() -> (w1510:i32)
                    n828 = call "StopWatch.vi"("Action"=enum16{"Start", "Stop", "Read", "Reset"}."Read") -> ("Time paused"=w1509:u32)  [unwired: 4 out]
                    n829 = Greater?(x=w1513, y=10.0) -> (0:w1500:bool)
                    n830 = Add(x=w1510, y=w1509) -> (x+y=w1501:u32)
                    n831 = while {
                      shift-right: [w1557] -> _
                      shift-left: w1522 -> [w1560]
                      shift-right: [w1553] -> _
                      shift-left: w1521 -> [w1561]
                      tunnel: w1520 -> [w1554]
                      tunnel: "Waiting for " -> [w1547]
                      tunnel: " seconds." -> [w1545]
                      tunnel: [w1543] -> w1516
                      tunnel: w1501 -> [w1542]
                      tunnel: w1508 -> [w1540]
                      tunnel: w1504 -> [w1534]
                      tunnel: [w1533] -> w1506
                      tunnel: [w1532] -> w1502
                      stop <- w1548 continue-if-true
                      n832 = local read "LCS Scales"() -> (w1559:T2)
                      n833 = local read "LCS Measurement Interval"() -> (w1533:i32)
                      n834 = local read "LCS Iscale"() -> (w1555:enum16{"nanoAmps", "microAmps", "milliAmps"})
                      n835 = Get Date/Time In Seconds() -> (seconds since 1Jan1904=w1552:timestamp)
                      n836 = To Double Precision Float(number=w1552) -> (double precision float=w1539:dbl)
                      n837 = Wait (ms)(milliseconds to wait=u32 50) -> ()  [unwired: 1 out]
                      n838 = Not Equal?(x=w1560, y=w1559) -> (x != y?=w1558:bool)
                      n839 = Not Equal?(x=w1561, y=w1555) -> (x != y?=w1556:bool)
                      n840 = case shown="False" w1558 {
                        tunnel: w1559 -> [w1569 w1570]
                        tunnel: [w1569 w1570] -> w1557
                        frame False {
                        }
                        frame True {
                          n841 = case shown="\"Log - log\".." w1570 {
                            tunnel: [w1573 1 0 w1578] -> w1572
                            tunnel: [w1573 0 1 w1578] -> w1571
                            frame .."Lin - Lin" {
                              w1573 = 0
                            }
                            frame "Log - Lin" {
                            }
                            frame "Lin - Log" {
                            }
                            frame "Log - log".. {
                              w1578 = 1
                            }
                          }
                          n842 = property on="LCS Graph" class="XYGraph (strict)"("X Scale.Mapping Mode"=w1572) -> ()  [unwired: 2 in, 2 out]
                          n843 = property on="LCS Graph" class="XYGraph (strict)"("Y Scale.Mapping Mode"=w1571, "YScale.Minimum"=w1571) -> ()  [unwired: 2 in, 2 out]
                        }
                      }
                      n844 = case shown="False" w1556 {
                        tunnel: [w1562 w1564] -> w1553
                        tunnel: w1555 -> [w1562 w1564]
                        tunnel: w1554 -> [w1563 w1566]
                        tunnel: [w1563 w1566] -> _
                        frame False {
                        }
                        frame True {
                          n845 = local read "LCS Graph"() -> (w1567:cluster{dbl[], dbl[]}[])
                          n846 = property on="LCS Graph" class="XYGraph (strict)"() -> ("YScale.Mapping Mode"=w1565:u8)  [unwired: 2 in, 2 out]
                          n847 = call "IVScaleYAxis.vi"("Data IN"=w1566, "Plot In"=w1567, "Y Scale"=w1564) -> ("Plot Out"=w1568:cluster{dbl[], dbl[]}[])  [unwired: 8 in]
                          n848 = property on="LCS Graph" class="XYGraph (strict)"("YScale.Minimum"=w1565) -> ()  [unwired: 2 in, 2 out]
                          n849 = local write "LCS Graph"(w1568) -> ()
                        }
                      }
                      n850 = Subtract(x=w1539, y=w1540) -> (x-y=w1532:dbl)
                      n851 = Subtract(x=w1542, y=w1532) -> (x-y=w1541:dbl)
                      n852 = To Long Integer(number=w1532) -> (32bit integer=w1536:i32)
                      n853 = Multiply(x=w1533, y=w1534) -> (x*y=w1537:u32)
                      n854 = local write "Time Remaining"(w1541) -> ()
                      n855 = local write "Time Elapsed"(w1532) -> ()
                      n856 = Subtract(x=w1537, y=w1536) -> (x-y=w1535:u32)
                      n857 = Format Into String(format string="%d", w1535) -> (resulting string=w1546:string)  [unwired: 2 in, 1 out]
                      n858 = local read "Abort Test"() -> (w1543:bool)
                      n859 = Greater Than 0?(x=w1535) -> (x > 0?=w1549:bool)
                      n860 = Concatenate Strings(w1547, w1546, w1545) -> (w1544:string)
                      n861 = Not(x=w1543) -> (.not. x?=w1550:bool)
                      n862 = local write "LCS STATUS"(w1544) -> ()
                      n863 = And(x=w1549, y=w1550) -> (x .and. y?=w1548:bool)
                    }
                    n864 = case shown="True" w1500 {
                      selector: w1500 -> [w1523 _]
                      tunnel: [w1523 w1524] -> w1499
                      frame False {
                      }
                      frame True {
                        n865 = flat-sequence {
                          tunnel: [w1526] -> w1524
                          frame #0 {
                            n866 = Wait (ms)(milliseconds to wait=u32 10000) -> ()  [unwired: 1 out]
                          }
                          frame #1 {
                            # "Humidity debouncing."
                            n867 = global read "QC_MeasurementSetup.vi" "Hardware Settings"() -> (w1531:T11)
                            n868 = Unbundle By Name(w1531) -> ("Arduino"=w1530:refnum<class "ArduinoControl.lvclass">)
                            n869 = call "ArduinoRead.vi"("Arduino function"=T6."T/RH", "ArduinoControl in"=w1530) -> ("rel. Humidity [%]"=w1527:dbl)  [unwired: 4 in, 5 out]
                            n870 = Greater?(x=w1527, y=10.0) -> (0:w1526:bool)
                          }
                        }
                      }
                    }
                    n871 = Greater?(x=w1502, y=w1501) -> (0:w1503:bool)
                    n872 = Build Array(w1516, w1503, w1499) -> (w1514:bool[])
                    n873 = Or Array Elements(Boolean array=w1514) -> (logical OR=w1517:bool)
                    n874 = Not(x=w1517) -> (.not. x?=w1515:bool)
                    n875 = Add(x=w1506, y=w1507) -> (x+y=w1505:dbl)
                  }
                }
                n876 = Increment(x=w1268) -> (x+1=w1267:i32)
                n877 = local write "LCS Current reading No."(w1267) -> ()
              }
            }
            frame #2 {
              # "Ramp down the voltage, and reset all of the switches."
              n878 = flat-sequence {
                tunnel: [w1600] -> w1586
                tunnel: [w1599] -> w1585
                tunnel: [w1598] -> w1584
                tunnel: w1583 -> [w1598]
                tunnel: w1581 -> [w1597]
                tunnel: [w1597] -> w1579
                tunnel: w1586 -> [w1607]
                tunnel: w1585 -> [w1606]
                tunnel: w1584 -> [w1605]
                tunnel: [w1605] -> w1582
                tunnel: [w1604] -> w1580
                tunnel: w1579 -> [w1604]
                tunnel: w1582 -> [w1608]
                tunnel: w1580 -> [w1609]
                frame #0 {
                  # "Ramp down the voltage."
                  n879 = global read "QC_MeasurementSetup.vi" "Hardware Settings"() -> (w1595:T11)
                  n880 = global read "QC_MeasurementSetup.vi" "Current Stability Measurement Parameters"() -> (w1594:T8)
                  n881 = Unbundle By Name(w1595) -> ("Switching GPIB Address"=w1599:string, "Arduino"=w1600:refnum<class "ArduinoControl.lvclass">, "Supply"=w1589:refnum<class "SupplyControl.lvclass">)
                  n882 = Unbundle By Name(w1594) -> ("Ramp down steps [V]"=w1593:dbl)
                  n883 = local read "LCS Current Volts:"() -> (w1592:dbl)
                  n884 = call "SupplyRamp.vi"("Requested Voltage"=0.0, "Step Size"=w1593, "Step Delay"=5000 ("y"), "Supply IN"=w1589, "Starting Voltage"=w1592) -> ("error out"=w1596:errorcluster, "Supply OUT"=w1588:refnum<class "SupplyControl.lvclass">, "Current Voltage"=w1591:dbl)  [unwired: 3 in, 1 out]
                  n885 = local write "LCS Current Volts:"(w1591) -> ()
                  n886 = call-dynamic "Supply_Stby.vi"("error in (no error)"=w1596, "SupplyControl in"=w1588) -> ()  [unwired: 8 in, 2 out]
                }
                frame #1 {
                  w1603 = u16 0 items=["open all channels", "open channels in channel list", "close channels in channel list"] ("open/close (open all:0)")
                  # "Open all channels in the Arduino and the Keithley 7002"
                  n887 = call "ArduinoRead.vi"("Arduino function"=T6."Reset Switches", "ArduinoControl in"=w1607) -> ("error out"=w1602:errorcluster)  [unwired: 4 in, 5 out]
                  n888 = call "Keith 7002 Open/Close Chan.vi"("GPIB address"=w1606, "error in"=w1602, "open/close (open all:0)"=w1603) -> ()  [unwired: 1 in, 1 out]
                }
                frame #2 {
                  # "Check if the test passed or failed for each sensor and save the data."
                  n889 = for {
                    N: w1609 -> [_]
                    tunnel: w1608 -> [w1610] mode=indexing
                    i -> [w1612]
                    n890 = local read "LCS Data"() -> (w1611:cluster{dbl[], dbl[], dbl[], dbl[], dbl[]}[])
                    n891 = Not Equal?(x=w1610, y="") -> (x != y?=w1613:bool)
                    n892 = case shown="True" w1613 {
                      tunnel: w1612 -> [_ w1615]
                      tunnel: w1611 -> [_ w1621]
                      frame False {
                      }
                      frame True {
                        w1630 = enum16{"Reset", "Write Element", "Read Array"}."Read Array" ("Action")
                        # "Need to determine the failure criterion first."
                        n893 = local read "LCS Current reading No."() -> (w1626:u32)
                        n894 = call "TestData.vi"("Action"=w1630, "Test No."=w1615, "Array No."=u32 0, "Data IN"=w1621) -> ("Array OUT"=w1642:dbl[], "Data OUT"=w1648:cluster{dbl[], dbl[], dbl[], dbl[], dbl[]}[])  [unwired: 6 in]
                        n895 = call "ScanFeedback.vi"("Data IN"=w1621, "measurement type"=T7."Stability", "Test No."=w1615) -> ("V depletion"=w1634:dbl)  [unwired: 2 in, 4 out]
                        n896 = call "TestData.vi"("Action"=w1630, "Test No."=w1615, "Array No."=u32 1, "Data IN"=w1648) -> ("Array OUT"=w1624:dbl[], "Data OUT"=w1633:cluster{dbl[], dbl[], dbl[], dbl[], dbl[]}[])  [unwired: 6 in]
                        n897 = Absolute Value(x=w1634) -> (abs(x)=w1637:dbl)
                        n898 = Absolute Value(x=0.0) -> (abs(x)=w1638:dbl)
                        n899 = call "TestData.vi"("Action"=w1630, "Test No."=w1615, "Array No."=u32 2, "Data IN"=w1633) -> ("Array OUT"=w1625:dbl[], "Data OUT"=w1647:cluster{dbl[], dbl[], dbl[], dbl[], dbl[]}[])  [unwired: 6 in]
                        n900 = Less Or Equal?(x=w1637, y=w1638) -> ()  [unwired: 1 out]
                        n901 = call "TestData.vi"("Action"=w1630, "Test No."=w1615, "Array No."=u32 3, "Data IN"=w1647) -> ("Array OUT"=w1631:dbl[], "Data OUT"=w1629:cluster{dbl[], dbl[], dbl[], dbl[], dbl[]}[])  [unwired: 6 in]
                        n902 = global read "QC_MeasurementSetup.vi" "Run Info"() -> (w1620:T12)
                        n903 = call "TestData.vi"("Action"=w1630, "Test No."=w1615, "Array No."=u32 4, "Data IN"=w1629) -> ("Array OUT"=w1628:dbl[])  [unwired: 6 in, 1 out]
                        n904 = Unbundle By Name(w1620) -> ("Stability"=w1617:bool[])
                        n905 = Build Array(w1642, w1625, w1631, w1624, w1628) -> (w1641:dbl[][])
                        n906 = Replace Array Subset(array=w1617, new element=TRUE ("new element/subarray"), index=w1615) -> (w1618:bool[])
                        n907 = Transpose 2D Array(2D array=w1641) -> (transposed array=w1640:dbl[][])
                        n908 = call "ComputeMean.vi"("Array In"=w1625, "No. of Readings"=w1626) -> ("Mean"=w1622:dbl)  [unwired: 9 in]
                        n909 = call "ComputeMean.vi"("Array In"=w1624, "No. of Readings"=w1626) -> ("Mean"=w1623:dbl)  [unwired: 9 in]
                        n910 = Bundle By Name(cluster=w1620, "Stability"=w1618) -> (w1619:T12)
                        n911 = call "SaveDataFile.vi"("Data Array"=w1640, "Temperature"=w1623, "Channel Number"=w1615, "Humidity"=w1622, "Array Titles"="Time[s]\tTemperature[C]\tHumidity[%]\tCurrent[nA]\tShunt_voltage[mV]", "Strip Segment"="") -> ()  [unwired: 6 in, 4 out]
                        n912 = global write "QC_MeasurementSetup.vi" "Run Info"(w1619) -> ()
                      }
                    }
                  }
                }
              }
            }
          }
        }
      }
    }
    frame #5 {
      # "Shut down all of the devices. Note, the SMU is already in standby and is generally left that way so does not need \nto be disconnected."
      n913 = global read "QC_MeasurementSetup.vi" "Hardware Settings"() -> (w1652:T11)
      n914 = Unbundle By Name(w1652) -> ("Arduino"=w1650:refnum<class "ArduinoControl.lvclass">, "Switching GPIB Address"=w1651:string, "Voltmeter Visa"=w1649:refnum<visa-resource-name>)
      n915 = call "ArduinoClose.vi"("ArduinoControl in"=w1650) -> ()  [unwired: 9 in, 2 out]
      n916 = call <instrlib>:"Keith 7002 Close.vi"("GPIB address"=w1651) -> ()  [unwired: 2 in, 1 out]
      n917 = call <instrlib>:"Close.vi"("VISA resource name"=w1649) -> ()  [unwired: 10 in, 1 out]
    }
    frame #6 {
      # "Loop to allow the user to enter comments, view individual plots and in the future, determine if \na test passed or failed."
      n918 = flat-sequence {
        tunnel: ["Review Iscale"] -> w1655
        tunnel: ["Review Scales"] -> w1654
        tunnel: [w1659] -> w1653
        tunnel: w1655 -> [w1679]
        tunnel: w1654 -> [w1678]
        tunnel: w1653 -> [w1677]
        frame #0 {
          w1664 = "none" ("X Scale.Name Label.Text")
          w1675 = "" ("Current Text")
          # "For now these will just show if a \ncertian test was perfromed or not.\nIn the future may add criteria to \nevaluate pass of fail."
          # "Setup tab variables and displays."
          n919 = global read "QC_MeasurementSetup.vi" "Run Info"() -> (w1659:T12)
          n920 = property on="Review Graph" class="XYGraph (strict)"() -> ("XScale.Mapping Mode"=w1669:u8, "YScale.Mapping Mode"=w1670:u8)  [unwired: 2 in, 2 out]
          n921 = Unbundle By Name(w1659) -> ("IV"=→"IV":bool[], "CV"=→"CV":bool[], "Stability"=→"Stability":bool[])
          n922 = local write "End Program"(FALSE ("End Program")) -> ()
          n923 = Build Array("none", "none", "none") -> (w1674:string[])
          n924 = Multiply(x=w1670, y=2) -> (x*y=w1668:i32)
          n925 = local write "Comment Box"(w1675) -> ()
          n926 = local write "Current Text"(w1675) -> ()
          n927 = local write "Test Control"(T1."Test Results" ("Test Control")) -> ()
          n928 = Add(x=w1669, y=w1668) -> (x+y=w1666:i32)
          n929 = property on="Review Graph" class="XYGraph (strict)"("XScale.NameLbl.Text"=w1664, "YScale.NameLbl.Text"=w1664) -> ()  [unwired: 2 in, 2 out]
          n930 = local write "Review Scales"(w1666) -> ()
          n931 = local write "Review Iscale"(0) -> ()
          n932 = property on="Review Iscale" class="Ring (strict)"("Strings []"=w1674) -> ()  [unwired: 2 in, 2 out]
          "Review Graph" <- cluster{dbl[], dbl[]} {[], []}
        }
        frame #1 {
          n933 = while {
            shift-right: [w1686] -> _
            shift-left: "Channel" -> [w1698]
            shift-right: [w1685] -> _
            shift-left: "Test Type" -> [w1697]
            shift-right: [w1683] -> _
            shift-left: w1679 -> [w1696]
            shift-right: [w1688] -> _
            shift-left: w1678 -> [w1695]
            tunnel: w1677 -> [w1682]
            stop <- "End Program" stop-if-true
            # "Loop to get and display individual plots/ add comments."
            n934 = flat-sequence {
              tunnel: [w1711] -> _
              tunnel: w1698 -> [w1711]
              tunnel: w1697 -> [w1710]
              tunnel: w1696 -> [w1702]
              tunnel: w1695 -> [w1701]
              tunnel: [w1704] -> w1694
              tunnel: [w1703] -> w1693
              tunnel: [w1702] -> w1692
              tunnel: [w1701] -> w1691
              tunnel: w1682 -> [w1700]
              tunnel: w1694 -> [w1822]
              tunnel: w1693 -> [w1821]
              tunnel: w1692 -> [w1827]
              tunnel: w1691 -> [w1828]
              tunnel: [w1826] -> w1690
              tunnel: [w1823] -> w1689
              tunnel: [w1822] -> w1687
              tunnel: [w1821] -> w1684
              tunnel: w1690 -> [w1932]
              tunnel: w1689 -> [w1935]
              tunnel: [w1935] -> w1688
              tunnel: [w1934] -> w1686
              tunnel: w1687 -> [w1934]
              tunnel: [w1933] -> w1685
              tunnel: w1684 -> [w1933]
              tunnel: [w1932] -> w1683
              frame #0 {
                # "Check if the user wants to load in a different plot."
                n935 = local read "Test Type"() -> (w1703:u16)
                n936 = local read "Channel"() -> (w1704:u16)
                n937 = Equal?(x=u16 3, y=w1703) -> (x = y?=w1706:bool)
                n938 = Equal?(x=w1704, y=u16 24) -> (x = y?=w1705:bool)
                n939 = Or(x=w1705, y=w1706) -> (x .or. y?=w1709:bool)
                n940 = case shown="False" w1709 {
                  tunnel: w1711 -> [w1714 _]
                  tunnel: w1704 -> [w1717 _]
                  tunnel: w1710 -> [w1715 _]
                  tunnel: w1703 -> [w1713 _]
                  tunnel: w1700 -> [w1712 _]
                  frame False {
                    n941 = Unbundle By Name(w1712) -> ("Data Paths"=w1716:string[][])
                    n942 = Not Equal?(x=w1717, y=w1714) -> (x != y?=w1718:bool)
                    n943 = Not Equal?(x=w1715, y=w1713) -> (x != y?=w1719:bool)
                    n944 = Or(x=w1718, y=w1719) -> (x .or. y?=w1720:bool)
                    n945 = case shown="True" w1720 {
                      tunnel: w1717 -> [_ w1721]
                      tunnel: w1713 -> [_ w1722]
                      tunnel: w1716 -> [_ w1726]
                      frame False {
                      }
                      frame True {
                        n946 = Index Array(array=w1726, index (row)=w1721, index (col)=w1722) -> (element=w1723:string)
                        n947 = Not Equal?(x=w1723, y="") -> (x != y?=w1724:bool)
                        n948 = case shown="True" w1724 {
                          tunnel: w1723 -> [_ w1733]
                          tunnel: w1722 -> [_ w1732]
                          tunnel: w1721 -> [_ w1728]
                          frame False {
                          }
                          frame True {
                            n949 = String To Path(string=w1733) -> (path=w1731:path)
                            "Data Path" <- w1731
                            n950 = local write "Comment Box"("" ("Comment Box")) -> ()
                            n951 = Read from Text File(file (use dialog)=w1731, count=-1) -> (text=→"Current Text":string)  [unwired: 2 in, 3 out]
                            n952 = case shown="1" w1732 {
                              tunnel: w1728 -> [w1736 w1759 w1788]
                              frame 0, Default {
                                n953 = flat-sequence {
                                tunnel: w1736 -> [w1741]
                                tunnel: [w1738] -> w1735
                                tunnel: [w1737] -> w1734
                                tunnel: w1735 -> [w1758]
                                tunnel: w1734 -> [w1757]
                                frame #0 {
                                w1740 = enum16{"Reset", "Write Element", "Read Array"}."Read Array" ("Action")
                                # "Set plot format"
                                n954 = property on="Review Graph" class="XYGraph (strict)"() -> ("YScale.Mapping Mode"=w1746:u8)  [unwired: 2 in, 2 out]
                                n955 = local read "IV Data"() -> (w1743:cluster{dbl[], dbl[], dbl[], dbl[], dbl[]}[])
                                n956 = local write "Review Iscale"(0) -> ()
                                n957 = call "TestData.vi"("Action"=w1740, "Test No."=w1741, "Array No."=u32 1, "Data IN"=w1743) -> ("Array OUT"=w1737:dbl[], "Data OUT"=w1744:cluster{dbl[], dbl[], dbl[], dbl[], dbl[]}[])  [unwired: 6 in]
                                n958 = Build Array("nanoAmps", "microAmps", "milliAmps") -> (w1752:string[])
                                n959 = property on="Review Graph" class="XYGraph (strict)"("XScale.NameLbl.Text"="Voltage (V)" ("X Scale.Name Label.Text"), "YScale.NameLbl.Text"="Current" ("Y Scale.Name Label.Text")) -> ()  [unwired: 2 in, 2 out]
                                n960 = property on="Review Graph" class="XYGraph (strict)"("YScale.Minimum"=w1746) -> ()  [unwired: 2 in, 2 out]
                                n961 = property on="Review Iscale" class="Ring (strict)"("Strings []"=w1752) -> ()  [unwired: 2 in, 2 out]
                                n962 = call "TestData.vi"("Action"=w1740, "Test No."=w1741, "Array No."=u32 0, "Data IN"=w1744) -> ("Array OUT"=w1738:dbl[])  [unwired: 6 in, 1 out]
                                }
                                frame #1 {
                                # "Plot Data"
                                n963 = local read "Review Graph"() -> (w1754:cluster{dbl[], dbl[]})
                                n964 = Absolute Value(x=w1758) -> (abs(x)=w1756:dbl[])
                                n965 = Absolute Value(x=w1757) -> (abs(x)=w1755:dbl[])
                                n966 = Bundle(cluster=w1754, w1756, w1755) -> (w1753:cluster{dbl[], dbl[]})
                                n967 = local write "Review Graph"(w1753) -> ()
                                }
                                }
                              }
                              frame 1 {
                                n968 = flat-sequence {
                                tunnel: w1759 -> [w1773]
                                tunnel: [w1770] -> w1761
                                tunnel: [w1769] -> w1760
                                tunnel: w1761 -> [w1785]
                                tunnel: w1760 -> [w1779]
                                frame #0 {
                                w1772 = enum16{"Reset", "Write Element", "Read Array"}."Read Array" ("Action")
                                # "Set plot format"
                                n969 = property on="Review Graph" class="XYGraph (strict)"() -> ("YScale.Mapping Mode"=w1768:u8)  [unwired: 2 in, 2 out]
                                n970 = local read "CV Data"() -> (w1775:cluster{dbl[], dbl[], dbl[], dbl[], dbl[]}[])
                                n971 = local write "Review Iscale"(0) -> ()
                                n972 = call "TestData.vi"("Action"=w1772, "Test No."=w1773, "Array No."=u32 1, "Data IN"=w1775) -> ("Array OUT"=w1769:dbl[], "Data OUT"=w1776:cluster{dbl[], dbl[], dbl[], dbl[], dbl[]}[])  [unwired: 6 in]
                                n973 = Build Array("1/C^2 [1/nF^2]", "nF", "pF") -> (w1762:string[])
                                n974 = property on="Review Graph" class="XYGraph (strict)"("XScale.NameLbl.Text"="Voltage (V)" ("X Scale.Name Label.Text"), "YScale.NameLbl.Text"="Capacitance" ("Y Scale.Name Label.Text")) -> ()  [unwired: 2 in, 2 out]
                                n975 = property on="Review Graph" class="XYGraph (strict)"("YScale.Minimum"=w1768) -> ()  [unwired: 2 in, 2 out]
                                n976 = property on="Review Iscale" class="Ring (strict)"("Strings []"=w1762) -> ()  [unwired: 2 in, 2 out]
                                n977 = call "TestData.vi"("Action"=w1772, "Test No."=w1773, "Array No."=u32 0, "Data IN"=w1776) -> ("Array OUT"=w1770:dbl[])  [unwired: 6 in, 1 out]
                                }
                                frame #1 {
                                # "Plot Data"
                                n978 = local read "Review Graph"() -> (w1783:cluster{dbl[], dbl[]})
                                n979 = Absolute Value(x=w1779) -> (abs(x)=w1780:dbl[])
                                n980 = Array Size(array=w1779) -> (size(s)=w1781:i32)
                                n981 = Absolute Value(x=w1785) -> (abs(x)=w1784:dbl[])
                                n982 = for {
                                N: w1781 -> [_]
                                tunnel: w1780 -> [w1787] mode=indexing
                                tunnel: [w1786] -> w1778 mode=indexing
                                n983 = formula code="y=1000000./(x*x);"("x"=w1787) -> ("y"=w1786:dbl)
                                }
                                n984 = Bundle(cluster=w1783, w1784, w1778) -> (w1782:cluster{dbl[], dbl[]})
                                n985 = local write "Review Graph"(w1782) -> ()
                                }
                                }
                              }
                              frame 2 {
                                n986 = flat-sequence {
                                tunnel: w1788 -> [w1799]
                                tunnel: [w1796] -> w1790
                                tunnel: [w1795] -> w1789
                                tunnel: w1790 -> [w1812]
                                tunnel: w1789 -> [w1811]
                                frame #0 {
                                w1798 = enum16{"Reset", "Write Element", "Read Array"}."Read Array" ("Action")
                                # "Set plot format"
                                n987 = local read "LCS Data"() -> (w1801:cluster{dbl[], dbl[], dbl[], dbl[], dbl[]}[])
                                n988 = property on="Review Graph" class="XYGraph (strict)"() -> ("YScale.Mapping Mode"=w1794:u8)  [unwired: 2 in, 2 out]
                                n989 = local write "Review Iscale"(0) -> ()
                                n990 = call "TestData.vi"("Action"=w1798, "Test No."=w1799, "Array No."=u32 1, "Data IN"=w1801) -> ("Array OUT"=w1795:dbl[], "Data OUT"=w1802:cluster{dbl[], dbl[], dbl[], dbl[], dbl[]}[])  [unwired: 6 in]
                                n991 = Build Array("nanoAmps", "microAmps", "milliAmps") -> (w1793:string[])
                                n992 = property on="Review Graph" class="XYGraph (strict)"("XScale.NameLbl.Text"="Time (s)" ("X Scale.Name Label.Text"), "YScale.NameLbl.Text"="Current" ("Y Scale.Name Label.Text")) -> ()  [unwired: 2 in, 2 out]
                                n993 = property on="Review Graph" class="XYGraph (strict)"("YScale.Minimum"=w1794) -> ()  [unwired: 2 in, 2 out]
                                n994 = call "TestData.vi"("Action"=w1798, "Test No."=w1799, "Array No."=u32 0, "Data IN"=w1802) -> ("Array OUT"=w1796:dbl[])  [unwired: 6 in, 1 out]
                                n995 = property on="Review Iscale" class="Ring (strict)"("Strings []"=w1793) -> ()  [unwired: 2 in, 2 out]
                                }
                                frame #1 {
                                # "Plot Data"
                                n996 = local read "Review Graph"() -> (w1808:cluster{dbl[], dbl[]})
                                n997 = Absolute Value(x=w1812) -> (abs(x)=w1810:dbl[])
                                n998 = Absolute Value(x=w1811) -> (abs(x)=w1809:dbl[])
                                n999 = Bundle(cluster=w1808, w1810, w1809) -> (w1807:cluster{dbl[], dbl[]})
                                n1000 = local write "Review Graph"(w1807) -> ()
                                }
                                }
                              }
                            }
                          }
                        }
                      }
                    }
                  }
                  frame True {
                    w1817 = "none" ("X Scale.Name Label.Text")
                    w1814 = "" ("Current Text")
                    n1001 = property on="Review Graph" class="XYGraph (strict)"("XScale.NameLbl.Text"=w1817, "YScale.NameLbl.Text"=w1817) -> ()  [unwired: 2 in, 2 out]
                    n1002 = Build Array("none", "none", "none") -> (w1815:string[])
                    n1003 = local write "Comment Box"(w1814) -> ()
                    n1004 = local write "Current Text"(w1814) -> ()
                    n1005 = property on="Review Iscale" class="Ring (strict)"("Strings []"=w1815) -> ()  [unwired: 2 in, 2 out]
                    n1006 = local write "Review Graph"(cluster{dbl[], dbl[]} {[], []}) -> ()
                    n1007 = local write "Review Iscale"(0) -> ()
                  }
                }
              }
              frame #1 {
                # "Check if the user wants to change the axes properties"
                n1008 = case shown="1" w1821 {
                  tunnel: w1827 -> [w1844 w1874 w1903 w1930]
                  tunnel: [w1842 w1870 w1900 w1930] -> w1826
                  tunnel: w1822 -> [w1839 w1872 w1902 _]
                  frame 0, Default {
                    n1009 = local read "Review Graph"() -> (w1843:cluster{dbl[], dbl[]})
                    n1010 = local read "Review Iscale"() -> (w1841:u16)
                    n1011 = Not Equal?(x=w1841, y=w1844) -> (x != y?=w1845:bool)
                    n1012 = case shown="False" w1845 {
                      tunnel: w1841 -> [w1847 w1858]
                      tunnel: w1843 -> [w1846 w1857]
                      tunnel: [w1847 w1858] -> w1842
                      tunnel: [w1846 w1856] -> w1840
                      tunnel: w1839 -> [_ w1854]
                      frame False {
                      }
                      frame True {
                        n1013 = local read "IV Data"() -> (w1855:cluster{dbl[], dbl[], dbl[], dbl[], dbl[]}[])
                        n1014 = Unbundle(w1857) -> (w1849:dbl[])  [unwired: 1 out]
                        n1015 = call "TestData.vi"("Test No."=w1854, "Array No."=u32 1, "Data IN"=w1855) -> ("Array OUT"=w1852:dbl[])  [unwired: 7 in, 1 out]
                        n1016 = property on="Review Graph" class="XYGraph (strict)"() -> ("YScale.Mapping Mode"=w1859:u8)  [unwired: 2 in, 2 out]
                        n1017 = Absolute Value(x=w1852) -> (abs(x)=w1851:dbl[])
                        n1018 = case shown="2" w1858 {
                          tunnel: w1851 -> [w1861 w1863 w1867]
                          tunnel: [w1861 w1862 w1866] -> w1850
                          tunnel: w1849 -> [w1860 w1865 w1869]
                          tunnel: [w1860 w1865 w1869] -> w1848
                          frame 0, Default {
                          }
                          frame 1 {
                            n1019 = Divide(x=w1863, y=1000.0) -> (x/y=w1862:dbl[])
                          }
                          frame 2 {
                            n1020 = Divide(x=w1867, y=1000000.0) -> (x/y=w1866:dbl[])
                          }
                        }
                        n1021 = property on="Review Graph" class="XYGraph (strict)"("YScale.Minimum"=w1859) -> ()  [unwired: 2 in, 2 out]
                        n1022 = Bundle(w1848, w1850) -> (w1856:cluster{dbl[], dbl[]})  [unwired: 1 in]
                      }
                    }
                    n1023 = local write "Review Graph"(w1840) -> ()
                  }
                  frame 1 {
                    n1024 = local read "Review Graph"() -> (w1875:cluster{dbl[], dbl[]})
                    n1025 = local read "Review Iscale"() -> (w1873:u16)
                    n1026 = Not Equal?(x=w1873, y=w1874) -> (x != y?=w1876:bool)
                    n1027 = case shown="False" w1876 {
                      tunnel: w1875 -> [w1877 w1884]
                      tunnel: [w1878 w1888] -> w1870
                      tunnel: w1873 -> [w1878 w1888]
                      tunnel: w1872 -> [_ w1887]
                      tunnel: [w1877 w1879] -> w1871
                      frame False {
                      }
                      frame True {
                        n1028 = local read "CV Data"() -> (w1886:cluster{dbl[], dbl[], dbl[], dbl[], dbl[]}[])
                        n1029 = Unbundle(w1884) -> (w1881:dbl[])  [unwired: 1 out]
                        n1030 = call "TestData.vi"("Test No."=w1887, "Array No."=u32 1, "Data IN"=w1886) -> ("Array OUT"=w1882:dbl[])  [unwired: 7 in, 1 out]
                        n1031 = Absolute Value(x=w1882) -> (abs(x)=w1883:dbl[])
                        n1032 = property on="Review Graph" class="XYGraph (strict)"() -> ("YScale.Mapping Mode"=w1889:u8)  [unwired: 2 in, 2 out]
                        n1033 = case shown="2" w1888 {
                          tunnel: w1883 -> [w1891 w1895 w1897]
                          tunnel: [w1890 w1895 w1896] -> w1880
                          frame 0, Default {
                            n1034 = Array Size(array=w1891) -> (size(s)=w1892:i32)
                            n1035 = for {
                              N: w1892 -> [_]
                              tunnel: w1891 -> [w1894] mode=indexing
                              tunnel: [w1893] -> w1890 mode=indexing
                              n1036 = formula code="y=1000000./(x*x);"("x"=w1894) -> ("y"=w1893:dbl)
                            }
                          }
                          frame 1 {
                          }
                          frame 2 {
                            n1037 = Divide(x=w1897, y=1000.0) -> (x/y=w1896:dbl[])
                          }
                        }
                        n1038 = property on="Review Graph" class="XYGraph (strict)"("YScale.Minimum"=w1889) -> ()  [unwired: 2 in, 2 out]
                        n1039 = Bundle(w1881, w1880) -> (w1879:cluster{dbl[], dbl[]})  [unwired: 1 in]
                      }
                    }
                    n1040 = local write "Review Graph"(w1871) -> ()
                  }
                  frame 2 {
                    n1041 = local read "Review Graph"() -> (w1904:cluster{dbl[], dbl[]})
                    n1042 = local read "Review Iscale"() -> (w1899:u16)
                    n1043 = Not Equal?(x=w1899, y=w1903) -> (x != y?=w1905:bool)
                    n1044 = case shown="True" w1905 {
                      tunnel: w1904 -> [w1906 w1913]
                      tunnel: [w1907 w1908] -> w1900
                      tunnel: w1902 -> [_ w1915]
                      tunnel: [w1906 w1909] -> w1901
                      tunnel: w1899 -> [w1907 w1908]
                      frame False {
                      }
                      frame True {
                        n1045 = local read "LCS Data"() -> (w1916:cluster{dbl[], dbl[], dbl[], dbl[], dbl[]}[])
                        n1046 = call "TestData.vi"("Test No."=w1915, "Array No."=u32 1, "Data IN"=w1916) -> ("Array OUT"=w1918:dbl[])  [unwired: 7 in, 1 out]
                        n1047 = Unbundle(w1913) -> (w1912:dbl[])  [unwired: 1 out]
                        n1048 = Absolute Value(x=w1918) -> (abs(x)=w1917:dbl[])
                        n1049 = property on="Review Graph" class="XYGraph (strict)"() -> ("YScale.Mapping Mode"=w1919:u8)  [unwired: 2 in, 2 out]
                        n1050 = case shown="2" w1908 {
                          tunnel: w1917 -> [w1921 w1923 w1927]
                          tunnel: [w1921 w1922 w1926] -> w1910
                          tunnel: w1912 -> [w1920 w1925 w1929]
                          tunnel: [w1920 w1925 w1929] -> w1911
                          frame 0, Default {
                          }
                          frame 1 {
                            n1051 = Divide(x=w1923, y=1000.0) -> (x/y=w1922:dbl[])
                          }
                          frame 2 {
                            n1052 = Divide(x=w1927, y=1000000.0) -> (x/y=w1926:dbl[])
                          }
                        }
                        n1053 = property on="Review Graph" class="XYGraph (strict)"("YScale.Minimum"=w1919) -> ()  [unwired: 2 in, 2 out]
                        n1054 = Bundle(w1911, w1910) -> (w1909:cluster{dbl[], dbl[]})  [unwired: 1 in]
                      }
                    }
                    n1055 = local write "Review Graph"(w1901) -> ()
                  }
                  frame 3 {
                  }
                }
                n1056 = local read "Review Scales"() -> (w1825:u16)
                n1057 = Not Equal?(x=w1825, y=w1828) -> (x != y?=w1824:bool)
                n1058 = case shown="False" w1824 {
                  tunnel: w1825 -> [w1829 w1830]
                  tunnel: [w1829 w1830] -> w1823
                  frame False {
                  }
                  frame True {
                    n1059 = case shown="..0" w1830 {
                      tunnel: [w1833 1 0 w1838] -> w1832
                      tunnel: [w1833 0 1 w1838] -> w1831
                      frame ..0 {
                        w1833 = 0
                      }
                      frame 1 {
                      }
                      frame 2 {
                      }
                      frame 3.. {
                        w1838 = 1
                      }
                    }
                    n1060 = property on="Review Graph" class="XYGraph (strict)"("X Scale.Mapping Mode"=w1832) -> ()  [unwired: 2 in, 2 out]
                    n1061 = property on="Review Graph" class="XYGraph (strict)"("Y Scale.Mapping Mode"=w1831, "YScale.Minimum"=w1831) -> ()  [unwired: 2 in, 2 out]
                  }
                }
              }
              frame #2 {
                # "Check if user wants to save the comment."
                n1062 = case shown="True" "Write Comments" {
                  frame False {
                  }
                  frame True {
                    n1063 = flat-sequence {
                      tunnel: [w1941] -> w1937
                      tunnel: [w1938] -> w1936
                      tunnel: w1937 -> [w2066]
                      tunnel: w1936 -> [w2065]
                      frame #0 {
                        # "Write text."
                        n1064 = local read "Current Text"() -> (w1947:string)
                        n1065 = xnode "Match Regular Expression"("input string"=w1947, "regular expression"="Comments: " ("input string")) -> ("before match"=w1945:string, "whole match"=w1944:string, "after match"=w1939:string)  [unwired: 4 in, 2 out]
                        n1066 = local read "Data Path"() -> (w1941:path)
                        n1067 = Concatenate Strings("Comment Box", " " ("string"), w1939) -> (w1943:string)
                        n1068 = Concatenate Strings(w1945, w1944, w1943) -> (w1942:string)
                        n1069 = Write to Text File(file (use dialog)=w1941, text=w1942) -> (error out=w1938:errorcluster)  [unwired: 2 in, 2 out]
                      }
                      frame #1 {
                        # "Re-display text and clear comment box."
                        n1070 = Read from Text File(file (use dialog)=w2066, error in=w2065) -> (text=w2064:string)  [unwired: 2 in, 3 out]
                        n1071 = local write "Current Text"(w2064) -> ()
                        n1072 = local write "Comment Box"("" ("Comment Box")) -> ()
                      }
                    }
                  }
                }
              }
            }
          }
        }
      }
    }
  }
